vi "main 1.17 beta.vi"() -> ()   [LabVIEW 2015]
uses:
  subvi/PHOIBOS/DEFINITIONS/DEF_dev_state.ctl
  subvi/PHOIBOS/DEFINITIONS/DEF_dev_type.ctl
  <vilib>/Analysis/_algsub.llb/Real Vector Norm.vi
  <vilib>/Analysis/1siggen.llb/Ramp Pattern by Samples.vi
  <vilib>/DAQmx/create/channels.llb/DAQmx Create Channel (DI-Digital Input).vi
  <userlib>/caLab/Private/Put_DBL_PV.vi
  <vilib>/Utility/file.llb/Write Delimited Spreadsheet (string).vi
  <vilib>/Utility/file.llb/Read Delimited Spreadsheet (string).vi
  <vilib>/Utility/file.llb/Write Delimited Spreadsheet (DBL).vi
  <userlib>/caLab/Private/Get_PV.vi
  subvi/Newport ESP301/Newport ESP301.lvlib
  subvi/sp_manip.llb/sp_manip_lib.lvlib
  subvi/sp_manip.llb/tcp_gateway.lvlib
  <vilib>/Analysis/NI_AALBase.lvlib
  <vilib>/Analysis/NI_AALPro.lvlib
  subvi/ZaberTSeries/ZaberTSeries.lvlib
panel:
  out "Pics L":i32=200
  out "Waveform Chart":dbl(graph)
  out "G2 X":cluster{dbl[], "Ramp Pattern":dbl[]}(graph)
  in  "reset every n pics":bool=TRUE
  in  "pics2avg":i32=50
  in  "abort acq.":bool
  out "G2 Y":cluster{dbl[], "Ramp Pattern":dbl[]}(graph)
  out "ETA":timestamp=timestamp(3655133644.4615793 s since 1904-01-01) format="%<%H:%M:%S>T"
  out "acq. imgs":i32=200
  out "snap_prog":dbl(slide)=1.0 scale=0.0..1.0
  in  "BasePath":path=path "X:/trARPES/PESData"
  in  "cam_liveavg":bool=TRUE caption="live average"
  out "cam_fps":dbl=19.774122625512067 caption="FPS" format="%.1g"
  out "sideimg":dbl[][](graph)
  out "RunNumber":u16=3067
  out "sum":dbl format="%#.2g"
  out "max":dbl
  out "mainimg":dbl[][](graph)
  out "ESP_con?":bool=TRUE caption="ESP301"
  out "phoib_con?":bool caption="PHOIBOS"
  out "manip_con?":bool=TRUE caption="manipulator"
  out "cam_con?":bool caption="camera"
  in  "main_close":bool
  in  "Tab Control":enum32{"live", "scan", "devices"}(tab)=enum."devices"
  out "Readback":dbl=304.0
  out "In Range":bool=TRUE
  in  "setpoint_set":bool
  in  "Setpoint":dbl=302.0
  out "TB":dbl=302.67
  out "TA":dbl=303.83
  in  "phoib_I_10s":dbl
  out "phoib_I_10":dbl caption="Mesh Back"
  in  "mirr_go":bool
  in  "ESP_opent0file":bool
  in  "mirr_rel":i32=1 caption="relative [steps]"
  in  "mirr_Y-":bool
  in  "mirr_Y+":bool
  in  "mirr_X+":bool
  in  "mirr_X-":bool
  in  "manip_deltas":dbl[](array[numeric])=[0.0, 0.0, 5.0, 0.0, 0.0, 0.0] caption="delta" format="%#.5g"
  in  "aq.mode":enum32{"Radio Selection 1", "Radio Selection 2"}(radio)=enum."Radio Selection 2"
  in  "dark avg":i32=100
  in  "cam_avgs":i32=200 caption="N"
  in  "ESP_delta":dbl caption="relative [mm]"
  in  "ESP_-":bool
  in  "ESP_+":bool
  in  "ESP_go":bool
  in  "ESP_dest_t":dbl=-1194159.4608093842 caption="[fs]"
  in  "ESP_dest":dbl=-324.0 caption="[mm]"
  in  "ESP_set_t0":bool
  in  "phoib_I_6s":dbl=3200.0
  in  "phoib_I_5s":dbl=1500.0
  in  "phoib_I_4s":dbl=4.558
  in  "phoib_I_3s":dbl=-10.0
  in  "phoib_I_2s":dbl=35.0
  in  "phoib_I_1s":dbl=21.0
  in  "phoib_standby":bool
  in  "phoib_set":bool
  out "phoib_I_6":dbl caption="Screen Voltage"
  out "phoib_I_5":dbl caption="Detctor Voltage"
  out "phoib_I_4":dbl caption="Work Function"
  out "phoib_I_3":dbl caption="Coil Current"
  out "phoib_I_2":dbl caption="Pass Energy"
  out "phoib_I_1":dbl caption="Kinetic Energy"
  out "Saved Positions":string[][](table)=[["ertwertwert", "-2.299945", "-2.030214", "38.900024", "50.000762", "0.000887", "-97.998082"], ["uztgugt", "-14.999451", "-13.638894", "442.380066", "13.998380", "-1.893758", "-76.305838"], ["asdf", "-14.999451", "-13.638894", "442.380066", "13.998380", "-1.893758", "-76.305838"], ["test3", "-14.999451", "-13.638894", "441.380066", "13.998380", "-1.893758", "-76.305838"]]
  in  "Save Pos":bool
  in  "Load":bool
  in  "Delete":bool
  in  "ManipRel +":bool
  in  "ManipRel -":bool
  in  "Move Abs":bool
  in  "stop manip":bool
  in  "dest":dbl[](array[numeric])=[1.794011231344732, -4.007411134769244, 35.099853515625, 337.9843004481455, 2.0, 140.61656469713384] caption="destination" format="%#.5g"
  out "axis":string[](array[string])=["x", "y", "z", "polar", "tilt", "azimut"]
  out "pos":dbl[](array[numeric])=[1.794011231344732, -4.007411134769244, 35.099853515625, 337.9843004481455, 1.998632949125299, 140.61656469713384] caption="position" format="%.5f"
  in  "ana_mode":T1(ring)=enum."WideAngleMode"
  in  "ana_voltrange":enum16{"3.5kV", "1.5kV", "400V", "100V", "10V"}(ring)=enum."400V"
  out "ESP_pos":dbl=-325.0 caption="Position"
  out "ESP_delay":dbl=-1200830.742713347 caption="Delay"
  out "ESP_t0":dbl=-145.0 caption="Time Zero @"
  out "phoib_I_7":dbl caption="Conversion Voltage"
  in  "phoib_I_7s":dbl=-30.0
  in  "phoib_I_8s":dbl=0.0039
  in  "phoib_I_9s":dbl
  out "phoib_I_8":dbl caption="FD1"
  out "phoib_I_9":dbl caption="Mesh Front"
  in  "gain":bool
  in  "cam_exp":u32=50 caption="exposure [ms]"
  in  "binning":u16(ring)=2 items=["X 1", "X 2", "X 4", "X 8"]
  in  "cam_dark?":bool=TRUE caption="subtract dark?"
  in  "cam_dark":bool
  in  "cam_saveimg":bool
  in  "e-size":u8
  in  "lower threshold":i32=50
  in  "count?":bool
  in  "ROI Left":i32=1
  in  "ROI Right":i32=43
  in  "ROI Top":i32=1
  in  "ROI Bottom":i32=33
  out "moving?":bool[](array[boolean])
  out "mirr_posX":i32=60782 caption="X"
  out "mirr_posY":i32=121383 caption="Y"
  in  "mirr_dest":i32[](array[numeric])=[60782, 121383]
  out "waveplate position":dbl format="%.6g"
  out "stage2 position":dbl format="%.6g"
  out "current scan 2":i32=3
  out "scan 1":dbl(slide)=1.0 scale=0.0..1.0
  in  "Tab Control 2":enum32{"setup", "data"}(tab)
  in  "scan_selector 2":T2(tab)=enum."stage2"
  in  "scan_manip_start 2":dbl[](array[numeric])=[1.794011231344732, -4.007411134769244, 35.099853515625, 337.9843004481455, 2.000390761745462, 140.61656469713384] caption="start position" format="%#.5g"
  in  "scan_manip_deltas 2":dbl[](array[numeric])=[0.0, 0.0, 0.0, 0.0, 1.0, 0.0] caption="direction vector\n(gets normalized)" format="%#.5g"
  in  "scan_manip_setstart 2":bool
  in  "scan_mirr_start 2":i32[](array[numeric])=[60782, 121383] caption="scan_mirr_start"
  in  "scan_mirr_deltas 2":i32[](array[numeric])=[1, 0] caption="direction vector\n(gets normalized)"
  in  "scan_mirr_setstart 2":bool
  in  "wait addional  2":dbl caption="s"
  in  "Wait for T 2":bool=TRUE
  in  "scan_volt_parameter 2":string(combo)="Kinetic Energy"
  in  "waypointsD2":string[][](table)=[["302", "1"], ["304", ""], ["", ""]]
  in  "waypointsD1":string[][](table)=[["302", "1"], ["304", ""], ["", ""]]
  in  "load waypoints 1":bool
  in  "meas_iter":i32=1 caption="Iterations"
  in  "scan_selector":T2(tab)=enum."stage2"
  in  "scan_manip_setstart":bool
  in  "scan_manip_start":dbl[](array[numeric])=[1.794011231344732, -4.007411134769244, 35.099853515625, 337.9843004481455, 2.000390761745462, 140.61656469713384] caption="start position" format="%#.5g"
  in  "scan_manip_deltas":dbl[](array[numeric])=[0.0, 0.0, 0.0, 0.0, 1.0, 0.0] caption="direction vector\n(gets normalized)" format="%#.5g"
  in  "scan_mirr_start":i32[](array[numeric])=[60782, 121383]
  in  "scan_mirr_deltas":i32[](array[numeric])=[1, 0] caption="direction vector\n(gets normalized)"
  in  "scan_mirr_setstart":bool
  in  "wait addional":dbl caption="s"
  in  "Wait for T":bool=TRUE
  in  "scan_volt_parameter":string(combo)="Kinetic Energy"
  in  "clear waypoints 1":bool
  in  "load waypoints 2":bool
  in  "clear waypoints 2":bool
  out "intensitygraph":cluster{"Array":dbl[], "Intensity Chart":dbl[]}(graph)={"Array"=[302.0, 303.0, 304.0], "Intensity Chart"=[1937.88, 12704.590000000002, 4640.840000000001]}
  out "energygraph":dbl[][](graph)=[[0.0, 0.0, 0.0, 64.28999999999999, 120.06, 0.0, 0.0, 0.0, 0.0, 0.0, 0.0, 0.0, 0.0, 0.0, 0.0, 0.0, 0.0, 0.0, 0.0, 0.0, 0.0, 0.0, 0.0, 0.0, 0.0, 0.0, 0.0, 0.0, 0.0, 0.0, 0.0, 0.0, 0.0, 0.0, 0.0, 0.0, 0.0, 0.0, 0.0, 0.0, 0.0, 0.0, 0.0, 0.0, 0.0, 0.0, 0.0, 0.0, 0.0, 384.53999999999996, 1103.3799999999999, 448.21000000000004, 0.0, 0.0, 0.0, 0.0, 0.0, 0.0, 0.0, 0.0, 0.0, 0.0, 0.0, 0.0, 0.0, 0.0, 0.0, 0.0, 0.0, 120.82, 0.0, 261.04, 195.1, 253.87, 199.70999999999998, 127.75, 87.50999999999999, 0.0, 52.54, 0.0, 0.0, 51.78, 55.73, 0.0, 0.0, 0.0, 0.0, 0.0, 0.0, 0.0, 0.0, 0.0, 0.0, 0.0, 0.0, 0.0, 0.0, 0.0, 0.0, 0.0, 0.0, 0.0, 0.0, 0.0, 0.0, 0.0, 0.0, 0.0, 0.0, 0.0, 0.0, 0.0, 0.0, 332.90999999999997, 1106.25, 934.74, 0.0, 156.76, 62.65, 0.0, 0.0, 0.0, 0.0, 0.0, 0.0, 54.62, 0.0, 0.0, 0.0, 0.0, 0.0, 0.0, 0.0, 0.0, 0.0, 0.0, 0.0, 0.0, 0.0, 0.0, 0.0, 0.0, 0.0, 0.0, 65.85, 165.75, 0.0, 0.0, 0.0, 0.0, 0.0, 0.0, 0.0, 0.0, 0.0, 0.0, 0.0, 0.0, 0.0, 0.0, 0.0, 0.0, 0.0, 266.63, 591.5, 261.64, 0.0, 391.9, 527.29, 82.87, 123.75, 286.74, 151.72, 0.0, 0.0, 0.0, 0.0, 0.0, 0.0, 0.0, 0.0, 0.0, 0.0, 0.0, 0.0, 0.0, 0.0, 0.0, 0.0, 0.0, 0.0, 0.0, 396.37, 721.0900000000001, 353.5, 83.97999999999999, 104.77000000000001, 0.0, 57.83, 60.98, 182.28, 128.78, 0.0, 0.0, 0.0, 465.25, 624.3399999999999, 348.62, 0.0, 0.0, 0.0, 0.0, 0.0, 0.0, 0.0, 0.0, 0.0, 0.0, 0.0, 0.0, 119.7, 217.91, 120.56, 0.0, 0.0, 0.0, 0.0, 0.0, 0.0, 0.0, 58.89, 0.0, 0.0, 0.0, 202.23999999999998, 149.79000000000002, 0.0, 117.82, 212.51999999999998, 534.74, 421.98, 50.97, 0.0, 0.0, 0.0, 0.0, 362.15999999999997, 656.04, 265.02, 0.0, 0.0, 0.0, 0.0, 0.0, 0.0, 0.0, 0.0, 0.0, 0.0, 0.0, 0.0, 0.0, 0.0, 0.0, 0.0, 0.0, 0.0, 0.0, 0.0, 0.0, 0.0, 0.0, 0.0, 0.0, 0.0, 0.0, 0.0, 0.0, 0.0, 0.0, 0.0, 0.0, 0.0, 0.0, 0.0, 0.0, 0.0, 0.0, 0.0, 0.0, 0.0, 0.0, 0.0, 0.0, 0.0, 0.0, 0.0, 0.0, 0.0, 0.0, 0.0, 0.0, 0.0, 0.0, 0.0, 0.0, 0.0, 0.0, 0.0, 0.0, 0.0, 0.0, 0.0, 237.67999999999998, 286.08, 130.9, 0.0, 0.0, 0.0, 0.0, 0.0, 0.0, 0.0, 0.0, 0.0, 0.0, 0.0, 0.0, 0.0, 0.0, 0.0, 0.0, 0.0, 0.0, 0.0, 0.0, 0.0, 0.0, 0.0, 0.0, 0.0, 0.0, 0.0, 0.0], [0.0, 0.0, 0.0, 0.0, 0.0, 0.0, 0.0, 0.0, 0.0, 0.0, 0.0, 0.0, 0.0, 0.0, 0.0, 0.0, 0.0, 485.13, 1279.2, 234.71, 0.0, 0.0, 0.0, 0.0, 0.0, 0.0, 0.0, 0.0, 0.0, 0.0, 0.0, 0.0, 50.5, 654.4200000000001, 511.98, 0.0, 0.0, 0.0, 0.0, 0.0, 0.0, 0.0, 0.0, 0.0, 0.0, 0.0, 0.0, 0.0, 0.0, 0.0, 0.0, 0.0, 0.0, 0.0, 0.0, 0.0, 0.0, 0.0, 63.72, 693.84, 574.54, 0.0, 0.0, 0.0, 68.68, 1054.28, 1010.9499999999999, 0.0, 0.0, 0.0, 0.0, 0.0, 0.0, 0.0, 0.0, 0.0, 0.0, 0.0, 56.57, 971.76, 1333.73, 330.0, 0.0, 0.0, 0.0, 0.0, 0.0, 349.33000000000004, 292.7, 0.0, 0.0, 0.0, 0.0, 0.0, 0.0, 82.77000000000001, 1059.23, 1069.87, 156.47, 0.0, 0.0, 0.0, 0.0, 293.91, 333.47, 551.4, 493.64, 73.72999999999999, 0.0, 0.0, 0.0, 0.0, 0.0, 0.0, 0.0, 0.0, 0.0, 0.0, 0.0, 0.0, 0.0, 0.0, 286.01, 543.0699999999999, 251.94, 0.0, 0.0, 0.0, 0.0, 0.0, 233.63, 968.4799999999999, 771.53, 109.94, 0.0, 123.07, 499.72999999999996, 431.4, 0.0, 0.0, 60.85, 69.5, 0.0, 0.0, 0.0, 0.0, 0.0, 0.0, 0.0, 0.0, 0.0, 0.0, 0.0, 0.0, 0.0, 0.0, 52.01, 0.0, 0.0, 0.0, 0.0, 0.0, 0.0, 0.0, 0.0, 0.0, 0.0, 0.0, 0.0, 0.0, 0.0, 0.0, 0.0, 0.0, 0.0, 0.0, 0.0, 0.0, 0.0, 0.0, 0.0, 0.0, 0.0, 0.0, 0.0, 0.0, 0.0, 0.0, 0.0, 0.0, 52.95, 478.8, 870.47, 572.83, 61.67, 268.19, 1143.4, 1804.2599999999998, 1145.6100000000001, 739.22, 904.59, 1109.3000000000002, 1233.6599999999999, 212.92, 0.0, 0.0, 105.95, 448.76000000000005, 1306.3500000000001, 1005.5900000000001, 68.8, 0.0, 57.94, 0.0, 0.0, 0.0, 0.0, 0.0, 0.0, 0.0, 0.0, 0.0, 0.0, 0.0, 0.0, 0.0, 0.0, 0.0, 0.0, 0.0, 0.0, 0.0, 0.0, 0.0, 0.0, 0.0, 0.0, 159.01, 520.94, 925.5600000000001, 1641.53, 2261.26, 1259.83, 0.0, 0.0, 0.0, 0.0, 0.0, 0.0, 136.69, 398.81, 382.02, 0.0, 0.0, 0.0, 0.0, 0.0, 0.0, 421.01, 1376.5800000000002, 1425.75, 268.07, 0.0, 345.84000000000003, 396.77, 0.0, 0.0, 0.0, 0.0, 0.0, 216.93, 727.65, 830.9, 774.2299999999999, 839.3900000000001, 309.97, 0.0, 0.0, 0.0, 0.0, 0.0, 0.0, 0.0, 100.57, 459.66, 305.86, 0.0, 0.0, 0.0, 0.0, 0.0, 0.0, 0.0, 0.0, 0.0, 0.0, 0.0, 0.0, 0.0, 0.0, 0.0, 0.0, 0.0, 0.0, 0.0, 0.0, 0.0, 0.0, 0.0, 0.0, 0.0, 64.97999999999999, 379.62, 337.15999999999997, 83.6, 463.66, 399.03999999999996, 0.0, 0.0, 0.0, 0.0, 0.0, 0.0, 0.0, 0.0, 0.0, 0.0, 0.0, 0.0, 0.0, 0.0, 0.0, 0.0, 0.0, 0.0, 0.0, 0.0, 0.0, 0.0, 0.0, 0.0, 0.0, 0.0, 0.0], [0.0, 0.0, 0.0, 0.0, 0.0, 0.0, 0.0, 0.0, 0.0, 0.0, 0.0, 0.0, 0.0, 0.0, 0.0, 165.83, 124.99, 78.27000000000001, 0.0, 0.0, 0.0, 765.77, 1457.88, 293.67, 0.0, 0.0, 0.0, 0.0, 0.0, 0.0, 0.0, 0.0, 0.0, 0.0, 0.0, 0.0, 0.0, 0.0, 0.0, 0.0, 0.0, 0.0, 0.0, 0.0, 0.0, 0.0, 0.0, 0.0, 0.0, 85.5, 116.32, 0.0, 0.0, 0.0, 0.0, 0.0, 0.0, 0.0, 0.0, 0.0, 0.0, 0.0, 0.0, 0.0, 0.0, 0.0, 0.0, 0.0, 179.01, 123.78999999999999, 64.69, 0.0, 433.57000000000005, 1457.15, 661.49, 0.0, 0.0, 0.0, 0.0, 0.0, 0.0, 171.38, 497.28999999999996, 835.47, 1797.0300000000002, 1202.25, 169.95, 0.0, 0.0, 0.0, 0.0, 383.74, 496.08, 196.89999999999998, 0.0, 0.0, 0.0, 0.0, 719.08, 1717.5100000000002, 1360.8, 163.65, 118.56, 798.75, 610.32, 0.0, 0.0, 0.0, 0.0, 73.12, 51.75, 0.0, 0.0, 0.0, 0.0, 0.0, 0.0, 0.0, 0.0, 0.0, 0.0, 0.0, 233.35000000000002, 1128.3, 1138.8400000000001, 207.43, 0.0, 0.0, 50.52, 0.0, 0.0, 0.0, 0.0, 0.0, 0.0, 0.0, 0.0, 0.0, 0.0, 0.0, 0.0, 0.0, 0.0, 0.0, 0.0, 0.0, 0.0, 0.0, 0.0, 0.0, 0.0, 122.82, 66.93, 184.87, 606.35, 1065.2, 616.33, 82.97, 0.0, 0.0, 0.0, 0.0, 0.0, 0.0, 0.0, 0.0, 0.0, 0.0, 0.0, 210.77, 369.49, 0.0, 0.0, 0.0, 0.0, 0.0, 0.0, 0.0, 0.0, 0.0, 0.0, 0.0, 0.0, 0.0, 0.0, 0.0, 0.0, 0.0, 0.0, 61.71, 492.70000000000005, 501.67999999999995, 50.9, 0.0, 0.0, 0.0, 0.0, 0.0, 0.0, 0.0, 0.0, 0.0, 0.0, 0.0, 0.0, 0.0, 0.0, 0.0, 0.0, 0.0, 0.0, 0.0, 0.0, 0.0, 0.0, 0.0, 0.0, 0.0, 0.0, 0.0, 0.0, 0.0, 0.0, 0.0, 0.0, 0.0, 0.0, 0.0, 0.0, 0.0, 0.0, 0.0, 0.0, 0.0, 0.0, 0.0, 0.0, 0.0, 0.0, 0.0, 0.0, 0.0, 0.0, 0.0, 0.0, 0.0, 0.0, 0.0, 0.0, 0.0, 0.0, 0.0, 0.0, 0.0, 0.0, 0.0, 0.0, 0.0, 0.0, 0.0, 0.0, 0.0, 0.0, 0.0, 0.0, 0.0, 0.0, 0.0, 0.0, 0.0, 191.69, 347.02, 262.31, 325.89, 168.79, 0.0, 0.0, 52.9, 53.13, 0.0, 0.0, 0.0, 0.0, 0.0, 0.0, 0.0, 0.0, 0.0, 0.0, 0.0, 0.0, 0.0, 0.0, 0.0, 0.0, 0.0, 0.0, 0.0, 0.0, 0.0, 0.0, 0.0, 0.0, 0.0, 0.0, 327.12, 491.83000000000004, 242.02999999999997, 0.0, 0.0, 0.0, 0.0, 0.0, 0.0, 0.0, 676.6, 975.77, 229.86, 0.0, 144.15, 151.75, 0.0, 0.0, 0.0, 0.0, 0.0, 0.0, 0.0, 0.0, 0.0, 0.0, 0.0, 0.0, 0.0, 0.0, 0.0, 0.0, 0.0, 0.0, 0.0, 0.0, 0.0, 0.0, 0.0]]
  out "anglegraph":dbl[][](graph)=[[0.0, 0.0, 0.0, 0.0, 0.0, 0.0, 0.0, 0.0, 0.0, 0.0, 0.0, 0.0, 0.0, 0.0, 0.0, 0.0, 0.0, 0.0, 0.0, 0.0, 0.0, 0.0, 0.0, 0.0, 0.0, 0.0, 0.0, 307.98, 204.45, 0.0, 0.0, 0.0, 0.0, 0.0, 0.0, 0.0, 0.0, 0.0, 0.0, 0.0, 0.0, 0.0, 0.0, 0.0, 0.0, 0.0, 0.0, 0.0, 0.0, 0.0, 0.0, 0.0, 0.0, 0.0, 0.0, 0.0, 0.0, 0.0, 0.0, 0.0, 0.0, 0.0, 0.0, 0.0, 0.0, 0.0, 0.0, 0.0, 0.0, 0.0, 0.0, 0.0, 0.0, 0.0, 0.0, 0.0, 0.0, 0.0, 0.0, 0.0, 0.0, 0.0, 0.0, 0.0, 0.0, 0.0, 0.0, 0.0, 0.0, 0.0, 0.0, 0.0, 0.0, 0.0, 0.0, 0.0, 0.0, 0.0, 0.0, 0.0, 0.0, 0.0, 0.0, 0.0, 0.0, 0.0, 0.0, 0.0, 0.0, 0.0, 0.0, 0.0, 0.0, 0.0, 0.0, 0.0, 0.0, 0.0, 0.0, 0.0, 0.0, 0.0, 0.0, 0.0, 0.0, 0.0, 0.0, 0.0, 0.0, 0.0, 0.0, 0.0, 0.0, 0.0, 0.0, 0.0, 0.0, 0.0, 0.0, 0.0, 0.0, 0.0, 0.0, 0.0, 0.0, 0.0, 0.0, 0.0, 0.0, 0.0, 0.0, 0.0, 0.0, 0.0, 0.0, 0.0, 640.8800000000001, 550.45, 91.89, 0.0, 0.0, 0.0, 0.0, 0.0, 0.0, 0.0, 0.0, 0.0, 0.0, 0.0, 0.0, 0.0, 0.0, 0.0, 0.0, 69.94, 60.96, 0.0, 0.0, 0.0, 0.0, 0.0, 0.0, 0.0, 0.0, 0.0, 0.0, 0.0, 0.0, 0.0, 0.0, 0.0, 0.0, 0.0, 0.0, 0.0, 115.87, 235.84, 172.04999999999998, 0.0, 0.0, 0.0, 0.0, 0.0, 0.0, 0.0, 0.0, 0.0, 0.0, 0.0, 0.0, 0.0, 0.0, 0.0, 0.0, 0.0, 0.0, 0.0, 0.0, 0.0, 0.0, 0.0, 0.0, 0.0, 0.0, 0.0, 0.0, 0.0, 0.0, 0.0, 0.0, 0.0, 0.0, 0.0, 0.0, 0.0, 0.0, 0.0, 0.0, 0.0, 0.0, 0.0, 0.0, 0.0, 0.0, 0.0, 0.0, 0.0, 0.0, 0.0, 0.0, 0.0, 0.0, 0.0, 0.0, 0.0], [0.0, 0.0, 0.0, 0.0, 0.0, 0.0, 0.0, 0.0, 0.0, 0.0, 0.0, 0.0, 0.0, 0.0, 0.0, 0.0, 54.97, 1426.6399999999999, 1312.94, 180.81, 0.0, 0.0, 0.0, 0.0, 0.0, 0.0, 0.0, 465.48, 989.61, 293.56, 0.0, 0.0, 0.0, 0.0, 0.0, 0.0, 0.0, 0.0, 0.0, 0.0, 0.0, 0.0, 0.0, 0.0, 0.0, 0.0, 0.0, 0.0, 0.0, 0.0, 0.0, 0.0, 0.0, 0.0, 0.0, 0.0, 0.0, 0.0, 0.0, 331.78, 944.91, 463.28, 0.0, 0.0, 0.0, 0.0, 143.70999999999998, 402.81, 196.09, 0.0, 0.0, 0.0, 483.82, 433.7, 0.0, 0.0, 0.0, 0.0, 0.0, 0.0, 89.85, 513.2, 263.03999999999996, 0.0, 0.0, 0.0, 0.0, 0.0, 0.0, 0.0, 0.0, 104.84, 0.0, 226.86, 214.93, 235.13, 0.0, 0.0, 0.0, 0.0, 0.0, 0.0, 0.0, 0.0, 0.0, 0.0, 0.0, 0.0, 0.0, 0.0, 0.0, 0.0, 0.0, 0.0, 0.0, 0.0, 0.0, 0.0, 0.0, 0.0, 0.0, 0.0, 0.0, 0.0, 0.0, 0.0, 0.0, 0.0, 0.0, 0.0, 0.0, 0.0, 0.0, 0.0, 0.0, 0.0, 0.0, 0.0, 0.0, 380.83, 649.96, 229.04, 0.0, 0.0, 0.0, 276.21000000000004, 441.79999999999995, 228.29, 0.0, 0.0, 0.0, 0.0, 0.0, 0.0, 0.0, 0.0, 0.0, 0.0, 0.0, 0.0, 0.0, 0.0, 0.0, 0.0, 0.0, 0.0, 0.0, 0.0, 123.92000000000002, 1311.81, 1454.81, 600.87, 0.0, 0.0, 0.0, 0.0, 0.0, 0.0, 0.0, 0.0, 0.0, 0.0, 0.0, 0.0, 0.0, 0.0, 0.0, 0.0, 0.0, 0.0, 0.0, 0.0, 0.0, 0.0, 0.0, 0.0, 0.0, 0.0, 0.0, 0.0, 0.0, 0.0, 654.53, 894.22, 410.35, 0.0, 0.0, 0.0, 0.0, 0.0, 0.0, 0.0, 0.0, 0.0, 0.0, 0.0, 0.0, 0.0, 0.0, 0.0, 0.0, 0.0, 0.0, 0.0, 0.0, 0.0, 0.0, 0.0, 0.0, 0.0, 0.0, 0.0, 0.0, 0.0, 0.0, 0.0, 0.0, 0.0, 0.0, 0.0, 0.0, 0.0, 0.0, 0.0, 0.0, 0.0, 0.0, 0.0, 0.0, 0.0, 0.0, 0.0, 0.0, 0.0, 0.0, 0.0], [0.0, 0.0, 0.0, 0.0, 0.0, 0.0, 0.0, 0.0, 0.0, 0.0, 0.0, 0.0, 0.0, 0.0, 0.0, 0.0, 0.0, 0.0, 0.0, 0.0, 0.0, 0.0, 0.0, 0.0, 0.0, 0.0, 0.0, 0.0, 0.0, 125.9, 1017.51, 504.48, 0.0, 0.0, 0.0, 0.0, 0.0, 0.0, 0.0, 0.0, 0.0, 0.0, 0.0, 0.0, 0.0, 0.0, 0.0, 0.0, 0.0, 0.0, 0.0, 0.0, 0.0, 0.0, 0.0, 0.0, 0.0, 0.0, 0.0, 0.0, 0.0, 0.0, 0.0, 0.0, 0.0, 0.0, 0.0, 0.0, 0.0, 0.0, 0.0, 0.0, 109.81, 66.88, 0.0, 0.0, 733.48, 806.32, 342.43, 0.0, 0.0, 0.0, 0.0, 0.0, 0.0, 0.0, 0.0, 0.0, 0.0, 0.0, 0.0, 0.0, 0.0, 0.0, 0.0, 0.0, 0.0, 0.0, 0.0, 0.0, 0.0, 0.0, 0.0, 0.0, 0.0, 174.07999999999998, 275.74, 429.21, 301.15999999999997, 0.0, 0.0, 0.0, 0.0, 0.0, 0.0, 0.0, 0.0, 0.0, 0.0, 0.0, 0.0, 0.0, 0.0, 0.0, 0.0, 0.0, 0.0, 0.0, 0.0, 0.0, 0.0, 0.0, 0.0, 0.0, 0.0, 0.0, 0.0, 0.0, 0.0, 0.0, 0.0, 0.0, 0.0, 0.0, 0.0, 0.0, 0.0, 0.0, 0.0, 0.0, 0.0, 0.0, 0.0, 0.0, 0.0, 0.0, 0.0, 0.0, 0.0, 0.0, 0.0, 0.0, 0.0, 0.0, 0.0, 0.0, 0.0, 0.0, 0.0, 0.0, 0.0, 0.0, 0.0, 0.0, 0.0, 252.98000000000002, 303.56, 60.91, 52.9, 53.13, 0.0, 0.0, 0.0, 0.0, 0.0, 0.0, 0.0, 0.0, 0.0, 0.0, 0.0, 0.0, 0.0, 0.0, 0.0, 0.0, 0.0, 0.0, 0.0, 0.0, 0.0, 0.0, 0.0, 0.0, 0.0, 0.0, 0.0, 0.0, 0.0, 0.0, 0.0, 0.0, 0.0, 61.05, 350.49, 266.71000000000004, 0.0, 0.0, 0.0, 0.0, 0.0, 0.0, 0.0, 0.0, 0.0, 0.0, 0.0, 0.0, 0.0, 0.0, 0.0, 0.0, 0.0, 0.0, 0.0, 0.0, 0.0, 0.0, 0.0, 0.0, 0.0, 0.0, 0.0, 0.0, 0.0, 0.0, 0.0, 0.0, 0.0, 0.0, 0.0, 0.0, 0.0, 0.0, 0.0, 0.0]]
  in  "stop after iteration":bool
  in  "time/step [s]":dbl=10.787117004394531
  out "current iteration":i32=1
  out "current scan":i32=3
  out "iteration":dbl(slide)=1.0 scale=0.0..1.0
  out "scan 2":dbl(slide)=1.0 scale=0.0..1.0
  in  "stop after step":bool
  in  "scan_go":bool
  out "measpoints":i32=3
  out "total steps":i32=3
  out "RAM [MB]":dbl=1.6590000000000003
  out "disk [MB]":dbl=1.6590000000000003
  out "duration [HH:MM:SS]":dbl=32.361351013183594 format="%<%H:%M:%S>t"
  out "ETA 2":timestamp
  in  "ESP patch":i32[](array[numeric])=[3, 2, 1]
  in  "LS310  EPICS Heater":string="trARPES:Carving:HT-RNG"
  in  "LS310  EPICS SP":string="trARPES:Carving:TEMP"
  in  "LS310  EPICS chanel B":string="trARPES:Carving:TEMP-B"
  in  "mm/s":dbl
  in  "Set Speed to":bool
  in  "ESP Axis waveplate":i32=2 min=1 max=3
  in  "mirr_init":bool
  in  "mirr_release":bool
  in  "mirr_Y#":u8=2
  in  "manip_init":bool
  in  "manip_release":bool
  in  "phoib_init":bool
  in  "phoib_release":bool
  in  "ESP_init":bool
  in  "ESP_release":bool
  in  "ESP301 VISA":refnum<visa-resource-name>="COM4"
  in  "board number":i32
  in  "cam_init":bool
  in  "cam_release":bool
  out "cam_error":errorcluster
  out "phoib_error":errorcluster
  out "state":T3 items=["Off"=-1, "Standby"=0, "On"=1]
  in  "ESP Axis delay":i32=3 min=1 max=3
  out "error out":errorcluster={"status"=FALSE, "code"=1073676418, "source"="VISA Close in Newport ESP301.lvlib:Close.vi->main 1.16 testing LR.vi"}
  out "error out 2":errorcluster={"status"=TRUE, "code"=1, "source"="TCP Write in sp_manip_lib.lvlib:sp_manip_disconnect.vi->main 1.16 testing LR.vi"}
  out "mirr_Error":errorcluster={"status"=FALSE, "code"=1073676418, "source"="VISA Close in ZaberTSeries.lvlib:Close.vi->main 1.16 testing LR.vi"}
  in  "mirr_VISA":refnum<visa-resource-name>="COM7"
  in  "mirr_X#":u8=1
  in  "Operating mode\nHP & QE / HS & DiCam Pro":u32=1
  in  "Frame trigger \n(High Performance and QE only)":u16
  in  "LS310  EPICS chanel A":string="trARPES:Carving:TEMP_RBV"
  in  "Status EPICS chanel":string="trARPES:Carving:TEMP-STAT"
  # "camera"
  # "analyzer"
  # "manipulator"
  # "temperature"
  # "aquisition"
  # "delay stage"
  # "mirror"
  # "Position"
  # "Destination"
  # "- no settings -"
  # "waypoints are absolute values"
  # "- no settings -"
  # "waypoints are absolute values"
  # "- no settings -"
  # "waypoints are absolute values"
  # "X\nY\nZ\npolar\ntilt\nazimut"
  # "waypoint \"0\" is start position"
  # "X\nY"
  # "waypoint \"0\" is start position"
  # "waypoints are absolute values"
  # "- no settings -"
  # "waypoints are absolute values"
  # "- no settings -"
  # "waypoints are absolute values"
  # "- no settings -"
  # "waypoints are absolute values"
  # "X\nY\nZ\npolar\ntilt\nazimut"
  # "waypoint \"0\" is start position"
  # "X\nY"
  # "waypoint \"0\" is start position"
  # "waypoints are absolute values"
  # "camera"
  # "phoibos"
  # "ESP301"
  # "manipulator"
  # "mirror"
  # "delay"
  # "waveplate"
  # "stage2"
  # "0 = sequential\n1 = simultaneous"
  # "0 = internal\n1 = external rising\n2 = external falling"
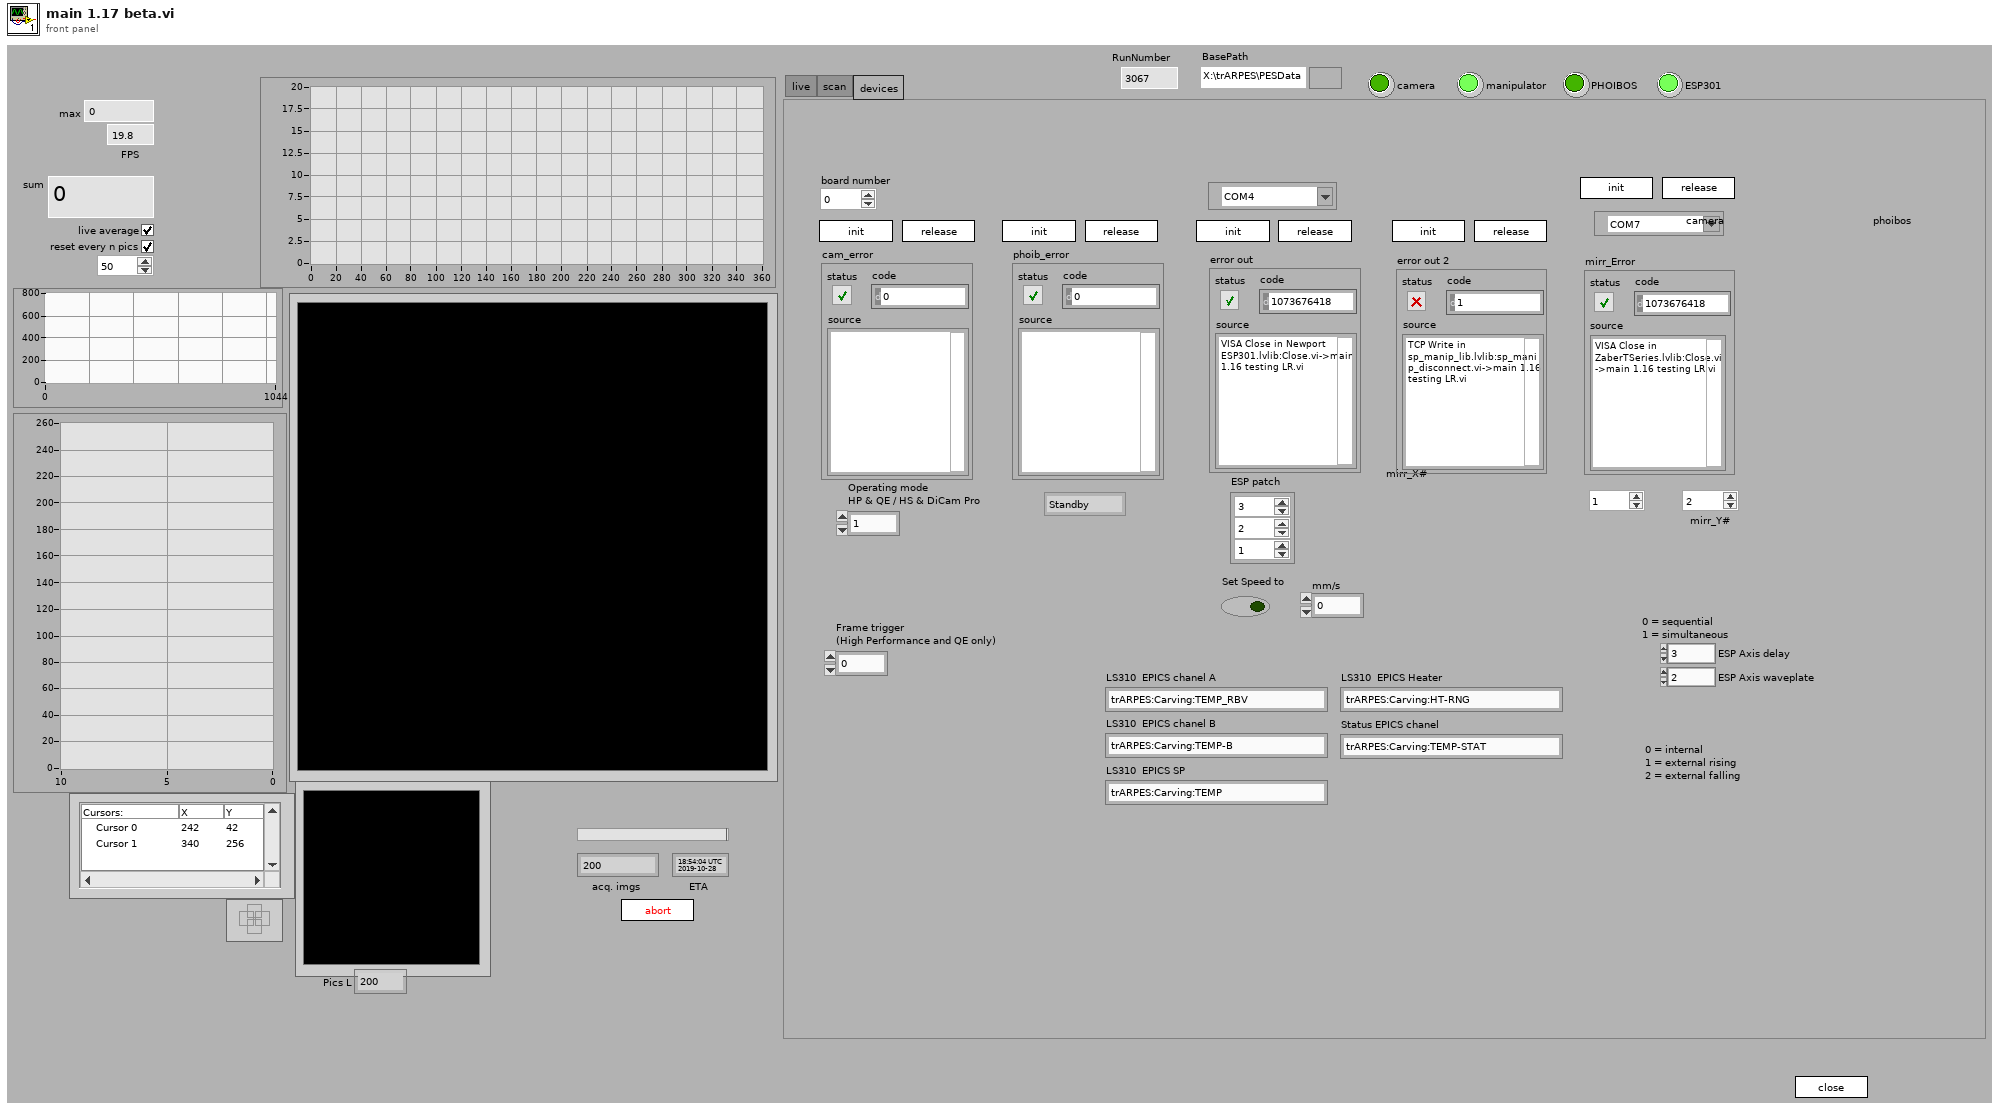
[diagram p1: front panel]
types:
  T1 = enum16{"HighMagnification", "MediumMagnification", "LowMagnification", "HighAngularDispersion", "MediumAngularDispersion", "LowAngularDispersion", "WideAngleMode", "LargeArea", "MediumArea", "SmallArea", "HighMagnification2", "SmallArea2"}
  T2 = enum32{"none", "delay", "waveplate", "stage2", "manipulator", "mirror", "temperature", "voltage"}
  T3 = typedef "DEF_dev_state.ctl" = i32
  T4 = cluster{"queue out":refnum<queue>, "queue out":refnum<queue>, "queue out":refnum<queue>, "queue out":refnum<queue>, "queue out":refnum<queue>, "queue out":refnum<queue>}
  T5 = typedef "LVCursorListTypeDef.ctl" = cluster{"Name":string, "Color":u32, "Style":u8, "Point Style":u8, "Name Visible":bool, "Allow Drag":bool, "Cursor Mode":u32, "Plot":i32, "Index":i32, "Position":cluster{"X":dbl, "Y":dbl}, "X Scale":u32, "Y Scale":u32, "Watch Plots":i32[], "Watch All Plots":bool, "Plot Area":i32, "Label Offset":cluster{"X":dbl, "Y":dbl}}[]
  T6 = cluster{"mirr_X#":u8, "Command":u8, dbl, "Response Count":i32}
  T7 = cluster{"mirr_Y#":u8, "Command":u8, dbl, "Response Count":i32}
  T8 = cluster{i32, "Command":u8, i32, "Response Count":i32}
  T9 = cluster{"Axis_Name":string, "Axis_Type":string, "Axis_Position":dbl, "continous":bool, "moving":bool}[]
  T10 = typedef "DEF_dev_type.ctl" = enum32{"devA (analyzer)", "devD (detector)"}
  T11 = cluster{"Camera type":u32, "Operating mode\nHP & QE / HS & DiCam Pro ":u32, "Frame trigger \n(High Performance and QE only)":u16, "Sequence trigger":u16, "Low Light\n(QE only)":bool, "Gain":bool, "Horzontal\nbinning":u16, "Vertical\nbinning ":u16, "ROI Left":i32, "ROI Right":i32, "ROI Top":i32, "ROI Bottom":i32}
  T12 = cluster{"Name":string, "Color":u32, "Style":u8, "Point Style":u8, "Name Visible":bool, "Allow Drag":bool, "Cursor Mode":u32, "Plot":i32, "Index":i32, "Position":cluster{"X":dbl, "Y":dbl}, "X Scale":u32, "Y Scale":u32, "Watch Plots":i32[], "Watch All Plots":bool, "Plot Area":i32, "Label Offset":cluster{"X":dbl, "Y":dbl}}
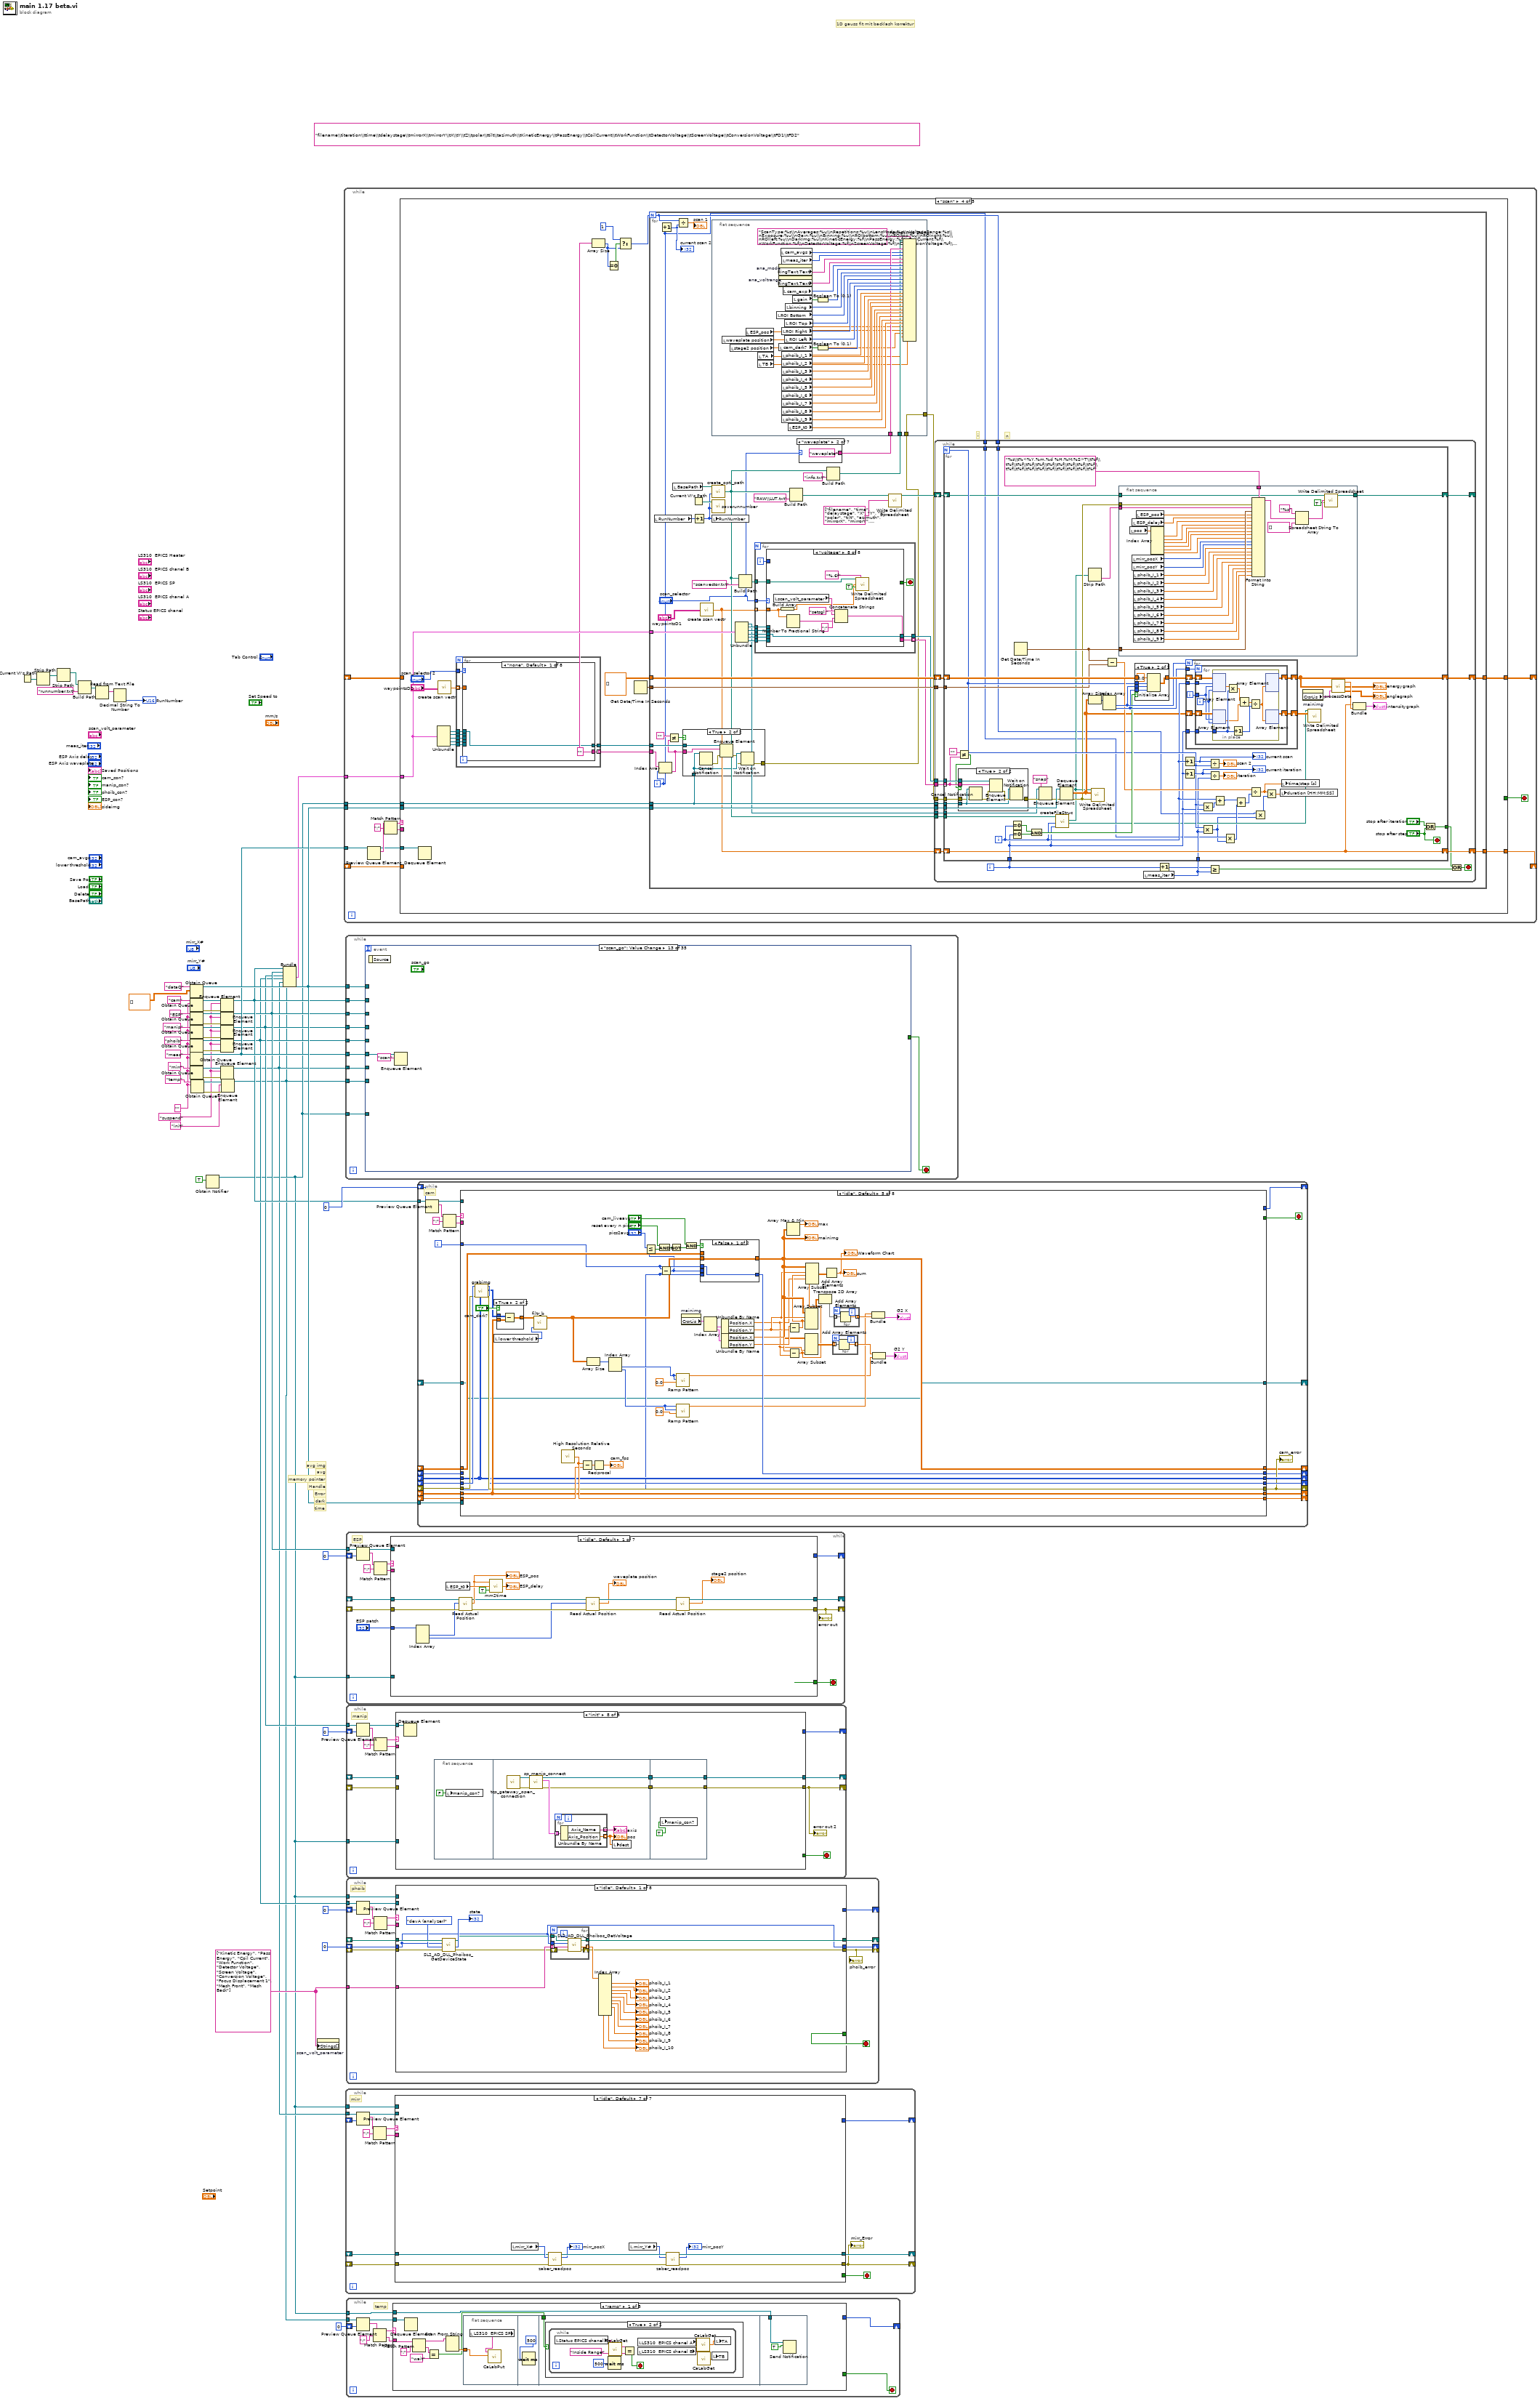
[diagram p0: block diagram]
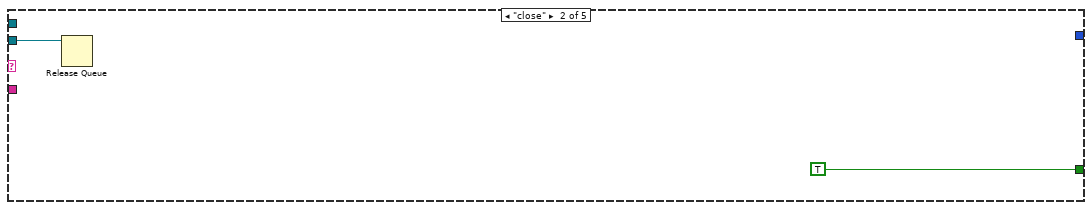
[diagram p3: hidden frame]
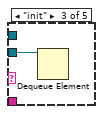
[diagram p4: hidden frame]
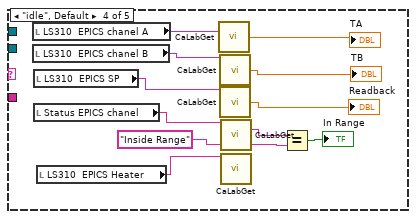
[diagram p5: hidden frame]
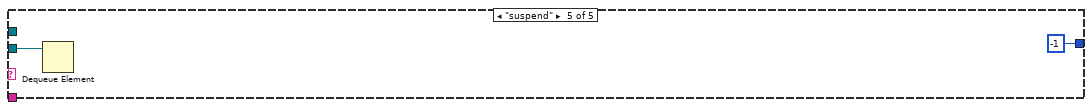
[diagram p6: hidden frame]
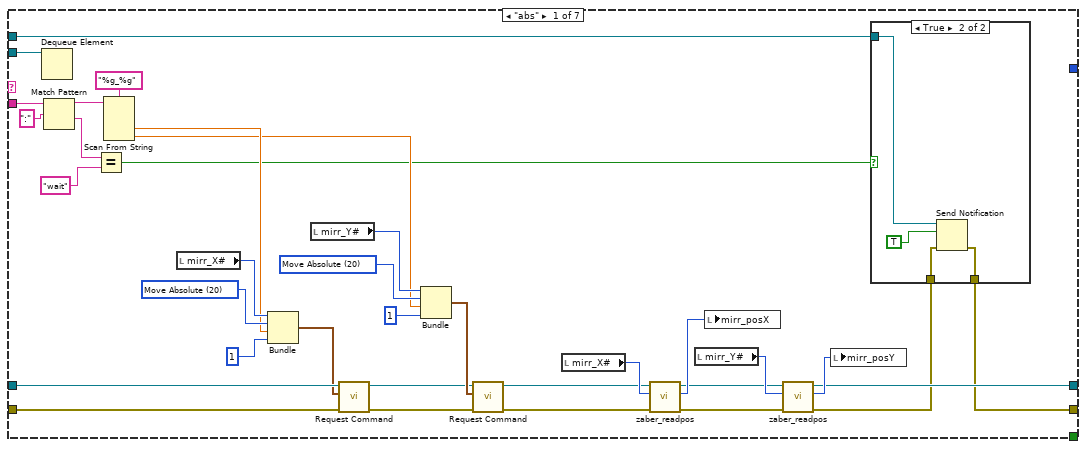
[diagram p7: hidden frame]
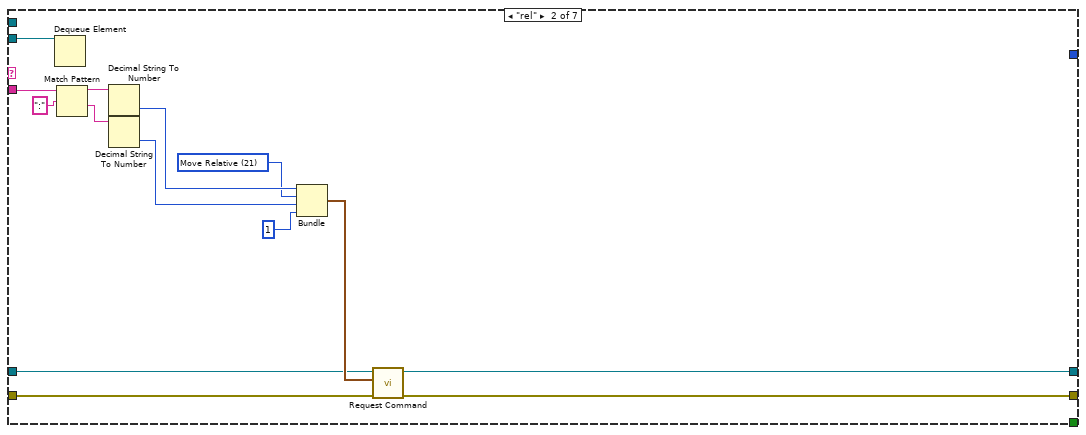
[diagram p9: hidden frame]
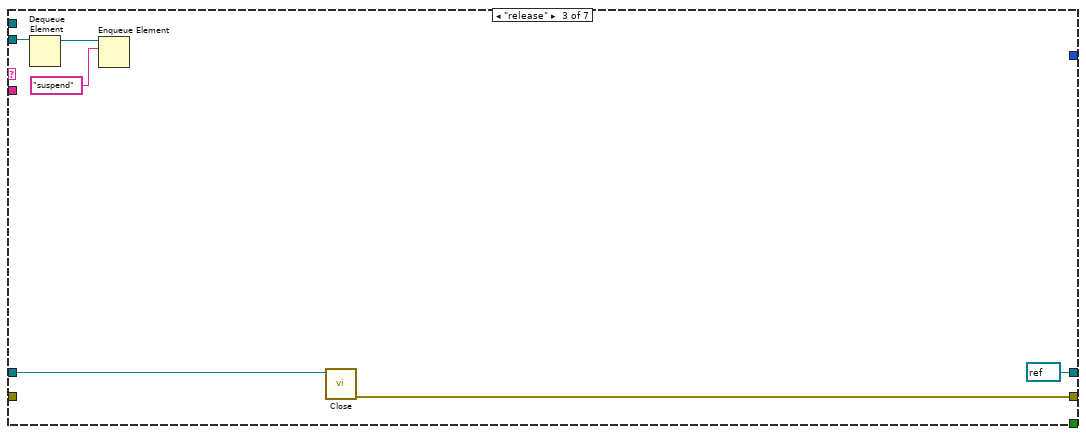
[diagram p10: hidden frame]
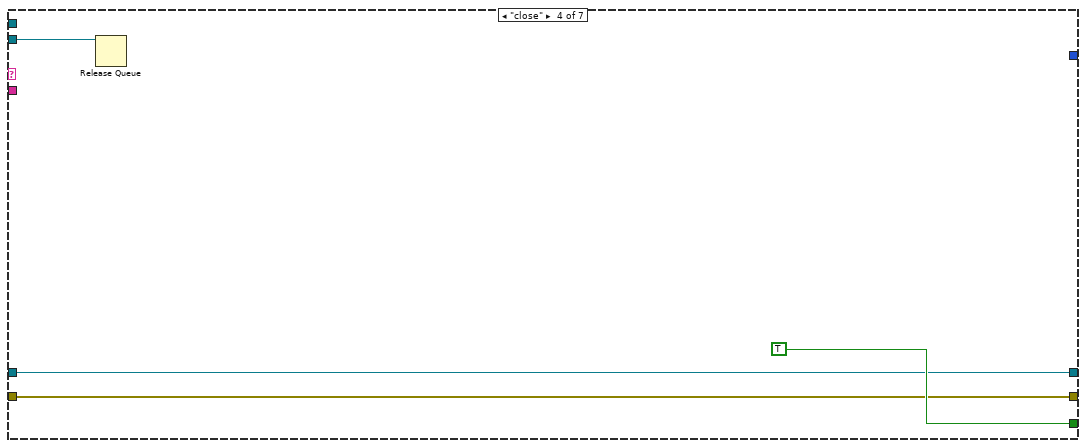
[diagram p11: hidden frame]
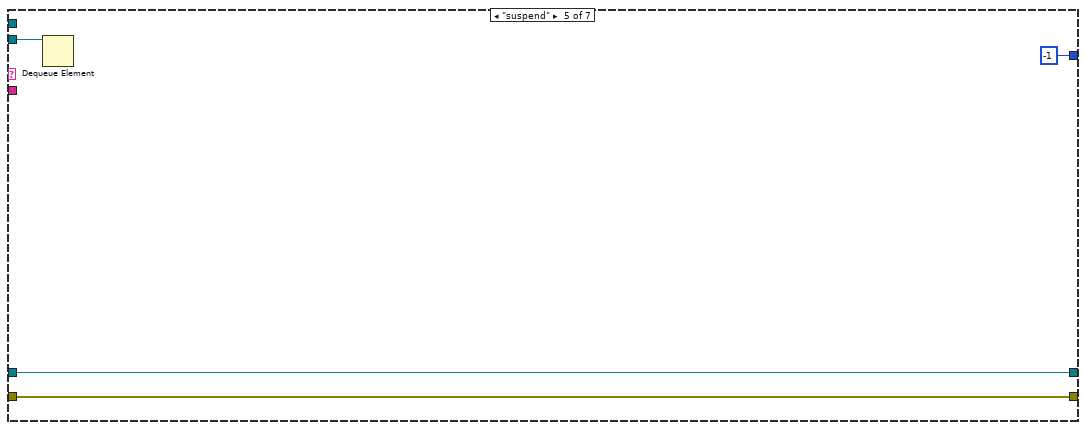
[diagram p12: hidden frame]
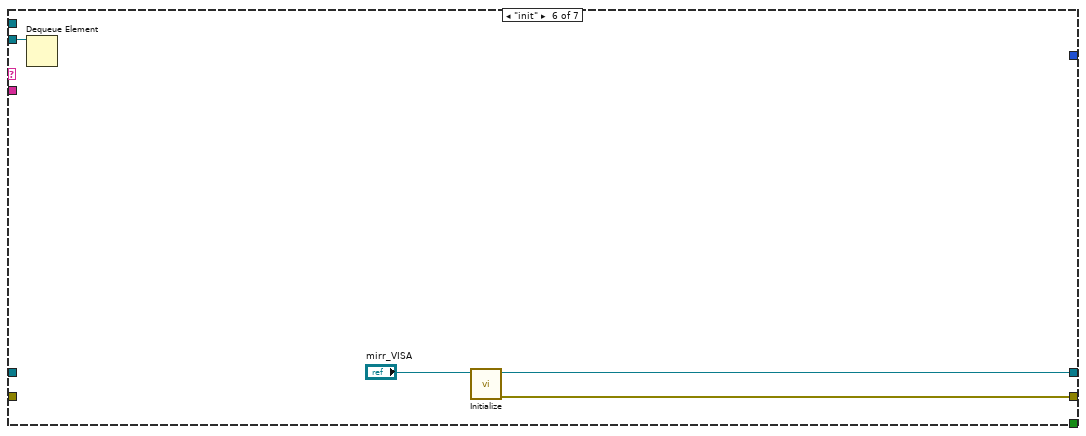
[diagram p13: hidden frame]
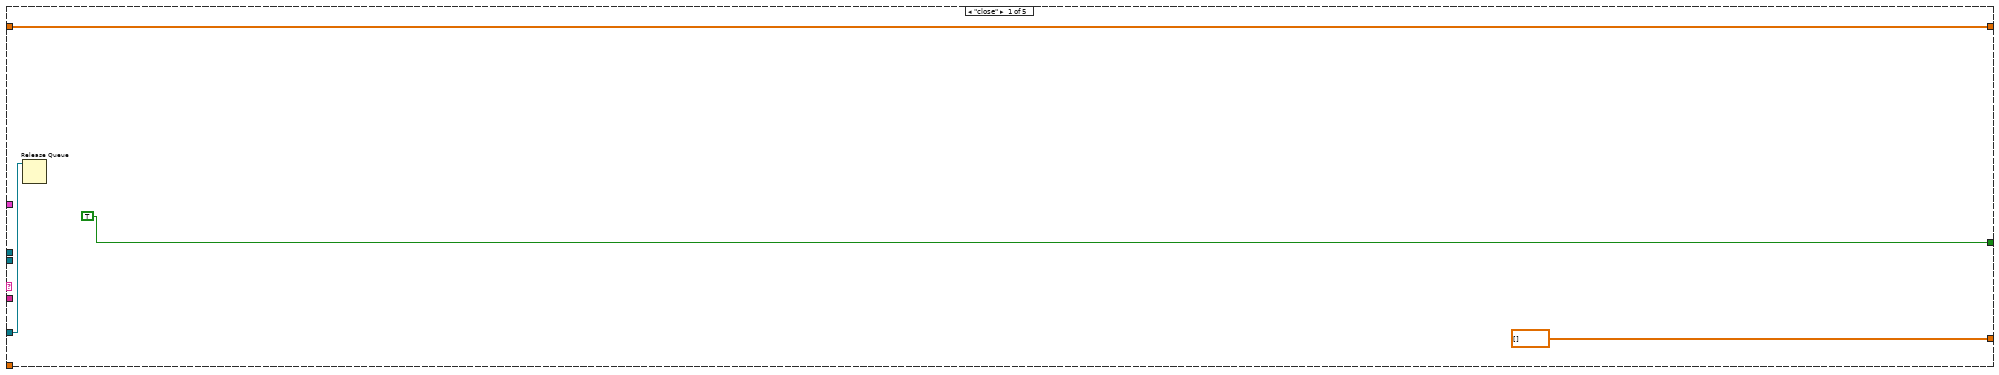
[diagram p14: hidden frame]
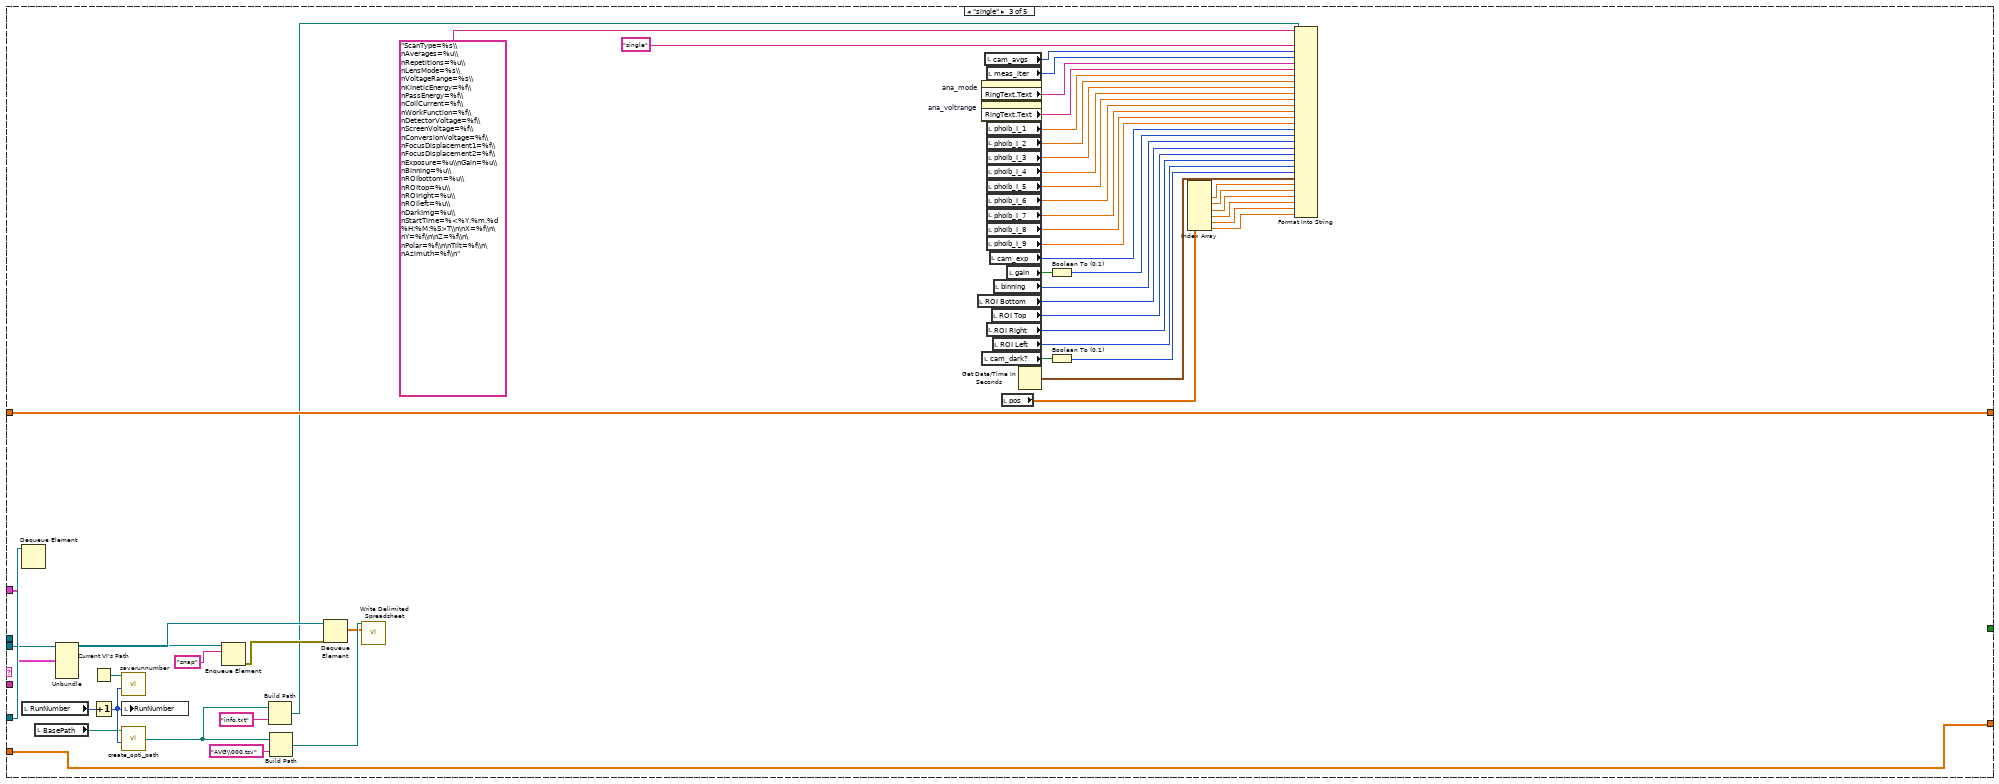
[diagram p16: hidden frame]
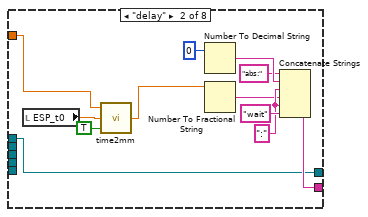
[diagram p17: hidden frame]
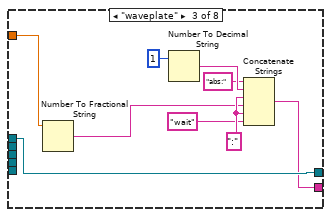
[diagram p18: hidden frame]
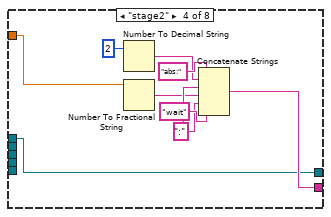
[diagram p19: hidden frame]
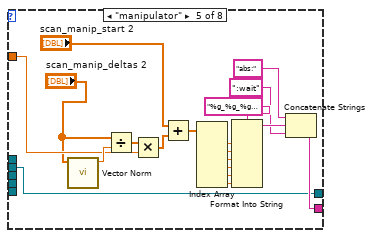
[diagram p20: hidden frame]
diagram:
  (unwired) "filename\\titeration\\ttime\\tdelaystage\\tmirrorX\\tmirrorY\\tX\\tY\\tZ\\tpolar\\ttilt\\tazimuth\\tKineticEnergy\\tPassEnergy\\tCoilCurrent\\tWorkFunction\\tDetectorVoltage\\tScreenVoltage\\tConversionVoltage\\tFD1\\tFD2"
  w15 = string[] ["Kinetic Energy", "Pass Energy", "Coil Current", "Work Function", "Detector Voltage", "Screen Voltage", "Conversion Voltage", "Focus Displacement 1", "Mesh Front", "Mesh Back"]
  w3 = "suspend" ("name (unnamed)")
  w8 = "" ("name (unnamed)")
  # "1D gauss fit mit backlash korrektur"
  # "avg img"
  # "avg"
  # "time"
  # "dark"
  # "Error"
  # "Handle"
  # "memory pointer"
  n1 = Current VI's Path() -> (path=w23:path)
  n2 = Strip Path(path=w23) -> (stripped path=w27:path)  [unwired: 1 out]
  n3 = Strip Path(path=w27) -> (stripped path=w28:path)  [unwired: 1 out]
  n4 = Build Path(base path=w28, name or relative path="runnumber.txt") -> (appended path=w25:path)
  n5 = Read from Text File(file (use dialog)=w25) -> (text=w26:string)  [unwired: 3 in, 3 out]
  n6 = Decimal String To Number(string=w26) -> (number=→"RunNumber":i32)  [unwired: 2 in, 1 out]
  n7 = Obtain Queue(name (unnamed)="dataQ", element data type=dbl[][] []) -> (queue out=w29:refnum<queue>)  [unwired: 3 in, 2 out]
  n8 = Obtain Queue(name (unnamed)="cam", element data type=w8) -> (queue out=w48:refnum<queue>, error out=w47:errorcluster)  [unwired: 3 in, 1 out]
  n9 = Obtain Queue(name (unnamed)="ESP", element data type=w8) -> (queue out=w45:refnum<queue>, error out=w46:errorcluster)  [unwired: 3 in, 1 out]
  n10 = Obtain Queue(name (unnamed)="manip", element data type=w8) -> (queue out=w42:refnum<queue>, error out=w41:errorcluster)  [unwired: 3 in, 1 out]
  n11 = Obtain Queue(name (unnamed)="phoib", element data type=w8) -> (queue out=w39:refnum<queue>, error out=w40:errorcluster)  [unwired: 3 in, 1 out]
  n12 = Obtain Queue(name (unnamed)="meas", element data type=w8) -> (queue out=w22:refnum<queue>)  [unwired: 3 in, 2 out]
  n13 = Obtain Queue(name (unnamed)="mirr", element data type=w8) -> (queue out=w13:refnum<queue>, error out=w12:errorcluster)  [unwired: 3 in, 1 out]
  n14 = Obtain Queue(name (unnamed)="temp", element data type=w8) -> (queue out=w7:refnum<queue>, error out=w6:errorcluster)  [unwired: 3 in, 1 out]
  n15 = Obtain Notifier(notification data type=TRUE) -> (notifier out=w5:refnum<notifier>)  [unwired: 3 in, 2 out]
  n16 = Enqueue Element(queue=w48, element=w3, error in (no error)=w47) -> (queue out=w20:refnum<queue>)  [unwired: 1 in, 2 out]
  n17 = Enqueue Element(queue=w45, element=w3, error in (no error)=w46) -> (queue out=w19:refnum<queue>)  [unwired: 1 in, 2 out]
  n18 = Enqueue Element(queue=w42, element=w3, error in (no error)=w41) -> (queue out=w18:refnum<queue>)  [unwired: 1 in, 2 out]
  n19 = Enqueue Element(queue=w39, element=w3, error in (no error)=w40) -> (queue out=w17:refnum<queue>)  [unwired: 1 in, 2 out]
  n20 = Enqueue Element(queue=w13, element=w3, error in (no error)=w12) -> (queue out=w10:refnum<queue>)  [unwired: 1 in, 2 out]
  n21 = Enqueue Element(queue=w7, element="init" ("name (unnamed)"), error in (no error)=w6) -> (queue out=w1:refnum<queue>)  [unwired: 1 in, 2 out]
  n22 = Bundle("queue out"=w20, "queue out"=w19, "queue out"=w18, "queue out"=w17, "queue out"=w10, "queue out"=w1) -> (w21:T4)  [unwired: 1 in]
  n23 = property on="scan_volt_parameter" class="CmbBox"("Strings[]"=w15) -> ()  [unwired: 2 in, 2 out]
  n24 = while {
    tunnel: w29 -> [w63]
    tunnel: w22 -> [w60]
    tunnel: w21 -> [w56]
    shift-right: [w54] -> _
    shift-left: _ -> [w53]
    tunnel: w5 -> [w52]
    shift-right: [w51] -> _
    shift-left: _ -> [w50]
    stop <- w55 stop-if-true
    n25 = Preview Queue Element(queue=w60) -> (queue out=w57:refnum<queue>, element=w62:string)  [unwired: 2 in, 2 out]
    n26 = Match Pattern(string=w62, regular expression=":") -> (before substring=w59:string, after substring=w58:string)  [unwired: 1 in, 2 out]
    n27 = case shown="\"scan\"" w59 {
      tunnel: w63 -> [_ _ w119 w142 _]
      tunnel: w58 -> [_ _ _ _ _]
      tunnel: w57 -> [w67 _ w120 w138 w601]
      tunnel: [TRUE _ _ _ _] -> w55
      tunnel: w56 -> [_ _ w107 w135 _]
      tunnel: [w65 w69 w105 w140 w607] -> w54
      tunnel: w53 -> [w65 w69 w105 _ w607]
      tunnel: w52 -> [_ _ _ w139 _]
      tunnel: [dbl[] [] ("Array") w68 w77 w136 w603] -> w51
      tunnel: w50 -> [_ w68 w77 _ w603]
      frame "close" {
        n28 = Release Queue(queue=w67) -> ()  [unwired: 2 in, 3 out]
      }
      frame "idle", Default {
      }
      frame "single" {
        n29 = Dequeue Element(queue=w120) -> ()  [unwired: 2 in, 4 out]
        n30 = local read "RunNumber"() -> (w114:u16)
        n31 = local read "BasePath"() -> (w115:path)
        n32 = Unbundle(w107) -> ("queue out"=w106:refnum<queue>)  [unwired: 5 out]
        n33 = Increment(x=w114) -> (x+1=w116:u16)
        n34 = Current VI's Path() -> (path=w113:path)
        n35 = call "saverunnumber.vi"("RunNumber"=w116, "VI path"=w113) -> ()  [unwired: 10 in]
        n36 = local write "RunNumber"(w116) -> ()
        n37 = call "create_opti_path.vi"("RunNumber"=w116, "base path"=w115) -> ("Path"=w109:path)  [unwired: 2 in]
        n38 = Enqueue Element(queue=w106, element="snap" ("string")) -> (error out=w117:errorcluster)  [unwired: 2 in, 2 out]
        n39 = Build Path(base path=w109, name or relative path="info.txt") -> (appended path=w78:path)
        n40 = Build Path(base path=w109, name or relative path="AVG\\000.tsv") -> (appended path=w111:path)
        n41 = Dequeue Element(queue=w119, error in (no error)=w117) -> (element=w108:dbl[][])  [unwired: 1 in, 3 out]
        n42 = call-poly <vilib>:"Write Delimited Spreadsheet.vi"("file path (dialog if empty)"=w111, "2D data"=w108) -> ()  [unwired: 12 in, 2 out]
        n43 = local read "ROI Bottom"() -> (w85:i32)
        n44 = property on="ana_mode" class="Enum (strict)"() -> ("RingText.Text"=w100:string)  [unwired: 2 in, 2 out]
        n45 = property on="ana_voltrange" class="Enum (strict)"() -> ("RingText.Text"=w99:string)  [unwired: 2 in, 2 out]
        n46 = local read "cam_dark?"() -> (w81:bool)
        n47 = local read "cam_avgs"() -> (w102:i32)
        n48 = local read "meas_iter"() -> (w101:i32)
        n49 = local read "phoib_I_1"() -> (w98:dbl)
        n50 = local read "phoib_I_2"() -> (w97:dbl)
        n51 = local read "phoib_I_3"() -> (w96:dbl)
        n52 = local read "phoib_I_4"() -> (w95:dbl)
        n53 = local read "phoib_I_5"() -> (w94:dbl)
        n54 = local read "phoib_I_6"() -> (w93:dbl)
        n55 = local read "phoib_I_7"() -> (w92:dbl)
        n56 = local read "phoib_I_8"() -> (w91:dbl)
        n57 = local read "phoib_I_9"() -> (w90:dbl)
        n58 = local read "ROI Right"() -> (w83:i32)
        n59 = local read "cam_exp"() -> (w89:u32)
        n60 = local read "ROI Top"() -> (w84:i32)
        n61 = local read "ROI Left"() -> (w82:i32)
        n62 = local read "binning"() -> (w86:u16)
        n63 = local read "pos"() -> (w76:dbl[])
        n64 = local read "gain"() -> (w88:bool)
        n65 = Get Date/Time In Seconds() -> (seconds since 1Jan1904=w79:timestamp)
        n66 = Boolean To (0,1)(Boolean=w88) -> (0, 1=w87:i16)
        n67 = Boolean To (0,1)(Boolean=w81) -> (0, 1=w80:i16)
        n68 = Index Array(array=w76) -> (element #1=w75:dbl, element #2=w74:dbl, element #3=w73:dbl, element #4=w72:dbl, element #5=w71:dbl, element #6=w70:dbl)  [unwired: 6 in]
        n69 = Format Into String(format string="ScanType=%s\\nAverages=%u\\nRepetitions=%u\\nLensMode=%s\\nVoltageRange=%s\\nKineticEnergy=%f\\nPassEnergy=%f\\nCoilCurrent=%f\\nWorkFunction=%f\\nDetectorVoltage=%f\\nScreenVoltage=%f\\nConversionVoltage=%f\\nFocusDisplacement1=%f\\nFocusDisplacement2=%f\\nExposure=%u\\nGain=%u\\nBinning=%u\\nROIbottom=%u\\nROItop=%u\\nROIright=%u\\nROIleft=%u\\nDarkImg=%u\\nStartTime=%<%Y.%m.%d %H:%M:%S>T\\n\nX=%f\\n\nY=%f\\n\nZ=%f\\n\nPolar=%f\\n\nTilt=%f\\n\nAzimuth=%f\\n", initial string=w78, "single" ("input 1"), w102, w101, w100, w99, w98, w97, w96, w95, w94, w93, w92, w91, w90, w89, w87, w86, w85, w84, w83, w82, w80, w79, w75, w74, w73, w72, w71, w70) -> ()  [unwired: 1 in, 2 out]
      }
      frame "scan" {
        n70 = Dequeue Element(queue=w138) -> ()  [unwired: 2 in, 4 out]
        n71 = Unbundle(w135) -> ("queue out"=w134:refnum<queue>, "queue out"=w133:refnum<queue>, "queue out"=w132:refnum<queue>, "queue out"=w131:refnum<queue>, "queue out"=w130:refnum<queue>)  [unwired: 1 out]
        n72 = call "create scan vectr.vi"("Table Control"="waypointsD2") -> ("Array"=w128:dbl[])
        n73 = for {
          tunnel: "scan_selector 2" -> [w151]
          tunnel: w134 -> [w150]
          tunnel: w133 -> [w149]
          tunnel: w132 -> [w148]
          tunnel: w131 -> [w147]
          tunnel: w130 -> [w146]
          tunnel: [w145] -> w125 mode=indexing
          tunnel: [w144] -> w129
          tunnel: w128 -> [w143] mode=indexing
          n74 = case shown="\"none\", Default" w151 {
            tunnel: ["" w155 w166 w176 w187 w205 w219 w231] -> w145
            tunnel: w150 -> [w152 w154 w168 w175 _ _ _ _]
            tunnel: w149 -> [_ _ _ _ w186 _ _ _]
            tunnel: w148 -> [_ _ _ _ _ _ _ w230]
            tunnel: w147 -> [_ _ _ _ _ w204 _ _]
            tunnel: w146 -> [_ _ _ _ _ _ w218 _]
            tunnel: [w152 w154 w168 w175 w186 w204 w218 w230] -> w144
            tunnel: w143 -> [_ w156 w167 w177 w188 w203 w221 w232]
            frame "none", Default {
            }
            frame "delay" {
              w159 = ":" ("string")
              n75 = local read "ESP_t0"() -> (w163:dbl)
              n76 = call "time2mm.vi"("fs[1]/ps[0]"=TRUE, "Offset (mm)"=w163, "time"=w156) -> ("position (mm)"=w164:dbl)
              n77 = Number To Decimal String(number=0) -> (decimal integer string=w161:string)  [unwired: 1 in]
              n78 = Number To Fractional String(number=w164) -> (F-format string=w157:string)  [unwired: 3 in]
              n79 = Concatenate Strings("abs:" ("string"), w161, w159, w157, w159, "wait" ("string")) -> (w155:string)
            }
            frame "waveplate" {
              w174 = ":" ("string")
              n80 = Number To Fractional String(number=w167) -> (F-format string=w169:string)  [unwired: 3 in]
              n81 = Number To Decimal String(number=1) -> (decimal integer string=w172:string)  [unwired: 1 in]
              n82 = Concatenate Strings("abs:" ("string"), w172, w174, w169, w174, "wait" ("string")) -> (w166:string)
            }
            frame "stage2" {
              w182 = ":" ("string")
              n83 = Number To Decimal String(number=2) -> (decimal integer string=w179:string)  [unwired: 1 in]
              n84 = Number To Fractional String(number=w177) -> (F-format string=w178:string)  [unwired: 3 in]
              n85 = Concatenate Strings("abs:" ("string"), w179, w182, w178, w182, "wait" ("string")) -> (w176:string)
            }
            frame "manipulator" {
              n86 = call-poly <vilib>:"Vector Norm.vi"("Input Vector"="scan_manip_deltas 2") -> ("norm"=w189:dbl)  [unwired: 9 in, 1 out]
              n87 = Divide(x="scan_manip_deltas 2", y=w189) -> (x/y=w190:dbl[])
              n88 = Multiply(x=w190, y=w188) -> (x*y=w201:dbl[])
              n89 = Add(x="scan_manip_start 2", y=w201) -> (x+y=w202:dbl[])
              n90 = Index Array(array=w202) -> (element #1=w199:dbl, element #2=w198:dbl, element #3=w197:dbl, element #4=w196:dbl, element #5=w195:dbl, element #6=w194:dbl)  [unwired: 6 in]
              n91 = Format Into String(format string="%g_%g_%g_%g_%g_%g", w199, w198, w197, w196, w195, w194) -> (resulting string=w192:string)  [unwired: 2 in, 1 out]
              n92 = Concatenate Strings("abs:" ("string"), w192, ":wait" ("string")) -> (w187:string)
            }
            frame "mirror" {
              n93 = call-poly <vilib>:"Vector Norm.vi"("Input Vector"="scan_mirr_deltas 2") -> ("norm"=w208:dbl)  [unwired: 9 in, 1 out]
              n94 = Divide(x="scan_mirr_deltas 2", y=w208) -> (x/y=w209:dbl[])
              n95 = Multiply(x=w209, y=w203) -> (x*y=w216:dbl[])
              n96 = Add(x="scan_mirr_start 2", y=w216) -> (x+y=w217:dbl[])
              n97 = Index Array(array=w217) -> (element #1=w213:dbl, element #2=w212:dbl)  [unwired: 2 in]
              n98 = Format Into String(format string="%g_%g", w213, w212) -> (resulting string=w210:string)  [unwired: 2 in, 1 out]
              n99 = Concatenate Strings("abs:" ("string"), w210, ":wait" ("string")) -> (w205:string)
            }
            frame "temperature" {
              n100 = Number To Fractional String(number=w221) -> (F-format string=w223:string)  [unwired: 3 in]
              n101 = Concatenate Strings("ramp:" ("string"), w223) -> (w224:string)
              n102 = case shown="True" "Wait for T 2" {
                tunnel: w224 -> [w226 w229]
                tunnel: ":wait" ("string") -> [_ w228]
                tunnel: [w226 w227] -> w219
                frame False {
                }
                frame True {
                  n103 = Concatenate Strings(w229, w228) -> (w227:string)
                }
              }
            }
            frame "voltage" {
              n104 = Number To Fractional String(number=w232) -> (F-format string=w236:string)  [unwired: 3 in]
              n105 = Concatenate Strings("setsgl:" ("string"), "scan_volt_parameter 2", ":" ("string"), w236) -> (w231:string)
            }
          }
        }
        n106 = Array Size(array=w125) -> (size(s)=w122:i32)
        n107 = Equal To 0?(x=w122) -> (x = 0?=w124:bool)
        n108 = Select(t=1, s=w124, f=w122) -> (s? t:f=w121:i32)
        n109 = Get Date/Time In Seconds() -> (seconds since 1Jan1904=w137:timestamp)
        n110 = for {
          N: w121 -> [w242]
          tunnel: w142 -> [w279]
          tunnel: dbl[][][] [] -> [w278]
          tunnel: [w277] -> w140
          tunnel: w139 -> [w274]
          tunnel: w137 -> [w276]
          tunnel: [w275] -> w136
          tunnel: w135 -> [w266]
          tunnel: w125 -> [w239]
          tunnel: w129 -> [w247]
          i -> [w237]
          # "i"
          # "n"
          n111 = local read "RunNumber"() -> (w259:u16)
          n112 = Index Array(array=w239, index=w237) -> (element=w238:string)
          n113 = Increment(x=w237) -> (x+1=w243:i32)
          "current scan 2" <- w243
          n114 = Not Equal?(x="", y=w238) -> (x != y?=w272:bool)
          n115 = local read "BasePath"() -> (w258:path)
          n116 = Divide(x=w242, y=w243) -> (x/y=→"scan 1":dbl)
          n117 = case shown="True" w272 {
            tunnel: w247 -> [_ w450]
            tunnel: w238 -> [_ w449]
            tunnel: w274 -> [_ w448]
            tunnel: [errorcluster {"status"=FALSE, "code"=0, "source"=""} ("error out") w445] -> w246
            frame False {
            }
            frame True {
              n118 = Cancel Notification(0:w448) -> (11:w447:errorcluster)  [unwired: 1 in, 2 out]
              n119 = Enqueue Element(queue=w450, element=w449, error in (no error)=w447) -> (error out=w446:errorcluster)  [unwired: 1 in, 2 out]
              n120 = Wait on Notification(notifier=w448, error in (no error)=w446) -> (error out=w445:errorcluster)  [unwired: 2 in, 3 out]
            }
          }
          n121 = Current VI's Path() -> (path=w260:path)
          n122 = Increment(x=w259) -> (x+1=w257:u16)
          n123 = call "create scan vectr.vi"("Table Control"="waypointsD1") -> ("Array"=w248:dbl[])
          n124 = flat-sequence {
            tunnel: w262 -> [w294]
            tunnel: w249 -> [w286]
            tunnel: w246 -> [w280]
            tunnel: [w280] -> w245
            frame #0 {
              n125 = local read "waveplate position"() -> (w283:dbl)
              n126 = local read "stage2 position"() -> (w282:dbl)
              n127 = local read "ESP_pos"() -> (w284:dbl)
              n128 = local read "TA"() -> (w285:dbl)
              n129 = local read "TB"() -> (w281:dbl)
              n130 = local read "ROI Bottom"() -> (w298:i32)
              n131 = property on="ana_mode" class="Enum (strict)"() -> ("RingText.Text"=w290:string)  [unwired: 2 in, 2 out]
              n132 = property on="ana_voltrange" class="Enum (strict)"() -> ("RingText.Text"=w291:string)  [unwired: 2 in, 2 out]
              n133 = local read "cam_dark?"() -> (w293:bool)
              n134 = local read "cam_avgs"() -> (w288:i32)
              n135 = local read "meas_iter"() -> (w289:i32)
              n136 = local read "ROI Right"() -> (w300:i32)
              n137 = local read "phoib_I_1"() -> (w303:dbl)
              n138 = local read "phoib_I_2"() -> (w304:dbl)
              n139 = local read "phoib_I_3"() -> (w305:dbl)
              n140 = local read "phoib_I_4"() -> (w306:dbl)
              n141 = local read "phoib_I_5"() -> (w307:dbl)
              n142 = local read "phoib_I_6"() -> (w308:dbl)
              n143 = local read "phoib_I_7"() -> (w309:dbl)
              n144 = local read "phoib_I_8"() -> (w310:dbl)
              n145 = local read "phoib_I_9"() -> (w311:dbl)
              n146 = local read "cam_exp"() -> (w295:u32)
              n147 = local read "ROI Top"() -> (w299:i32)
              n148 = local read "ROI Left"() -> (w301:i32)
              n149 = local read "binning"() -> (w297:u16)
              n150 = local read "ESP_t0"() -> (w312:dbl)
              n151 = local read "gain"() -> (w292:bool)
              n152 = Boolean To (0,1)(Boolean=w292) -> (0, 1=w296:i16)
              n153 = Boolean To (0,1)(Boolean=w293) -> (0, 1=w302:i16)
              n154 = Format Into String(format string="ScanType:%s\\nAverages:%u\\nRepetitions:%u\\nLensMode:%s\\nVoltageRange:%s\\nExposure:%u\\nGain:%u\\nBinning:%u\\nROIbottom:%u\\nROItop:%u\\nROIright:%u\\nROIleft:%u\\nDarkImg:%u\\nKineticEnergy:%f\\nPassEnergy:%f\\nCoilCurrent:%f\\nWorkFunction:%f\\nDetectorVoltage:%f\\nScreenVoltage:%f\\nConversionVoltage:%f\\nFocusDisplacement1:%f\\nFocusDisplacement2:%f\\nTimeZero:%f\\nDelayStage:%f\\nWaveplate:%f\\n2ndStage:%f\\nTempA:%f\\nTempB:%f\\n", initial string=w286, w294, w288, w289, w290, w291, w295, w296, w297, w298, w299, w300, w301, w302, w303, w304, w305, w306, w307, w308, w309, w310, w311, w312, w284, w283, w282, w285, w281) -> ()  [unwired: 1 in, 2 out]
            }
          }
          n155 = call "create_opti_path.vi"("RunNumber"=w257, "base path"=w258) -> ("Path"=w250:path)  [unwired: 2 in]
          n156 = call "saverunnumber.vi"("RunNumber"=w257, "VI path"=w260) -> ()  [unwired: 10 in]
          n157 = local write "RunNumber"(w257) -> ()
          n158 = Unbundle(w266) -> ("queue out"=w265:refnum<queue>, "queue out"=w267:refnum<queue>, "queue out"=w268:refnum<queue>, "queue out"=w269:refnum<queue>, "queue out"=w270:refnum<queue>, "queue out"=w271:refnum<queue>)
          n159 = Build Path(base path=w250, name or relative path="scanvector.txt") -> (appended path=w252:path)
          n160 = for {
            tunnel: [w331] -> w264 mode=indexing
            tunnel: [w330] -> w263
            tunnel: w267 -> [w329]
            tunnel: w268 -> [w328]
            tunnel: w269 -> [w327]
            tunnel: w270 -> [w326]
            tunnel: w252 -> [w325]
            tunnel: w271 -> [w324]
            tunnel: w248 -> [w323] mode=indexing
            tunnel: "scan_selector" -> [w321]
            i -> [w320]
            stop <- w322 stop-if-true
            n161 = case shown="\"voltage\"" w321 {
              tunnel: w323 -> [w340 _ w354 w365 w396 w408 w425 w434]
              tunnel: [w338 w348 w351 w366 w384 w405 w423 w438] -> w330
              tunnel: [w343 "" w355 w367 w385 w406 w418 w439] -> w331
              tunnel: w329 -> [w338 w348 w351 w366 _ _ _ _]
              tunnel: w328 -> [_ _ _ _ w384 _ _ _]
              tunnel: w327 -> [_ _ _ _ _ _ _ w438]
              tunnel: w326 -> [_ _ _ _ _ w405 _ _]
              tunnel: w325 -> [w333 _ w353 w364 w380 w402 w426 w435]
              tunnel: w324 -> [_ _ _ _ _ _ w423 _]
              tunnel: [_ TRUE _ _ _ _ _ _] -> w322
              tunnel: w320 -> [_ _ _ _ _ _ _ _]
              frame "delay" {
                w345 = ":" ("string")
                n162 = local read "ESP_t0"() -> (w339:dbl)
                n163 = call "time2mm.vi"("fs[1]/ps[0]"=TRUE, "Offset (mm)"=w339, "time"=w340) -> ("position (mm)"=w335:dbl)
                n164 = Build Array(w335) -> (w334:dbl[])
                n165 = Number To Decimal String(number=0) -> (decimal integer string=w342:string)  [unwired: 1 in]
                n166 = Number To Fractional String(number=w335) -> (F-format string=w347:string)  [unwired: 3 in]
                n167 = call-poly <vilib>:"Write Delimited Spreadsheet.vi"("file path (dialog if empty)"=w333, "format (%.3f)"="%.6f", "1D data"=w334, "append to file? (F)"=TRUE) -> ()  [unwired: 10 in, 2 out]
                n168 = Concatenate Strings("abs:" ("string"), w342, w345, w347, w345, "wait" ("string")) -> (w343:string)
              }
              frame "none", Default {
              }
              frame "waveplate" {
                w352 = ":" ("string")
                n169 = Number To Fractional String(number=w354) -> (F-format string=w363:string)  [unwired: 3 in]
                n170 = Build Array(w354) -> (w357:dbl[])
                n171 = Number To Decimal String(number=1) -> (decimal integer string=w360:string)  [unwired: 1 in]
                n172 = call-poly <vilib>:"Write Delimited Spreadsheet.vi"("file path (dialog if empty)"=w353, "format (%.3f)"="%.6f", "1D data"=w357, "append to file? (F)"=TRUE) -> ()  [unwired: 10 in, 2 out]
                n173 = Concatenate Strings("abs:" ("string"), w360, w352, w363, w352, "wait" ("string")) -> (w355:string)
              }
              frame "stage2" {
                w369 = ":" ("string")
                n174 = Build Array(w365) -> (w374:dbl[])
                n175 = Number To Decimal String(number=2) -> (decimal integer string=w375:string)  [unwired: 1 in]
                n176 = Number To Fractional String(number=w365) -> (F-format string=w376:string)  [unwired: 3 in]
                n177 = call-poly <vilib>:"Write Delimited Spreadsheet.vi"("file path (dialog if empty)"=w364, "format (%.3f)"="%.6f", "1D data"=w374, "append to file? (F)"=TRUE) -> ()  [unwired: 10 in, 2 out]
                n178 = Concatenate Strings("abs:" ("string"), w375, w369, w376, w369, "wait" ("string")) -> (w367:string)
              }
              frame "manipulator" {
                n179 = call-poly <vilib>:"Vector Norm.vi"("Input Vector"="scan_manip_deltas") -> ("norm"=w398:dbl)  [unwired: 9 in, 1 out]
                n180 = Divide(x="scan_manip_deltas", y=w398) -> (x/y=w397:dbl[])
                n181 = Multiply(x=w397, y=w396) -> (x*y=w383:dbl[])
                n182 = Add(x="scan_manip_start", y=w383) -> (x+y=w379:dbl[])
                n183 = call-poly <vilib>:"Write Delimited Spreadsheet.vi"("file path (dialog if empty)"=w380, "format (%.3f)"="%.6f", "1D data"=w379, "append to file? (F)"=TRUE) -> ()  [unwired: 10 in, 2 out]
                n184 = Index Array(array=w379) -> (element #1=w387:dbl, element #2=w388:dbl, element #3=w389:dbl, element #4=w390:dbl, element #5=w391:dbl, element #6=w392:dbl)  [unwired: 6 in]
                n185 = Format Into String(format string="%g_%g_%g_%g_%g_%g", w387, w388, w389, w390, w391, w392) -> (resulting string=w394:string)  [unwired: 2 in, 1 out]
                n186 = Concatenate Strings("abs:" ("string"), w394, ":wait" ("string")) -> (w385:string)
              }
              frame "mirror" {
                n187 = call-poly <vilib>:"Vector Norm.vi"("Input Vector"="scan_mirr_deltas") -> ("norm"=w416:dbl)  [unwired: 9 in, 1 out]
                n188 = Divide(x="scan_mirr_deltas", y=w416) -> (x/y=w415:dbl[])
                n189 = Multiply(x=w415, y=w408) -> (x*y=w404:dbl[])
                n190 = Add(x="scan_mirr_start", y=w404) -> (x+y=w401:dbl[])
                n191 = call-poly <vilib>:"Write Delimited Spreadsheet.vi"("file path (dialog if empty)"=w402, "format (%.3f)"="%.6f", "1D data"=w401, "append to file? (F)"=TRUE) -> ()  [unwired: 10 in, 2 out]
                n192 = Index Array(array=w401) -> (element #1=w411:dbl, element #2=w412:dbl)  [unwired: 2 in]
                n193 = Format Into String(format string="%g_%g", w411, w412) -> (resulting string=w414:string)  [unwired: 2 in, 1 out]
                n194 = Concatenate Strings("abs:" ("string"), w414, ":wait" ("string")) -> (w406:string)
              }
              frame "temperature" {
                n195 = Build Array(w425) -> (w424:dbl[])
                n196 = Number To Fractional String(number=w425) -> (F-format string=w422:string)  [unwired: 3 in]
                n197 = Concatenate Strings("ramp:" ("string"), w422) -> (w420:string)
                n198 = case shown="True" "Wait for T" {
                  tunnel: w420 -> [w429 w432]
                  tunnel: ":wait" ("string") -> [_ w431]
                  tunnel: [w429 w430] -> w418
                  frame False {
                  }
                  frame True {
                    n199 = Concatenate Strings(w432, w431) -> (w430:string)
                  }
                }
                n200 = call-poly <vilib>:"Write Delimited Spreadsheet.vi"("file path (dialog if empty)"=w426, "format (%.3f)"="%.6f", "1D data"=w424, "append to file? (F)"=TRUE) -> ()  [unwired: 10 in, 2 out]
              }
              frame "voltage" {
                n201 = local read "scan_volt_parameter"() -> (w442:string)
                n202 = Build Array(w434) -> (w433:dbl[])
                n203 = Number To Fractional String(number=w434) -> (F-format string=w440:string)  [unwired: 3 in]
                n204 = Concatenate Strings("setsgl:" ("string"), w442, ":" ("string"), w440) -> (w439:string)
                n205 = call-poly <vilib>:"Write Delimited Spreadsheet.vi"("file path (dialog if empty)"=w435, "format (%.3f)"="%.6f", "1D data"=w433, "append to file? (F)"=TRUE) -> ()  [unwired: 10 in, 2 out]
              }
            }
          }
          n206 = Build Path(base path=w250, name or relative path="RAW\\LUT.txt") -> (appended path=w261:path)
          n207 = case shown="\"waveplate\"" "scan_selector" {
            tunnel: ["delay" ("input 1") "waveplate" ("input 1") "stage2" ("input 1") "manipulator" ("input 1") "temperature" "mirror" ("input 1") "voltage" ("input 1")] -> w262
            frame "delay", Default {
            }
            frame "waveplate" {
            }
            frame "stage2" {
            }
            frame "manipulator" {
            }
            frame "temperature" {
            }
            frame "mirror" {
            }
            frame "voltage" {
            }
          }
          n208 = Build Path(base path=w250, name or relative path="info.txt") -> (appended path=w249:path)
          n209 = call-poly <vilib>:"Write Delimited Spreadsheet.vi"("file path (dialog if empty)"=w261, "1D data"=string[] ["filename", "time", "delaystage", "X", "Y", "Z", "polar", "tilt", "azimuth", "mirrorX", "mirrorY", "KineticEnergy", "PassEnergy", "CoilCurrent", "WorkFunction", "DetectorVoltage", "ScreenVoltage", "ConversionVoltage", "FD1", "FD2"]) -> ("new file path (Not A Path if cancelled)"=w253:path)  [unwired: 12 in, 1 out]
          n210 = while {
            tunnel: w250 -> [w472]
            tunnel: w279 -> [w471]
            shift-right: [w470] -> w277
            shift-left: w278 -> [w469]
            tunnel: w274 -> [w468]
            tunnel: w276 -> [w467]
            tunnel: w263 -> [w466]
            tunnel: w264 -> [w465]
            tunnel: w265 -> [w464]
            shift-right: [w462] -> _
            shift-left: w253 -> [w463]
            shift-right: [w461] -> w275
            shift-left: w248 -> [w460]
            tunnel: w245 -> [w453]
            tunnel: w242 -> [w452]
            tunnel: w237 -> [w451]
            i -> [w459]
            stop <- w456 stop-if-true
            n211 = local read "meas_iter"() -> (w458:i32)
            n212 = for {
              N -> [w509]
              tunnel: w472 -> [w507]
              tunnel: w471 -> [w528]
              tunnel: w459 -> [w505]
              shift-right: [w519] -> w470
              shift-left: w469 -> [w524]
              tunnel: w468 -> [w521]
              tunnel: w467 -> [w508]
              tunnel: w466 -> [w501]
              tunnel: w465 -> [w481] mode=indexing
              tunnel: w464 -> [w500]
              shift-right: [w496] -> w462
              shift-left: w463 -> [w497]
              shift-right: [w492] -> w461
              shift-left: w460 -> [w492]
              tunnel: [w489] -> w455
              tunnel: w458 -> [w488]
              tunnel: w453 -> [w483]
              tunnel: w452 -> [w475]
              tunnel: w451 -> [w479]
              i -> [w506]
              stop <- "stop after step" stop-if-true
              n213 = Not Equal?(x="", y=w481) -> (x != y?=w480:bool)
              n214 = case shown="True" w480 {
                tunnel: [w533 w539] -> w523
                tunnel: w521 -> [_ w537]
                tunnel: w501 -> [_ w536]
                tunnel: w481 -> [_ w535]
                tunnel: w483 -> [w533 w534]
                frame False {
                }
                frame True {
                  n215 = Cancel Notification(0:w537, 3:w534) -> (11:w538:errorcluster)  [unwired: 2 out]
                  n216 = Enqueue Element(queue=w536, element=w535, error in (no error)=w538) -> (error out=w540:errorcluster)  [unwired: 1 in, 2 out]
                  n217 = Wait on Notification(notifier=w537, error in (no error)=w540) -> (error out=w539:errorcluster)  [unwired: 2 in, 3 out]
                }
              }
              n218 = Equal To 0?(x=w506) -> (x = 0?=w527:bool)
              n219 = Equal To 0?(x=w505) -> (x = 0?=w526:bool)
              n220 = Get Date/Time In Seconds() -> (seconds since 1Jan1904=w498:timestamp)
              n221 = And(x=w527, y=w526) -> (x .and. y?=w525:bool)
              n222 = Enqueue Element(queue=w500, element="snap", error in (no error)=w523) -> (error out=w522:errorcluster)  [unwired: 1 in, 2 out]
              n223 = call "createFileStruc.vi"("i_iter"=w505, "i_delay"=w506, "meas_path"=w507) -> ("AVG file"=w502:path, "RAW file"=w494:path)  [unwired: 7 in]
              n224 = Dequeue Element(queue=w528, error in (no error)=w522) -> (element=w504:dbl[][], error out=w495:errorcluster)  [unwired: 1 in, 2 out]
              n225 = Strip Path(path=w494) -> (name=w493:string)  [unwired: 1 out]
              n226 = Array Size(array=w504) -> (size(s)=w532:i32[])
              n227 = call-poly <vilib>:"Write Delimited Spreadsheet.vi"("file path (dialog if empty)"=w494, "2D data"=w504, "error in (no error)"=w495) -> ()  [unwired: 11 in, 2 out]
              n228 = Index Array(array=w532) -> (element #1=w530:i32, element #2=w529:i32)  [unwired: 2 in]
              n229 = Subtract(x=w498, y=w508) -> (x-y=w511:dbl)
              n230 = flat-sequence {
                tunnel: "%s\\t%<%Y.%m.%d %H:%M:%S>T\\t%f\\t%f\\t%f\\t%f\\t%f\\t%f\\t%f\\t%f\\t%f\\t%f\\t%f\\t%f\\t%f\\t%f\\t%f\\t%f\\t%f\\t%f\\t%f" -> [w570]
                tunnel: w498 -> [w569]
                tunnel: w497 -> [w546]
                tunnel: [w545] -> w496
                tunnel: w495 -> [w542]
                tunnel: w493 -> [w541]
                frame #0 {
                  n231 = local read "pos"() -> (w571:dbl[])
                  n232 = local read "mirr_posX"() -> (w558:i32)
                  n233 = local read "mirr_posY"() -> (w559:i32)
                  n234 = local read "ESP_delay"() -> (w551:dbl)
                  n235 = local read "phoib_I_1"() -> (w560:dbl)
                  n236 = local read "phoib_I_2"() -> (w561:dbl)
                  n237 = local read "phoib_I_3"() -> (w562:dbl)
                  n238 = local read "phoib_I_4"() -> (w563:dbl)
                  n239 = local read "phoib_I_5"() -> (w564:dbl)
                  n240 = local read "phoib_I_6"() -> (w565:dbl)
                  n241 = local read "phoib_I_7"() -> (w566:dbl)
                  n242 = local read "phoib_I_8"() -> (w567:dbl)
                  n243 = local read "phoib_I_9"() -> (w568:dbl)
                  n244 = local read "ESP_pos"() -> (w550:dbl)
                  n245 = Index Array(array=w571) -> (element #1=w552:dbl, element #2=w553:dbl, element #3=w554:dbl, element #4=w555:dbl, element #5=w556:dbl, element #6=w557:dbl)  [unwired: 6 in]
                  n246 = Format Into String(format string=w570, error in=w542, w541, w569, w550, w551, w552, w553, w554, w555, w556, w557, w558, w559, w560, w561, w562, w563, w564, w565, w566, w567, w568) -> (resulting string=w548:string)  [unwired: 1 in, 1 out]
                  n247 = Spreadsheet String To Array(format string="%s", spreadsheet string=w548, array type (2D Dbl)=string[] []) -> (array=w544:string[])  [unwired: 1 in]
                  n248 = call-poly <vilib>:"Write Delimited Spreadsheet.vi"("file path (dialog if empty)"=w546, "1D data"=w544, "append to file? (F)"=TRUE) -> ("new file path (Not A Path if cancelled)"=w545:path)  [unwired: 11 in, 1 out]
                }
              }
              n249 = case shown="True" w525 {
                tunnel: w509 -> [_ w577]
                tunnel: [w572 w575] -> w531
                tunnel: w524 -> [w572 _]
                tunnel: w530 -> [_ w574]
                tunnel: w529 -> [_ w573]
                frame False {
                }
                frame True {
                  n250 = Initialize Array(0.0 ("element"), w577, w574, w573) -> (w575:dbl[][][])
                }
              }
              n251 = Increment(x=w506) -> (x+1=w515:i32)
              "current scan" <- w515
              n252 = Increment(x=w505) -> (x+1=w514:i32)
              "current iteration" <- w514
              n253 = for {
                N: w530 -> [_]
                tunnel: w506 -> [w584]
                shift-right: [w582] -> w519
                shift-left: w531 -> [w585]
                tunnel: w505 -> [w580]
                shift-right: [w579] -> w503
                shift-left: w504 -> [w581]
                tunnel: w529 -> [w578]
                i -> [w583]
                n254 = for {
                  N: w578 -> [_]
                  tunnel: w584 -> [w592]
                  tunnel: w583 -> [w589]
                  shift-right: [w591] -> w582
                  shift-left: w585 -> [w593]
                  tunnel: w580 -> [w587]
                  shift-right: [w586] -> w579
                  shift-left: w581 -> [w590]
                  i -> [w588]
                  n255 = in-place {
                    in-place-border: w587 -> [w599]
                    n256 = in-place-array #1(w593, w592, w589, w588) -> (w600:dbl)
                    n257 = in-place-array #2(w590, w589, w588) -> (w597:dbl)
                    n258 = Multiply(x=w600, y=w599) -> (x*y=w598:dbl)
                    n259 = Increment(x=w599) -> (x+1=w595:i32)
                    n260 = Add(x=w598, y=w597) -> (x+y=w596:dbl)
                    n261 = Divide(x=w596, y=w595) -> (x/y=w594:dbl)
                    n262 = in-place-array #1(w594) -> (w591:dbl[][][])  [unwired: 3 out]
                    n263 = in-place-array #2(w594) -> (w586:dbl[][])  [unwired: 2 out]
                  }
                }
              }
              n264 = Multiply(x=w509, y=w505) -> (x*y=w510:i32)
              n265 = Multiply(x=w509, y=w488) -> (x*y=w474:i32)
              n266 = Divide(x=w515, y=w509) -> (x/y=→"scan 2":dbl)
              n267 = Divide(x=w514, y=w488) -> (x/y=→"iteration":dbl)
              n268 = Add(x=w506, y=w510) -> (x+y=w477:i32)
              n269 = Multiply(x=w479, y=w474) -> (x*y=w478:i32)
              n270 = Add(x=w477, y=w478) -> (x+y=w476:i32)
              n271 = Divide(x=w511, y=w476) -> (x/y=w484:dbl)
              n272 = Multiply(x=w475, y=w474) -> (x*y=w473:i32)
              n273 = Multiply(x=w484, y=w473) -> (x*y=w487:dbl)
              n274 = local write "duration [HH:MM:SS]"(w487) -> ()
              n275 = local write "time/step [s]"(w484) -> ()
              n276 = property on="mainimg" class="IntGraph (strict)"() -> ("CrsrLis"=w518:T5)  [unwired: 2 in, 2 out]
              n277 = call-poly <vilib>:"Write Delimited Spreadsheet.vi"("file path (dialog if empty)"=w502, "2D data"=w503) -> ()  [unwired: 12 in, 2 out]
              n278 = call "processData.vi"("Cursor List"=w518, "data in"=w519) -> ("Angle Chart"=→"anglegraph":dbl[][], "Energy Chart"=→"energygraph":dbl[][], "Intensity Chart"=w517:dbl[])  [unwired: 1 in]
              n279 = Bundle("Array"=w492, "Intensity Chart"=w517) -> (→"intensitygraph":cluster{"Array":dbl[], "Intensity Chart":dbl[]})  [unwired: 1 in]
              n280 = Or(x="stop after iteration", y="stop after step") -> (x .or. y?=w489:bool)
            }
            n281 = Increment(x=w459) -> (x+1=w457:i32)
            n282 = Greater Or Equal?(x=w457, y=w458) -> (x >= y?=w454:bool)
            n283 = Or(x=w455, y=w454) -> (x .or. y?=w456:bool)
          }
        }
      }
      frame "refresh" {
        n284 = Dequeue Element(queue=w601) -> ()  [unwired: 2 in, 4 out]
        n285 = property on="mainimg" class="IntGraph (strict)"() -> ("CrsrLis"=w608:T5)  [unwired: 2 in, 2 out]
        n286 = call "processData.vi"("Cursor List"=w608, "data in"=w607) -> ("Angle Chart"=w605:dbl[][], "Energy Chart"=w606:dbl[][], "Intensity Chart"=w602:dbl[])  [unwired: 1 in]
        n287 = Bundle("Array"=w603, "Intensity Chart"=w602) -> (w604:cluster{"Array":dbl[], "Intensity Chart":dbl[]})  [unwired: 1 in]
        n288 = local write "energygraph"(w606) -> ()
        n289 = local write "intensitygraph"(w604) -> ()
        n290 = local write "anglegraph"(w605) -> ()
      }
    }
  }
  n291 = while {
    tunnel: w20 -> [w617]
    tunnel: w19 -> [w616]
    tunnel: w18 -> [w615]
    tunnel: w17 -> [w614]
    tunnel: w22 -> [w612]
    tunnel: w29 -> [w613]
    tunnel: w5 -> [w611]
    tunnel: w10 -> [w610]
    tunnel: w1 -> [w609]
    stop <- w618 stop-if-true
    n292 = event shown="[12] \"scan_go\": Value Change" {
      selector: _ -> [_ _ _ _ _ _ _ _ _ _ _ _ _ _ _ _ _ _ _ _ _ _ _ _ _ _ _ _ _ _ _ _ _ _ _]
      dyn-events: _ -> [_ _ _ _ _ _ _ _ _ _ _ _ _ _ _ _ _ _ _ _ _ _ _ _ _ _ _ _ _ _ _ _ _ _ _]
      timeout: _ -> [_ _ _ _ _ _ _ _ _ _ _ _ _ _ _ _ _ _ _ _ _ _ _ _ _ _ _ _ _ _ _ _ _ _ _]
      tunnel: [_ TRUE _ _ _ _ _ _ _ _ _ _ _ _ _ _ _ _ _ _ _ _ _ _ _ _ _ _ _ _ _ _ _ _ _] -> w618
      tunnel: w617 -> [_ w633 w645 _ _ _ _ _ _ w673 w675 _ _ _ _ _ _ _ _ _ _ _ _ _ _ _ _ _ _ _ _ _ _ _ _]
      tunnel: w616 -> [_ w632 _ w649 _ _ _ _ _ _ _ _ _ _ _ _ _ _ _ _ _ _ w754 _ _ w776 _ _ _ _ _ _ _ _ _]
      tunnel: w615 -> [_ w631 _ _ w655 _ _ _ _ _ _ _ _ _ _ _ _ _ _ w728 w744 w746 _ _ _ _ _ _ _ _ _ _ _ _ _]
      tunnel: w614 -> [_ w630 _ _ _ _ w663 w669 w670 _ _ _ _ _ _ _ _ _ _ _ _ _ _ _ _ _ _ _ _ _ _ _ _ _ _]
      tunnel: w613 -> [_ w638 _ _ _ _ _ _ _ _ _ _ _ _ _ _ _ _ _ _ _ _ _ _ _ _ _ _ _ _ _ _ _ _ _]
      tunnel: w612 -> [_ w629 _ _ _ _ _ _ _ _ _ w677 w679 _ _ _ _ _ _ _ _ _ _ _ _ _ _ _ _ _ _ _ w800 _ _]
      tunnel: w611 -> [_ w637 _ _ _ _ _ _ _ _ _ _ _ _ _ _ _ _ _ _ _ _ _ _ _ _ _ _ _ _ _ _ _ _ _]
      tunnel: w610 -> [_ w628 _ _ _ _ _ _ _ _ _ _ _ _ w702 _ _ _ _ _ _ _ _ _ _ _ _ _ _ _ _ _ _ w802 w823]
      tunnel: w609 -> [_ w621 _ _ _ _ _ _ _ _ _ _ _ _ _ _ _ _ _ _ _ _ _ _ _ _ _ _ _ _ _ _ _ _ _]
      event Timeout {
        n293 = event-data() -> ()  [unwired: 1 in, 1 out]
      }
      event "main_close": Value Change {
        w619 = "close" ("element")
        w634 = "release" ("element")
        n294 = event-data() -> ()  [unwired: 1 in, 1 out]
        n295 = Flush Queue(queue=w633) -> (queue out=w627:refnum<queue>)  [unwired: 1 in, 2 out]
        n296 = Flush Queue(queue=w632) -> (queue out=w626:refnum<queue>)  [unwired: 1 in, 2 out]
        n297 = Flush Queue(queue=w631) -> (queue out=w625:refnum<queue>)  [unwired: 1 in, 2 out]
        n298 = Flush Queue(queue=w630) -> (queue out=w624:refnum<queue>)  [unwired: 1 in, 2 out]
        n299 = Flush Queue(queue=w629) -> (queue out=w623:refnum<queue>)  [unwired: 1 in, 2 out]
        n300 = Flush Queue(queue=w628) -> (queue out=w622:refnum<queue>)  [unwired: 1 in, 2 out]
        n301 = Flush Queue(queue=w621) -> (queue out=w620:refnum<queue>)  [unwired: 1 in, 2 out]
        n302 = Release Notifier(notifier=w637) -> ()  [unwired: 2 in, 3 out]
        n303 = Release Queue(queue=w638) -> ()  [unwired: 2 in, 3 out]
        n304 = Enqueue Element(queue=w627, element=w634) -> (queue out=w642:refnum<queue>)  [unwired: 2 in, 2 out]
        n305 = Enqueue Element(queue=w626, element=w634) -> (queue out=w641:refnum<queue>)  [unwired: 2 in, 2 out]
        n306 = Enqueue Element(queue=w625, element=w634) -> (queue out=w640:refnum<queue>)  [unwired: 2 in, 2 out]
        n307 = Enqueue Element(queue=w624, element=w634) -> (queue out=w639:refnum<queue>)  [unwired: 2 in, 2 out]
        n308 = Enqueue Element(queue=w622, element=w634) -> (queue out=w636:refnum<queue>, error out=w635:errorcluster)  [unwired: 2 in, 1 out]
        n309 = Enqueue Element(queue=w642, element=w619) -> ()  [unwired: 2 in, 3 out]
        n310 = Enqueue Element(queue=w641, element=w619) -> ()  [unwired: 2 in, 3 out]
        n311 = Enqueue Element(queue=w640, element=w619) -> ()  [unwired: 2 in, 3 out]
        n312 = Enqueue Element(queue=w639, element=w619) -> ()  [unwired: 2 in, 3 out]
        n313 = Enqueue Element(queue=w623, element=w619) -> ()  [unwired: 2 in, 3 out]
        n314 = Enqueue Element(queue=w636, element=w619, error in (no error)=w635) -> ()  [unwired: 1 in, 3 out]
        n315 = Enqueue Element(queue=w620, element=w619) -> ()  [unwired: 2 in, 3 out]
      }
      event "cam_release", "cam_init": Value Change {
        n316 = event-data() -> ()  [unwired: 1 in, 2 out]
        n317 = Select(t="init" ("name (unnamed)"), s="cam_init", f="release" ("name (unnamed)")) -> (s? t:f=w644:string)
        n318 = Enqueue Element(queue=w645, element=w644) -> ()  [unwired: 2 in, 3 out]
      }
      event "ESP_release", "ESP_init": Value Change {
        n319 = event-data() -> ()  [unwired: 1 in, 2 out]
        n320 = Select(t="init" ("name (unnamed)"), s="ESP_init", f="release" ("name (unnamed)")) -> (s? t:f=w653:string)
        n321 = Enqueue Element(queue=w649, element=w653) -> ()  [unwired: 2 in, 3 out]
      }
      event "manip_init", "manip_release": Value Change {
        n322 = event-data() -> ()  [unwired: 1 in, 2 out]
        n323 = Flush Queue(queue=w655) -> (queue out=w654:refnum<queue>)  [unwired: 1 in, 2 out]
        n324 = Select(t="init" ("name (unnamed)"), s="manip_init", f="release" ("name (unnamed)")) -> (s? t:f=w657:string)
        n325 = Enqueue Element(queue=w654, element=w657) -> ()  [unwired: 2 in, 3 out]
      }
      event "setpoint_set": Value Change {
        n326 = event-data() -> ()  [unwired: 1 in, 2 out]
        n327 = local read "Setpoint"() -> (w661:dbl)
        n328 = local read "LS310  EPICS SP"() -> (w660:string)
        n329 = call-poly <userlib>:"CaLabPut.vi"("Value"=w661, "PV Name"=w660) -> ()  [unwired: 6 in, 4 out]
      }
      event "phoib_release", "phoib_init": Value Change {
        n330 = event-data() -> ()  [unwired: 1 in, 2 out]
        n331 = Flush Queue(queue=w663) -> (queue out=w662:refnum<queue>)  [unwired: 1 in, 2 out]
        n332 = Select(t="init" ("name (unnamed)"), s="phoib_init", f="release" ("name (unnamed)")) -> (s? t:f=w665:string)
        n333 = Enqueue Element(queue=w662, element=w665) -> ()  [unwired: 2 in, 3 out]
      }
      event "phoib_standby": Value Change {
        n334 = event-data() -> ()  [unwired: 1 in, 2 out]
        n335 = Enqueue Element(queue=w669, element="standby") -> ()  [unwired: 2 in, 3 out]
      }
      event "phoib_set": Value Change {
        n336 = event-data() -> ()  [unwired: 1 in, 2 out]
        n337 = Enqueue Element(queue=w670, element="set") -> ()  [unwired: 2 in, 3 out]
      }
      event "cam_dark": Value Change {
        n338 = event-data() -> ()  [unwired: 1 in, 2 out]
        n339 = Enqueue Element(queue=w673, element="dark") -> ()  [unwired: 2 in, 3 out]
      }
      event "ROI Left", "ROI Right", "ROI Top", "ROI Bottom", "cam_exp", "binning", "gain": Value Change {
        n340 = event-data() -> ()  [unwired: 1 in, 1 out]
        n341 = Enqueue Element(queue=w675, element="set") -> ()  [unwired: 2 in, 3 out]
      }
      event "cam_saveimg": Value Change {
        n342 = event-data() -> ()  [unwired: 1 in, 1 out]
        n343 = Enqueue Element(queue=w677, element="single") -> ()  [unwired: 2 in, 3 out]
      }
      event "scan_go": Value Change {
        n344 = event-data() -> ()  [unwired: 1 in, 1 out]
        n345 = Enqueue Element(queue=w679, element="scan") -> ()  [unwired: 2 in, 3 out]
      }
      event "meas_iter", "waypointsD1", "waypointsD2": Value Change {
        n346 = event-data() -> ()  [unwired: 1 in, 6 out]
        n347 = local read "waypointsD2"() -> (w690:string[][])
        n348 = local read "waypointsD1"() -> (w700:string[][])
        n349 = call "create scan vectr.vi"("Table Control"=w690) -> ("Array"=w689:dbl[])
        n350 = call "create scan vectr.vi"("Table Control"=w700) -> ("Array"=w699:dbl[])
        n351 = Array Size(array=w689) -> (size(s)=w687:i32)
        n352 = Array Size(array=w699) -> (size(s)=w683:i32)
        n353 = local read "meas_iter"() -> (w695:i32)
        n354 = local read "binning"() -> (w697:u16)
        n355 = Equal To 0?(x=w687) -> (x = 0?=w688:bool)
        n356 = Select(t=1, s=w688, f=w687) -> (s? t:f=w685:i32)
        n357 = Index Array(array=dbl[] [8.79, 2.2, 0.553, 0.138], index=w697) -> (element=w694:dbl)
        n358 = Multiply(x=w685, y=w683) -> (x*y=w684:i32)
        "measpoints" <- w684
        n359 = Multiply(x=w684, y=w695) -> (x*y=w692:i32)
        "total steps" <- w692
        n360 = Get Date/Time In Seconds() -> (seconds since 1Jan1904=w682:timestamp)
        n361 = Multiply(x=w692, y=w694) -> (x*y=→"disk [MB]":dbl)
        n362 = Multiply(x=w692, y="time/step [s]") -> (x*y=w681:dbl)
        "duration [HH:MM:SS]" <- w681
        n363 = Multiply(x=w683, y=w694) -> (x*y=→"RAM [MB]":dbl)
        n364 = Add(x=w682, y=w681) -> (x+y=→"ETA 2":timestamp)
      }
      event "mirr_go": Value Change {
        n365 = event-data() -> ()  [unwired: 1 in, 1 out]
        n366 = Index Array(array="mirr_dest") -> (element #1=w707:i32, element #2=w706:i32)  [unwired: 2 in]
        n367 = Format Into String(format string="%g_%g", w707, w706) -> (resulting string=w704:string)  [unwired: 2 in, 1 out]
        n368 = Concatenate Strings("abs:" ("string"), w704) -> (w701:string)
        n369 = Enqueue Element(queue=w702, element=w701) -> ()  [unwired: 2 in, 3 out]
      }
      event "scan_manip_setstart": Value Change {
        n370 = event-data() -> ()  [unwired: 1 in, 1 out]
        n371 = local read "pos"() -> (w709:dbl[])
        n372 = local write "scan_manip_start"(w709) -> ()
      }
      event "scan_manip_setstart 2": Value Change {
        n373 = event-data() -> ()  [unwired: 1 in, 1 out]
        n374 = local read "pos"() -> (w710:dbl[])
        n375 = local write "scan_manip_start 2"(w710) -> ()
      }
      event "scan_mirr_setstart": Value Change {
        n376 = event-data() -> ()  [unwired: 1 in, 1 out]
        n377 = local read "mirr_posX"() -> (w713:i32)
        n378 = local read "mirr_posY"() -> (w712:i32)
        n379 = Build Array(w713, w712) -> (w711:i32[])
        n380 = local write "scan_mirr_start"(w711) -> ()
      }
      event "scan_mirr_setstart 2": Value Change {
        n381 = event-data() -> ()  [unwired: 1 in, 1 out]
        n382 = local read "mirr_posX"() -> (w716:i32)
        n383 = local read "mirr_posY"() -> (w715:i32)
        n384 = Build Array(w716, w715) -> (w714:i32[])
        n385 = local write "scan_mirr_start 2"(w714) -> ()
      }
      event "Move Abs": Value Change {
        n386 = event-data() -> ()  [unwired: 1 in, 1 out]
        n387 = Index Array(array="dest") -> (element #1=w726:dbl, element #2=w725:dbl, element #3=w724:dbl, element #4=w723:dbl, element #5=w722:dbl, element #6=w721:dbl)  [unwired: 6 in]
        n388 = Format Into String(format string="%g_%g_%g_%g_%g_%g", w726, w725, w724, w723, w722, w721) -> (resulting string=w719:string)  [unwired: 2 in, 1 out]
        n389 = Concatenate Strings("abs:" ("string"), w719) -> (w718:string)
        n390 = Enqueue Element(queue=w728, element=w718) -> ()  [unwired: 2 in, 3 out]
      }
      event "ManipRel +", "ManipRel -": Value Change {
        n391 = event-data() -> ()  [unwired: 1 in, 2 out]
        n392 = Negate(x="manip_deltas") -> (-x=w732:dbl[])
        n393 = Select(t="manip_deltas", s="ManipRel +", f=w732) -> (s? t:f=w730:dbl[])
        n394 = Index Array(array=w730) -> (element #1=w736:dbl, element #2=w737:dbl, element #3=w738:dbl, element #4=w739:dbl, element #5=w740:dbl, element #6=w741:dbl)  [unwired: 6 in]
        n395 = Format Into String(format string="%g_%g_%g_%g_%g_%g", w736, w737, w738, w739, w740, w741) -> (resulting string=w743:string)  [unwired: 2 in, 1 out]
        n396 = Concatenate Strings("rel:" ("string"), w743, ":wait" ("string")) -> (w734:string)
        n397 = Enqueue Element(queue=w744, element=w734) -> ()  [unwired: 2 in, 3 out]
      }
      event "stop manip": Value Change {
        n398 = event-data() -> ()  [unwired: 1 in, 1 out]
        n399 = Enqueue Element(queue=w746, element="stop") -> ()  [unwired: 2 in, 3 out]
      }
      event "ESP_go": Value Change {
        w748 = ":" ("string")
        n400 = event-data() -> ()  [unwired: 1 in, 1 out]
        n401 = Number To Decimal String(number=0) -> (decimal integer string=w750:string)  [unwired: 1 in]
        n402 = Number To Fractional String(number="ESP_dest") -> (F-format string=w749:string)  [unwired: 3 in]
        n403 = Concatenate Strings("abs:" ("string"), w750, w748, w749, w748) -> (w753:string)
        n404 = Enqueue Element(queue=w754, element=w753) -> ()  [unwired: 2 in, 3 out]
      }
      event "ESP_set_t0": Value Change {
        n405 = event-data() -> ()  [unwired: 1 in, 1 out]
        n406 = Current VI's Path() -> (path=w765:path)
        n407 = Strip Path(path=w765) -> (stripped path=w763:path)  [unwired: 1 out]
        n408 = Strip Path(path=w763) -> (stripped path=w762:path)  [unwired: 1 out]
        n409 = local read "ESP_pos"() -> (w764:dbl)
        "ESP_t0" <- w764
        n410 = Number To Fractional String(number=w764) -> (F-format string=w757:string)  [unwired: 3 in]
        n411 = Build Path(base path=w762, name or relative path="t0.txt") -> (appended path=w759:path)
        n412 = Get Date/Time In Seconds() -> (seconds since 1Jan1904=w761:timestamp)
        n413 = Format Date/Time String(time format string (%c)="%Y.%m.%d %H:%M", seconds (now)=w761) -> (date/time string=w758:string)  [unwired: 1 in]
        n414 = Build Array(w758, w757) -> (w756:string[])
        n415 = call-poly <vilib>:"Write Delimited Spreadsheet.vi"("file path (dialog if empty)"=w759, "1D data"=w756, "append to file? (F)"=TRUE) -> ()  [unwired: 11 in, 2 out]
      }
      event "ESP_opent0file": Value Change {
        n416 = event-data() -> ()  [unwired: 1 in, 6 out]
        n417 = Current VI's Path() -> (path=w769:path)
        n418 = Strip Path(path=w769) -> (stripped path=w768:path)  [unwired: 1 out]
        n419 = Strip Path(path=w768) -> (stripped path=w770:path)  [unwired: 1 out]
        n420 = call <vilib>:"System Exec.vi"("wait until completion? (T)"=FALSE, "working directory"=w770, "command line"="notepad t0.txt") -> ()  [unwired: 5 in, 4 out]
      }
      event "ESP_+", "ESP_-": Value Change {
        n421 = event-data() -> ()  [unwired: 1 in, 6 out]
        n422 = Negate(x="ESP_delta") -> (-x=w779:dbl)
        n423 = Select(t="ESP_delta", s="ESP_+", f=w779) -> (s? t:f=w777:dbl)
        n424 = Number To Decimal String(number=0) -> (decimal integer string=w775:string)  [unwired: 1 in]
        n425 = Number To Fractional String(number=w777) -> (F-format string=w773:string)  [unwired: 3 in]
        n426 = Concatenate Strings("rel:" ("string"), w775, ":" ("string"), w773) -> (w782:string)
        n427 = Enqueue Element(queue=w776, element=w782) -> ()  [unwired: 2 in, 3 out]
      }
      event "ESP_dest": Value Change {
        n428 = event-data() -> ()  [unwired: 1 in, 6 out]
        n429 = local read "ESP_dest"() -> (w786:dbl)
        n430 = local read "ESP_t0"() -> (w785:dbl)
        n431 = call "mm2time.vi"("fs?"=TRUE ("fs[1]/ps[0]"), "Offset (mm)"=w785, "distance (mm)"=w786) -> ("time in fs/ps seconds"=w783:dbl)
        n432 = local write "ESP_dest_t"(w783) -> ()
      }
      event "ESP_dest_t": Value Change {
        n433 = event-data() -> ()  [unwired: 1 in, 1 out]
        n434 = local read "ESP_t0"() -> (w789:dbl)
        n435 = call "time2mm.vi"("fs[1]/ps[0]"=TRUE, "Offset (mm)"=w789, "time"="ESP_dest_t") -> ("position (mm)"=w787:dbl)
        n436 = local write "ESP_dest"(w787) -> ()
      }
      event "load waypoints 1": Value Change {
        n437 = event-data() -> ()  [unwired: 1 in, 6 out]
        n438 = call-poly <vilib>:"Read Delimited Spreadsheet.vi"() -> ("all rows"=w792:string[][], "error out"=w791:errorcluster)  [unwired: 10 in, 4 out]
        n439 = case shown="No Error" w791 {
          tunnel: w792 -> [w793 _]
          frame No Error {
            n440 = local write "waypointsD1"(w793) -> ()
          }
          frame Error {
          }
        }
      }
      event "load waypoints 2": Value Change {
        n441 = event-data() -> ()  [unwired: 1 in, 6 out]
        n442 = call-poly <vilib>:"Read Delimited Spreadsheet.vi"() -> ("all rows"=w795:string[][], "error out"=w794:errorcluster)  [unwired: 10 in, 4 out]
        n443 = case shown="No Error" w794 {
          tunnel: w795 -> [w796 _]
          frame No Error {
            n444 = local write "waypointsD2"(w796) -> ()
          }
          frame Error {
          }
        }
      }
      event "clear waypoints 1": Value Change {
        n445 = event-data() -> ()  [unwired: 1 in, 6 out]
        n446 = local write "waypointsD1"(string[][] []) -> ()
      }
      event "clear waypoints 2": Value Change {
        n447 = event-data() -> ()  [unwired: 1 in, 6 out]
        n448 = local write "waypointsD2"(string[][] []) -> ()
      }
      event "mainimg": Cursor Release {
        n449 = event-data() -> ()  [unwired: 1 in, 1 out]
        n450 = Enqueue Element(queue=w800, element="refresh") -> ()  [unwired: 2 in, 3 out]
      }
      event "mirr_init", "mirr_release": Value Change {
        n451 = event-data() -> ()  [unwired: 1 in, 6 out]
        n452 = Flush Queue(queue=w802) -> (queue out=w803:refnum<queue>)  [unwired: 1 in, 2 out]
        n453 = Select(t="init" ("name (unnamed)"), s="mirr_init", f="release" ("name (unnamed)")) -> (s? t:f=w804:string)
        n454 = Enqueue Element(queue=w803, element=w804) -> ()  [unwired: 2 in, 3 out]
      }
      event "mirr_X-", "mirr_X+", "mirr_Y+", "mirr_Y-": Value Change {
        n455 = event-data() -> ()  [unwired: 1 in, 1 out]
        n456 = local read "mirr_X#"() -> (w814:u8)
        n457 = local read "mirr_Y#"() -> (w813:u8)
        n458 = Or(x="mirr_X+", y="mirr_X-") -> (x .or. y?=w815:bool)
        n459 = Or(x="mirr_X-", y="mirr_Y-") -> (x .or. y?=w821:bool)
        n460 = Negate(x="mirr_rel") -> (-x=w820:i32)
        n461 = Select(t=w814, s=w815, f=w813) -> (s? t:f=w812:u8)
        n462 = Select(t=w820, s=w821, f="mirr_rel") -> (s? t:f=w809:i32)
        n463 = Number To Decimal String(number=w812) -> (decimal integer string=w811:string)  [unwired: 1 in]
        n464 = Number To Decimal String(number=w809) -> (decimal integer string=w808:string)  [unwired: 1 in]
        n465 = Concatenate Strings("rel:" ("string"), w811, ":" ("string"), w808) -> (w807:string)
        n466 = Enqueue Element(queue=w823, element=w807) -> ()  [unwired: 2 in, 3 out]
      }
    }
  }
  n467 = while {
    tunnel: w10 -> [w832]
    shift-right: [w829] -> _
    shift-left: _ -> [w830]
    tunnel: w5 -> [w828]
    shift-right: [w827] -> _
    shift-left: _ -> [w826]
    shift-right: [w824] -> _
    shift-left: _ -> [w825]
    stop <- w831 stop-if-true
    # "mirr"
    n468 = Preview Queue Element(queue=w832, timeout in ms (-1)=w830) -> (queue out=w835:refnum<queue>, element=w836:string)  [unwired: 1 in, 2 out]
    n469 = Match Pattern(string=w836, regular expression=":") -> (before substring=w834:string, after substring=w833:string)  [unwired: 1 in, 2 out]
    n470 = case shown="\"idle\", Default" w834 {
      tunnel: w835 -> [w871 w881 w896 w900 w903 w908 _]
      tunnel: w833 -> [w865 w882 _ _ _ _ _]
      tunnel: [_ _ _ TRUE _ _ _] -> w831
      tunnel: [_ _ _ _ -1 _ _] -> w829
      tunnel: w828 -> [w838 _ _ _ _ _ _]
      tunnel: [w857 w878 refnum<visa-resource-name> refnum ("VISA resource name out") w898 w902 w907 w913] -> w827
      tunnel: w826 -> [w870 w880 w895 w898 w902 _ w917]
      tunnel: [w842 w877 w894 w897 w901 w906 w912] -> w824
      tunnel: w825 -> [w869 w879 _ w897 w901 _ w916]
      frame "abs" {
        w853 = u8 20 items=["Echo"=55, "Home"=1, "Move Absolute"=20, "Move Relative"=21, "Move at Constant Speed"=22, "Renumber"=2, "Restore Settings"=36, "Stop"=23] ("Command")
        w868 = u8 20 items=["Echo"=55, "Home"=1, "Move Absolute"=20, "Move Relative"=21, "Move at Constant Speed"=22, "Renumber"=2, "Restore Settings"=36, "Stop"=23] ("Command")
        n471 = Dequeue Element(queue=w871) -> ()  [unwired: 2 in, 4 out]
        n472 = Match Pattern(string=w865, regular expression=":") -> (before substring=w855:string, after substring=w841:string)  [unwired: 1 in, 2 out]
        n473 = Equal?(x=w841, y="wait") -> (x = y?=w839:bool)
        n474 = Scan From String(format string="%g_%g", input string=w855) -> (output 1=w850:dbl, output 2=w849:dbl)  [unwired: 4 in, 3 out]
        n475 = local read "mirr_X#"() -> (w852:u8)
        n476 = Bundle("mirr_X#"=w852, "Command"=w868, w850, "Response Count"=1) -> (w864:T6)  [unwired: 1 in]
        n477 = local read "mirr_Y#"() -> (w851:u8)
        n478 = call "Request Command.vi"("error in (no error)"=w869, "Request"=w864, "VISA resource name"=w870) -> ("error out"=w846:errorcluster, "VISA resource name out"=w847:refnum<visa-resource-name>)  [unwired: 5 in, 2 out]
        n479 = Bundle("mirr_Y#"=w851, "Command"=w853, w849, "Response Count"=1) -> (w848:T7)  [unwired: 1 in]
        n480 = call "Request Command.vi"("error in (no error)"=w846, "Request"=w848, "VISA resource name"=w847) -> ("error out"=w844:errorcluster, "VISA resource name out"=w845:refnum<visa-resource-name>)  [unwired: 5 in, 2 out]
        n481 = local read "mirr_X#"() -> (w862:u8)
        n482 = call "zaber_readpos.vi"("error in (no error)"=w844, "axis"=w862, "VISA in"=w845) -> ("error out"=w858:errorcluster, "position"=w863:i32, "VISA out"=w859:refnum<visa-resource-name>)  [unwired: 6 in]
        n483 = local read "mirr_Y#"() -> (w860:u8)
        n484 = local write "mirr_posX"(w863) -> ()
        n485 = call "zaber_readpos.vi"("error in (no error)"=w858, "axis"=w860, "VISA in"=w859) -> ("error out"=w843:errorcluster, "position"=w861:i32, "VISA out"=w857:refnum<visa-resource-name>)  [unwired: 6 in]
        n486 = local write "mirr_posY"(w861) -> ()
        n487 = case shown="True" w839 {
          tunnel: w843 -> [w872 w876]
          tunnel: [w872 w875] -> w842
          tunnel: w838 -> [_ w874]
          frame False {
          }
          frame True {
            n488 = Send Notification(notification=TRUE, notifier=w874, error in (no error)=w876) -> (error out=w875:errorcluster)  [unwired: 1 out]
          }
        }
      }
      frame "rel" {
        w885 = u8 21 items=["Echo"=55, "Home"=1, "Move Absolute"=20, "Move Relative"=21, "Move at Constant Speed"=22, "Renumber"=2, "Restore Settings"=36, "Stop"=23] ("Command")
        n489 = Dequeue Element(queue=w881) -> ()  [unwired: 2 in, 4 out]
        n490 = Match Pattern(string=w882, regular expression=":") -> (before substring=w887:string, after substring=w886:string)  [unwired: 1 in, 2 out]
        n491 = Decimal String To Number(string=w887) -> (number=w889:i32)  [unwired: 2 in, 1 out]
        n492 = Decimal String To Number(string=w886) -> (number=w890:i32)  [unwired: 2 in, 1 out]
        n493 = Bundle(w889, "Command"=w885, w890, "Response Count"=1) -> (w883:T8)  [unwired: 1 in]
        n494 = call "Request Command.vi"("error in (no error)"=w879, "Request"=w883, "VISA resource name"=w880) -> ("error out"=w877:errorcluster, "VISA resource name out"=w878:refnum<visa-resource-name>)  [unwired: 5 in, 2 out]
      }
      frame "release" {
        n495 = Dequeue Element(queue=w896) -> (queue out=w892:refnum<queue>)  [unwired: 2 in, 3 out]
        n496 = Enqueue Element(queue=w892, element="suspend") -> ()  [unwired: 2 in, 3 out]
        n497 = call "Close.vi"("VISA resource name"=w895) -> ("error out"=w894:errorcluster)  [unwired: 9 in, 1 out]
      }
      frame "close" {
        n498 = Release Queue(queue=w900) -> ()  [unwired: 2 in, 3 out]
      }
      frame "suspend" {
        n499 = Dequeue Element(queue=w903) -> ()  [unwired: 2 in, 4 out]
      }
      frame "init" {
        n500 = Dequeue Element(queue=w908) -> ()  [unwired: 2 in, 4 out]
        n501 = call "Initialize.vi"("VISA resource name"="mirr_VISA") -> ("error out"=w906:errorcluster, "VISA resource name out"=w907:refnum<visa-resource-name>)  [unwired: 8 in, 1 out]
      }
      frame "idle", Default {
        n502 = local read "mirr_X#"() -> (w918:u8)
        n503 = call "zaber_readpos.vi"("error in (no error)"=w916, "axis"=w918, "VISA in"=w917) -> ("error out"=w914:errorcluster, "position"=→"mirr_posX":i32, "VISA out"=w915:refnum<visa-resource-name>)  [unwired: 6 in]
        n504 = local read "mirr_Y#"() -> (w911:u8)
        n505 = call "zaber_readpos.vi"("error in (no error)"=w914, "axis"=w911, "VISA in"=w915) -> ("error out"=w912:errorcluster, "position"=→"mirr_posY":i32, "VISA out"=w913:refnum<visa-resource-name>)  [unwired: 6 in]
      }
    }
    "mirr_Error" <- w824
  }
  n506 = while {
    tunnel: w19 -> [w928]
    shift-right: [w926] -> _
    shift-left: _ -> [w924]
    shift-right: [w925] -> _
    shift-left: _ -> [w923]
    shift-right: [w921] -> _
    shift-left: 0 -> [w922]
    tunnel: w5 -> [w920]
    stop <- w927 stop-if-true
    # "ESP"
    n507 = Preview Queue Element(queue=w928, timeout in ms (-1)=w922) -> (queue out=w931:refnum<queue>, element=w932:string)  [unwired: 1 in, 2 out]
    n508 = Match Pattern(string=w932, regular expression=":") -> (before substring=w930:string, after substring=w929:string)  [unwired: 1 in, 2 out]
    n509 = case shown="\"idle\", Default" w930 {
      tunnel: w931 -> [_ w954 w974 w1014 w1017 w1024 w1029]
      tunnel: w929 -> [_ w958 w980 _ _ _ _]
      tunnel: [_ _ _ _ _ TRUE _] -> w927
      tunnel: [w937 w960 w975 w1012 refnum<visa-resource-name> refnum ("VISA resource name out") w1021 w1028] -> w926
      tunnel: [w938 w961 w973 w1011 w1019 w1022 w1027] -> w925
      tunnel: w924 -> [w947 w963 w978 w1012 w1020 w1021 _]
      tunnel: w923 -> [w946 w962 w979 w1011 _ w1022 _]
      tunnel: [_ _ _ -1 _ _ _] -> w921
      tunnel: w920 -> [_ _ w967 _ _ _ _]
      tunnel: "ESP patch" -> [w944 w953 w966 _ _ _ _]
      frame "idle", Default {
        n510 = Index Array(array=w944) -> (element #1=w943:i32, element #2=w940:i32)  [unwired: 3 in, 1 out]
        n511 = local read "ESP_t0"() -> (w950:dbl)
        n512 = call "Read Actual Position.vi"("error in (no error)"=w946, "Axis (1)"=w943, "VISA resource name"=w947) -> ("error out"=w941:errorcluster, "Position (units)"=w945:dbl, "VISA resource name out"=w942:refnum<visa-resource-name>)  [unwired: 2 in]
        "ESP_pos" <- w945
        n513 = call "mm2time.vi"("fs?"=TRUE, "Offset (mm)"=w950, "distance (mm)"=w945) -> ("time in fs/ps seconds"=→"ESP_delay":dbl)
        n514 = call "Read Actual Position.vi"("error in (no error)"=w941, "Axis (1)"=w940, "VISA resource name"=w942) -> ("error out"=w939:errorcluster, "Position (units)"=→"waveplate position":dbl, "VISA resource name out"=w936:refnum<visa-resource-name>)  [unwired: 2 in]
        n515 = call "Read Actual Position.vi"("error in (no error)"=w939, "VISA resource name"=w936) -> ("error out"=w938:errorcluster, "Position (units)"=→"stage2 position":dbl, "VISA resource name out"=w937:refnum<visa-resource-name>)  [unwired: 3 in]
      }
      frame "rel" {
        n516 = Dequeue Element(queue=w954) -> ()  [unwired: 2 in, 4 out]
        n517 = Match Pattern(string=w958, regular expression=":") -> (before substring=w957:string, after substring=w956:string)  [unwired: 1 in, 2 out]
        n518 = Decimal String To Number(string=w957) -> (number=w952:i32)  [unwired: 2 in, 1 out]
        n519 = Fract/Exp String To Number(string=w956) -> (number=w955:dbl)  [unwired: 3 in, 1 out]
        n520 = Index Array(array=w953, index=w952) -> (element=w951:i32)
        n521 = call "Move Relative.vi"("error in (no error)"=w962, "Position (0 units)"=w955, "Axis (1)"=w951, "VISA resource name"=w963) -> ("error out"=w961:errorcluster, "VISA resource name out"=w960:refnum<visa-resource-name>)  [unwired: 2 in]
      }
      frame "abs" {
        n522 = Dequeue Element(queue=w974) -> ()  [unwired: 2 in, 4 out]
        n523 = Match Pattern(string=w980, regular expression=":") -> (before substring=w981:string, after substring=w971:string)  [unwired: 1 in, 2 out]
        n524 = Match Pattern(string=w971, regular expression=":") -> (before substring=w970:string, after substring=w969:string)  [unwired: 1 in, 2 out]
        n525 = Decimal String To Number(string=w981) -> (number=w965:i32)  [unwired: 2 in, 1 out]
        n526 = Fract/Exp String To Number(string=w970) -> (number=w968:dbl)  [unwired: 3 in, 1 out]
        n527 = Index Array(array=w966, index=w965) -> (element=w964:i32)
        n528 = call "Move Absolute.vi"("error in (no error)"=w979, "Position (0 units)"=w968, "Axis (1)"=w964, "VISA resource name"=w978) -> ("error out"=w976:errorcluster, "VISA resource name out"=w977:refnum<visa-resource-name>)  [unwired: 2 in]
        n529 = case shown="\"wait\"" w969 {
          tunnel: w964 -> [_ w985]
          tunnel: w977 -> [w984 w1001]
          tunnel: w976 -> [w983 w1000]
          tunnel: [w984 w990] -> w975
          tunnel: [w983 w997] -> w973
          tunnel: w967 -> [_ w996]
          frame "", Default {
          }
          frame "wait" {
            n530 = while {
              tunnel: w985 -> [w1010]
              shift-right: [w1007] -> w999
              shift-left: w1001 -> [w1009]
              shift-right: [w1006] -> w998
              shift-left: w1000 -> [w1008]
              stop <- w1005 stop-if-true
              n531 = call "Get Axis Motion Status.vi"("error in (no error)"=w1008, "Axis (1)"=w1010, "VISA resource name"=w1009) -> ("error out"=w1006:errorcluster, "Motion Done"=w1005:bool, "VISA resource name out"=w1007:refnum<visa-resource-name>)  [unwired: 2 in]
            }
            n532 = flat-sequence {
              tunnel: w999 -> [w1004]
              tunnel: w998 -> [w1003]
              tunnel: [w1004] -> w992
              tunnel: [w1003] -> w991
              frame #0 {
                n533 = Wait (ms)(milliseconds to wait=u32 1000) -> ()  [unwired: 1 out]
              }
            }
            n534 = local read "ESP_t0"() -> (w994:dbl)
            n535 = call "Read Actual Position.vi"("error in (no error)"=w991, "Axis (1)"=w985, "VISA resource name"=w992) -> ("error out"=w986:errorcluster, "Position (units)"=w988:dbl, "VISA resource name out"=w990:refnum<visa-resource-name>)  [unwired: 2 in]
            n536 = call "mm2time.vi"("fs?"=TRUE, "Offset (mm)"=w994, "distance (mm)"=w988) -> ("time in fs/ps seconds"=w989:dbl)
            n537 = call <vilib>:"Clear Errors.vi"("error in (no error)"=w986) -> ("error out"=w987:errorcluster)  [unwired: 5 in, 1 out]
            n538 = local write "ESP_pos"(w988) -> ()
            n539 = local write "ESP_delay"(w989) -> ()
            n540 = Send Notification(notification=TRUE, notifier=w996, error in (no error)=w987) -> (error out=w997:errorcluster)  [unwired: 1 out]
          }
        }
      }
      frame "suspend" {
        n541 = Dequeue Element(queue=w1014) -> ()  [unwired: 2 in, 4 out]
      }
      frame "release" {
        n542 = Dequeue Element(queue=w1017) -> (queue out=w1015:refnum<queue>)  [unwired: 2 in, 3 out]
        n543 = call "Close.vi"("VISA resource name"=w1020) -> ("error out"=w1019:errorcluster)  [unwired: 10 in]
        n544 = Enqueue Element(queue=w1015, element="suspend") -> ()  [unwired: 2 in, 3 out]
      }
      frame "close" {
        n545 = Release Queue(queue=w1024) -> ()  [unwired: 2 in, 3 out]
      }
      frame "init" {
        n546 = Dequeue Element(queue=w1029) -> ()  [unwired: 2 in, 4 out]
        n547 = flat-sequence {
          tunnel: [w1032] -> w1026
          tunnel: [w1031] -> w1025
          tunnel: [w1036] -> w1027
          tunnel: [w1037] -> w1028
          tunnel: w1026 -> [w1037]
          tunnel: w1025 -> [w1036]
          frame #0 {
            n548 = local write "ESP_con?"(FALSE ("ESP_con?")) -> ()
          }
          frame #1 {
            n549 = call "Initialize.vi"("VISA resource name"="ESP301 VISA", "Serial Link (RS232)"=enum16{"RS232", "USB"}."RS232") -> ("VISA resource name out"=w1032:refnum<visa-resource-name>, "error out"=w1031:errorcluster)  [unwired: 7 in]
          }
          frame #2 {
            n550 = local write "ESP_con?"(TRUE ("ESP_con?")) -> ()
          }
        }
      }
    }
    "error out" <- w925
  }
  n551 = while {
    tunnel: w18 -> [w1046]
    shift-right: [w1044] -> _
    shift-left: _ -> [w1042]
    shift-right: [w1043] -> _
    shift-left: _ -> [w1041]
    shift-right: [w1039] -> _
    shift-left: 0 -> [w1040]
    tunnel: w5 -> [w1038]
    stop <- w1045 stop-if-true
    # "manip"
    n552 = Preview Queue Element(queue=w1046, timeout in ms (-1)=w1040) -> (queue out=w1049:refnum<queue>, element=w1050:string)  [unwired: 1 in, 2 out]
    n553 = Match Pattern(string=w1050, regular expression=":") -> (before substring=w1048:string, after substring=w1047:string)  [unwired: 1 in, 2 out]
    n554 = case shown="\"init\"" w1048 {
      tunnel: w1049 -> [_ w1062 w1089 w1136 w1174 w1180 w1189 w1194]
      tunnel: w1047 -> [_ _ w1076 w1135 _ _ _ _]
      tunnel: [_ _ _ _ _ _ TRUE _] -> w1045
      tunnel: [w1056 w1064 w1068 w1133 w1176 refnum<k5> refnum ("gateway_connection out") w1187 w1193] -> w1044
      tunnel: [w1055 w1063 w1070 w1132 w1175 w1182 w1186 w1192] -> w1043
      tunnel: w1042 -> [w1058 w1066 w1092 w1126 w1176 w1184 w1187 _]
      tunnel: w1041 -> [w1057 w1065 w1091 w1127 w1175 _ w1186 _]
      tunnel: [_ _ _ _ -1 _ _ _] -> w1039
      tunnel: w1038 -> [_ _ w1067 w1129 _ _ _ _]
      frame "idle", Default {
        n555 = call "sp_manip_get_axis_status.vi"("error in"=w1057, "gateway_connection"=w1058) -> ("error out"=w1055:errorcluster, "axis_out"=w1054:T9, "gateway_connection out"=w1056:refnum<k5>)  [unwired: 5 in, 2 out]
        n556 = for {
          tunnel: w1054 -> [w1061] mode=indexing
          tunnel: [w1060] -> w1053 mode=indexing
          tunnel: [w1059] -> w1052 mode=indexing
          n557 = Unbundle By Name(w1061) -> ("Axis_Position"=w1060:dbl, "moving"=w1059:bool)
        }
        "moving?" <- w1052
        n558 = local write "pos"(w1053) -> ()
      }
      frame "stop" {
        n559 = Dequeue Element(queue=w1062) -> ()  [unwired: 2 in, 4 out]
        n560 = call "sp_manip_abort.vi"("error in"=w1065, "gateway_connection"=w1066) -> ("error out"=w1063:errorcluster, "gateway_connection out"=w1064:refnum<k5>)  [unwired: 6 in, 2 out]
      }
      frame "rel" {
        n561 = Dequeue Element(queue=w1089) -> ()  [unwired: 2 in, 4 out]
        n562 = Match Pattern(string=w1076, regular expression=":") -> (before substring=w1075:string, after substring=w1074:string)  [unwired: 1 in, 2 out]
        n563 = Equal?(x=w1074, y="wait") -> (x = y?=w1072:bool)
        n564 = call "sp_manip_get_axis_status.vi"("error in"=w1091, "gateway_connection"=w1092) -> ("error out"=w1094:errorcluster, "axis_out"=w1081:T9, "gateway_connection out"=w1093:refnum<k5>)  [unwired: 5 in, 2 out]
        n565 = Scan From String(format string="%g_%g_%g_%g_%g_%g", input string=w1075) -> (output 1=w1088:dbl, output 2=w1087:dbl, output 3=w1086:dbl, output 4=w1085:dbl, output 5=w1084:dbl, output 6=w1083:dbl)  [unwired: 8 in, 3 out]
        n566 = for {
          tunnel: w1081 -> [w1121] mode=indexing
          tunnel: [w1120] -> w1079 mode=indexing
          tunnel: [w1119] -> w1080 mode=indexing
          n567 = Unbundle By Name(w1121) -> ("Axis_Name"=w1120:string, "Axis_Position"=w1119:dbl)
        }
        n568 = Build Array(w1088, w1087, w1086, w1085, w1084, w1083) -> (w1082:dbl[])
        n569 = Add(x=w1080, y=w1082) -> (x+y=w1078:dbl[])
        n570 = call "sp_manip_start_move.vi"("error in"=w1094, "target positions"=w1078, "axis names"=w1079, "gateway_connection"=w1093) -> ("error out"=w1071:errorcluster, "gateway_connection out"=w1069:refnum<k5>)  [unwired: 4 in, 2 out]
        n571 = case shown="True" w1072 {
          tunnel: w1071 -> [w1095 w1106]
          tunnel: [w1095 w1105] -> w1070
          tunnel: w1069 -> [w1096 w1107]
          tunnel: [w1096 w1099] -> w1068
          tunnel: w1067 -> [_ w1104]
          frame False {
          }
          frame True {
            n572 = while {
              tunnel: w1107 -> [w1113]
              tunnel: w1106 -> [w1112]
              tunnel: [w1111] -> w1100
              tunnel: [w1110] -> w1098
              stop <- w1114 continue-if-true
              n573 = call "sp_manip_get_axis_status.vi"("error in"=w1112, "gateway_connection"=w1113) -> ("error out"=w1110:errorcluster, "axis_out"=w1116:T9, "gateway_connection out"=w1111:refnum<k5>)  [unwired: 5 in, 2 out]
              n574 = for {
                tunnel: w1116 -> [w1118] mode=indexing
                tunnel: [w1117] -> w1115 mode=indexing
                n575 = Unbundle By Name(w1118) -> ("moving"=w1117:bool)
              }
              n576 = Or Array Elements(Boolean array=w1115) -> (logical OR=w1114:bool)
            }
            n577 = call "sp_manip_get_axis_status.vi"("error in"=w1098, "gateway_connection"=w1100) -> ("error out"=w1097:errorcluster, "axis_out"=w1102:T9, "gateway_connection out"=w1099:refnum<k5>)  [unwired: 5 in, 2 out]
            n578 = for {
              tunnel: w1102 -> [w1109] mode=indexing
              tunnel: [w1108] -> w1101 mode=indexing
              n579 = Unbundle By Name(w1109) -> ("Axis_Position"=w1108:dbl)
            }
            n580 = Send Notification(notification=TRUE, notifier=w1104, error in (no error)=w1097) -> (error out=w1105:errorcluster)  [unwired: 1 out]
            n581 = local write "dest"(w1101) -> ()
          }
        }
      }
      frame "abs" {
        n582 = Dequeue Element(queue=w1136) -> ()  [unwired: 2 in, 4 out]
        n583 = call "sp_manip_get_axis_status.vi"("error in"=w1127, "gateway_connection"=w1126) -> ("error out"=w1122:errorcluster, "axis_out"=w1125:T9, "gateway_connection out"=w1123:refnum<k5>)  [unwired: 5 in, 2 out]
        n584 = Match Pattern(string=w1135, regular expression=":") -> (before substring=w1139:string, after substring=w1138:string)  [unwired: 1 in, 2 out]
        n585 = Equal?(x=w1138, y="wait") -> (x = y?=w1128:bool)
        n586 = for {
          tunnel: w1125 -> [w1149] mode=indexing
          tunnel: [w1148] -> w1124 mode=indexing
          n587 = Unbundle By Name(w1149) -> ("Axis_Name"=w1148:string)
        }
        n588 = Scan From String(format string="%g_%g_%g_%g_%g_%g", input string=w1139) -> (output 1=w1145:dbl, output 2=w1144:dbl, output 3=w1143:dbl, output 4=w1142:dbl, output 5=w1141:dbl, output 6=w1140:dbl)  [unwired: 8 in, 3 out]
        n589 = Build Array(w1145, w1144, w1143, w1142, w1141, w1140) -> (w1147:dbl[])
        n590 = call "sp_manip_start_move.vi"("error in"=w1122, "target positions"=w1147, "axis names"=w1124, "gateway_connection"=w1123) -> ("error out"=w1131:errorcluster, "gateway_connection out"=w1130:refnum<k5>)  [unwired: 4 in, 2 out]
        n591 = case shown="True" w1128 {
          tunnel: w1131 -> [w1150 w1161]
          tunnel: [w1150 w1160] -> w1132
          tunnel: w1130 -> [w1151 w1162]
          tunnel: [w1151 w1153] -> w1133
          tunnel: w1129 -> [_ w1159]
          frame False {
          }
          frame True {
            n592 = while {
              tunnel: w1162 -> [w1168]
              tunnel: w1161 -> [w1167]
              tunnel: [w1166] -> w1155
              tunnel: [w1165] -> w1154
              stop <- w1169 continue-if-true
              n593 = call "sp_manip_get_axis_status.vi"("error in"=w1167, "gateway_connection"=w1168) -> ("error out"=w1165:errorcluster, "axis_out"=w1171:T9, "gateway_connection out"=w1166:refnum<k5>)  [unwired: 5 in, 2 out]
              n594 = for {
                tunnel: w1171 -> [w1173] mode=indexing
                tunnel: [w1172] -> w1170 mode=indexing
                n595 = Unbundle By Name(w1173) -> ("moving"=w1172:bool)
              }
              n596 = Or Array Elements(Boolean array=w1170) -> (logical OR=w1169:bool)
            }
            n597 = call "sp_manip_get_axis_status.vi"("error in"=w1154, "gateway_connection"=w1155) -> ("error out"=w1152:errorcluster, "axis_out"=w1157:T9, "gateway_connection out"=w1153:refnum<k5>)  [unwired: 5 in, 2 out]
            n598 = for {
              tunnel: w1157 -> [w1164] mode=indexing
              tunnel: [w1163] -> w1156 mode=indexing
              n599 = Unbundle By Name(w1164) -> ("Axis_Position"=w1163:dbl)
            }
            n600 = local write "pos"(w1156) -> ()
            n601 = Send Notification(notification=TRUE, notifier=w1159, error in (no error)=w1152) -> (error out=w1160:errorcluster)  [unwired: 1 out]
          }
        }
      }
      frame "suspend" {
        n602 = Dequeue Element(queue=w1174) -> ()  [unwired: 2 in, 4 out]
      }
      frame "release" {
        n603 = Dequeue Element(queue=w1180) -> (queue out=w1178:refnum<queue>)  [unwired: 2 in, 3 out]
        n604 = call "sp_manip_disconnect.vi"("gateway_connection"=w1184) -> ("error out"=w1183:errorcluster, "gateway_connection_out"=w1185:refnum<k5>)  [unwired: 7 in, 2 out]
        n605 = call "tcp_gateway_close_connection.vi"("error in"=w1183, "server_connection"=w1185) -> ("error out"=w1182:errorcluster)  [unwired: 5 in]
        n606 = Enqueue Element(queue=w1178, element="suspend") -> ()  [unwired: 2 in, 3 out]
      }
      frame "close" {
        n607 = Release Queue(queue=w1189) -> ()  [unwired: 2 in, 3 out]
      }
      frame "init" {
        n608 = Dequeue Element(queue=w1194) -> ()  [unwired: 2 in, 4 out]
        n609 = flat-sequence {
          tunnel: [w1197] -> w1191
          tunnel: [w1196] -> w1190
          tunnel: [w1207] -> w1192
          tunnel: [w1208] -> w1193
          tunnel: w1191 -> [w1208]
          tunnel: w1190 -> [w1207]
          frame #0 {
            n610 = local write "manip_con?"(FALSE ("manip_con?")) -> ()
          }
          frame #1 {
            n611 = call "tcp_gateway_open_connection.vi"() -> ("gateway_connection"=w1200:refnum<k5>, "error out"=w1199:errorcluster)  [unwired: 5 in, 3 out]
            n612 = call "sp_manip_connect.vi"("error in"=w1199, "gateway_connection"=w1200) -> ("error out"=w1196:errorcluster, "axis_out"=w1198:T9, "gateway_connection out"=w1197:refnum<k5>)  [unwired: 5 in, 2 out]
            n613 = for {
              tunnel: w1198 -> [w1205] mode=indexing
              tunnel: [w1204] -> w1201 mode=indexing
              tunnel: [w1203] -> w1202 mode=indexing
              n614 = Unbundle By Name(w1205) -> ("Axis_Name"=w1204:string, "Axis_Position"=w1203:dbl)
            }
            "axis" <- w1201
            "pos" <- w1202
            n615 = local write "dest"(w1202) -> ()
          }
          frame #2 {
            n616 = local write "manip_con?"(TRUE ("manip_con?")) -> ()
          }
        }
      }
    }
    "error out 2" <- w1043
  }
  n617 = while {
    tunnel: w17 -> [w1220]
    shift-right: [w1209] -> _
    shift-left: 0 -> [w1218]
    shift-right: [w1217] -> _
    shift-left: _ -> [w1216]
    shift-right: [w1215] -> _
    shift-left: _ -> [w1214]
    shift-right: [w1213] -> _
    shift-left: u32 0 ("pHandle") -> [w1212]
    tunnel: w15 -> [w1211]
    tunnel: w5 -> [w1210]
    stop <- w1219 stop-if-true
    # "phoib"
    n618 = Preview Queue Element(queue=w1220, timeout in ms (-1)=w1218) -> (queue out=w1223:refnum<queue>, element=w1224:string)  [unwired: 1 in, 2 out]
    n619 = Match Pattern(string=w1224, regular expression=":") -> (before substring=w1222:string, after substring=w1221:string)  [unwired: 1 in, 2 out]
    n620 = case shown="\"idle\", Default" w1222 {
      tunnel: w1223 -> [_ w1281 w1336 w1353 w1371 w1385 w1390 w1395]
      tunnel: w1221 -> [_ _ w1332 _ _ _ _ _]
      tunnel: [_ _ _ _ _ TRUE _ _] -> w1219
      tunnel: [w1235 w1283 w1301 w1356 w1369 w1383 w1389 w1392] -> w1217
      tunnel: w1216 -> [w1246 w1272 w1322 w1358 w1370 w1383 w1389 _]
      tunnel: [w1234 w1282 w1317 w1355 w1368 w1381 w1387 w1391] -> w1215
      tunnel: w1214 -> [w1244 w1271 _ w1357 _ w1381 w1387 _]
      tunnel: [w1232 w1269 w1300 w1354 w1367 w1382 w1388 w1394] -> w1213
      tunnel: w1212 -> [w1232 w1269 w1320 w1354 w1366 w1382 w1388 _]
      tunnel: w1211 -> [w1233 w1262 w1298 _ _ _ _ _]
      tunnel: w1210 -> [_ _ w1316 _ _ _ _ _]
      tunnel: [_ _ _ _ _ _ -1 _] -> w1209
      frame "idle", Default {
        n621 = call "SL2_AD_DLL_Phoibos_GetDeviceState.vi"("dll_path"=w1246, "pHandle_in"=w1232, "dev_type"=DEF_dev_type."devA (analyzer)", "error in"=w1244) -> ("path out"=w1231:path, "state"=→"state":T3, "error out"=w1230:errorcluster)  [unwired: 2 in]
        n622 = for {
          tunnel: w1232 -> [w1253]
          tunnel: w1233 -> [w1251] mode=indexing
          tunnel: [w1250] -> w1243 mode=indexing
          tunnel: [w1249] -> w1235
          shift-right: [w1248] -> w1234
          shift-left: w1230 -> [w1252]
          tunnel: w1231 -> [w1247]
          n623 = call "SL2_AD_DLL_Phoibos_GetVoltage.vi"("error in"=w1252, "voltage_name"=w1251, "pHandle"=w1253, "dll path in"=w1247) -> ("error out"=w1248:errorcluster, "value"=w1250:dbl, "dll path out"=w1249:path)  [unwired: 3 in]
        }
        n624 = Index Array(array=w1243) -> (element #1=→"phoib_I_1":dbl, element #2=→"phoib_I_2":dbl, element #3=→"phoib_I_3":dbl, element #4=→"phoib_I_4":dbl, element #5=→"phoib_I_5":dbl, element #6=→"phoib_I_6":dbl, element #7=→"phoib_I_7":dbl, element #8=→"phoib_I_8":dbl, element #9=→"phoib_I_9":dbl, element #10=→"phoib_I_10":dbl)  [unwired: 10 in]
      }
      frame "set" {
        n625 = Dequeue Element(queue=w1281) -> ()  [unwired: 2 in, 4 out]
        n626 = Add(x=u32[] [251749632, 251749633, 251749634, 251749635, 251749636, 251749637, 251749638, 251749639, 251749640, 251749641, 251749642, 251749643, 251749644, 251749645, 251749646, 251749647, 251749648, 251749649, 251749650, 251749651, 251749652, 251749653, 251749654, 251749655, 251749656, 251749657, 251749658, 251749659, 251749660, 251749661, 251749662, 251749663, 251749664, 251749665, 251749666, 251749667, 251749668, 251749669, 251749670, 251749671, 251749672, 251749673, 251749674, 251749675, 251749676, 251749677, 251749678, 251749679, 251749680, 251749681, 251749682, 251749683, 251749684, 251749685, 251749686, 251749687, 251749688, 251749689, 251749690, 251749691, 251749692, 251749693, 251749694, 251749695, 251749696] ("modeIDs"), y=9984) -> (x+y=w1255:u32[])
        n627 = Multiply(x="ana_voltrange", y=12) -> (x*y=w1278:i32)
        n628 = Add(x="ana_mode", y=w1278) -> (x+y=w1275:i32)
        n629 = Index Array(array=w1255, index=w1275) -> (element=w1273:u32)
        n630 = Build Array("phoib_I_1s", "phoib_I_2s", "phoib_I_3s", "phoib_I_4s", "phoib_I_5s", "phoib_I_6s", "phoib_I_7s", "phoib_I_8s", "phoib_I_9s", "phoib_I_10s") -> (w1261:dbl[])
        n631 = call "SL2_AD_DLL_Phoibos_SetDeviceMode.vi"("pHandle"=w1269, "error in"=w1271, "value"=w1273, "dev_type"=DEF_dev_type."devA (analyzer)", "dll path in"=w1272) -> ("error out"=w1260:errorcluster, "dll path out"=w1270:path)  [unwired: 4 in]
        n632 = for {
          tunnel: w1269 -> [w1289]
          shift-right: [w1296] -> w1283
          shift-left: w1270 -> [w1293]
          tunnel: w1262 -> [w1288] mode=indexing
          tunnel: w1261 -> [w1287] mode=indexing
          shift-right: [w1295] -> w1282
          shift-left: w1260 -> [w1291]
          n633 = call "SL2_AD_DLL_Phoibos_GetVoltageRange.vi"("error in"=w1291, "voltage_name"=w1288, "pHandle"=w1289, "dll path in"=w1293) -> ("error out"=w1290:errorcluster, "min"=w1285:dbl, "max"=w1286:dbl, "dll path out"=w1292:path)  [unwired: 2 in]
          n634 = In Range and Coerce(upper limit=w1286, x=w1287, lower limit=w1285) -> (coerced(x)=w1284:dbl)  [unwired: 1 out]
          n635 = call "SL2_AD_DLL_Phoibos_SetVoltage.vi"("commit"=TRUE, "pHandle"=w1289, "error in"=w1290, "value"=w1284, "voltageName"=w1288, "dll path in"=w1292) -> ("error out"=w1295:errorcluster, "dll path out"=w1296:path)  [unwired: 3 in]
        }
      }
      frame "setsgl" {
        n636 = Dequeue Element(queue=w1336) -> ()  [unwired: 2 in, 4 out]
        n637 = Match Pattern(string=w1332, regular expression=":") -> (before substring=w1325:string, after substring=w1334:string)  [unwired: 1 in, 2 out]
        n638 = Equal?(x=w1334, y="wait") -> ()  [unwired: 1 out]
        n639 = Match Pattern(string=w1325, regular expression=":") -> (before substring=w1299:string, after substring=w1324:string)  [unwired: 1 in, 2 out]
        n640 = Fract/Exp String To Number(string=w1324) -> (number=w1323:dbl)  [unwired: 3 in, 1 out]
        n641 = call "SL2_AD_DLL_Phoibos_GetVoltageRange.vi"("voltage_name"=w1299, "pHandle"=w1320, "dll path in"=w1322) -> ("error out"=w1329:errorcluster, "min"=w1327:dbl, "max"=w1328:dbl, "dll path out"=w1330:path)  [unwired: 3 in]
        n642 = In Range and Coerce(upper limit=w1328, x=w1323, lower limit=w1327) -> (coerced(x)=w1318:dbl)  [unwired: 1 out]
        n643 = call "SL2_AD_DLL_Phoibos_SetVoltage.vi"("commit"=TRUE, "pHandle"=w1320, "error in"=w1329, "value"=w1318, "voltageName"=w1299, "dll path in"=w1330) -> ("error out"=w1319:errorcluster, "dll path out"=w1321:path)  [unwired: 3 in]
        n644 = while {
          tunnel: w1321 -> [w1352]
          tunnel: w1320 -> [w1346]
          tunnel: w1299 -> [w1351]
          tunnel: w1319 -> [w1350]
          tunnel: w1318 -> [w1349]
          tunnel: [w1346] -> w1300
          tunnel: [w1345] -> w1302
          tunnel: [w1344] -> w1304
          stop <- w1347 stop-if-true
          n645 = call "SL2_AD_DLL_Phoibos_GetVoltage.vi"("error in"=w1350, "voltage_name"=w1351, "pHandle"=w1346, "dll path in"=w1352) -> ("error out"=w1344:errorcluster, "value"=w1348:dbl, "dll path out"=w1345:path)  [unwired: 3 in]
          n646 = Equal?(x=w1349, y=w1348) -> (x = y?=w1347:bool)
        }
        n647 = for {
          tunnel: w1300 -> [w1343]
          tunnel: [w1341] -> w1305 mode=indexing
          tunnel: [w1340] -> w1301
          shift-right: [w1339] -> w1303
          shift-left: w1304 -> [w1342]
          tunnel: w1302 -> [w1338]
          tunnel: w1298 -> [w1337] mode=indexing
          n648 = call "SL2_AD_DLL_Phoibos_GetVoltage.vi"("error in"=w1342, "voltage_name"=w1337, "pHandle"=w1343, "dll path in"=w1338) -> ("error out"=w1339:errorcluster, "value"=w1341:dbl, "dll path out"=w1340:path)  [unwired: 3 in]
        }
        n649 = Index Array(array=w1305) -> (element #1=w1306:dbl, element #2=w1307:dbl, element #3=w1308:dbl, element #4=w1309:dbl, element #5=w1310:dbl, element #6=w1314:dbl, element #7=w1311:dbl, element #8=w1312:dbl, element #9=w1313:dbl, element #10=w1297:dbl)  [unwired: 10 in]
        n650 = local write "phoib_I_1"(w1306) -> ()
        n651 = local write "phoib_I_2"(w1307) -> ()
        n652 = local write "phoib_I_3"(w1308) -> ()
        n653 = local write "phoib_I_4"(w1309) -> ()
        n654 = local write "phoib_I_5"(w1310) -> ()
        n655 = local write "phoib_I_6"(w1314) -> ()
        n656 = local write "phoib_I_7"(w1311) -> ()
        n657 = local write "phoib_I_8"(w1312) -> ()
        n658 = local write "phoib_I_9"(w1313) -> ()
        n659 = local write "phoib_I_10"(w1297) -> ()
        n660 = Send Notification(notification=TRUE, notifier=w1316, error in (no error)=w1303) -> (error out=w1317:errorcluster)  [unwired: 1 out]
      }
      frame "standby" {
        w1359 = T3 0 items=["Off"=-1, "Standby"=0, "On"=1] ("state")
        n661 = Dequeue Element(queue=w1353) -> ()  [unwired: 2 in, 4 out]
        n662 = call "SL2_AD_DLL_Phoibos_SetDeviceState.vi"("pHandle_in"=w1354, "error in"=w1357, "state"=w1359, "dev_type"=DEF_dev_type."devA (analyzer)", "dll_path"=w1358) -> ("error out"=w1355:errorcluster, "path out"=w1356:path)  [unwired: 2 in]
      }
      frame "release" {
        n663 = Dequeue Element(queue=w1371) -> (queue out=w1361:refnum<queue>)  [unwired: 2 in, 3 out]
        n664 = flat-sequence {
          tunnel: w1370 -> [w1372]
          tunnel: w1366 -> [w1373]
          tunnel: [w1376] -> w1365
          tunnel: [w1375] -> w1364
          tunnel: [u32 0] -> w1363
          tunnel: [w1378] -> w1367
          tunnel: [w1379] -> w1368
          tunnel: [w1380] -> w1369
          tunnel: w1365 -> [w1380]
          tunnel: w1364 -> [w1379]
          tunnel: w1363 -> [w1378]
          frame #0 {
            n665 = call "SL2_AD_DLL_Phoibos_Shutdown.vi"("pHandle"=w1373, "dll path in"=w1372) -> ("error out"=w1375:errorcluster, "dll path out"=w1376:path)  [unwired: 4 in]
          }
          frame #1 {
            n666 = local write "phoib_con?"(FALSE ("phoib_con?")) -> ()
          }
        }
        n667 = Enqueue Element(queue=w1361, element="suspend") -> ()  [unwired: 2 in, 3 out]
      }
      frame "close" {
        n668 = Release Queue(queue=w1385) -> ()  [unwired: 2 in, 3 out]
      }
      frame "suspend" {
        n669 = Dequeue Element(queue=w1390) -> ()  [unwired: 2 in, 4 out]
      }
      frame "init" {
        n670 = Dequeue Element(queue=w1395) -> ()  [unwired: 2 in, 4 out]
        n671 = flat-sequence {
          tunnel: [w1402] -> w1393
          tunnel: [w1398] -> w1392
          tunnel: [w1397] -> w1391
          tunnel: [w1410] -> w1394
          tunnel: w1393 -> [w1410]
          frame #0 {
            n672 = local write "phoib_con?"(FALSE ("phoib_con?")) -> ()
          }
          frame #1 {
            w1401 = DEF_dev_type."devA (analyzer)" ("dev_type")
            n673 = call "GetSL2AD_VI_dllPath.vi"() -> ("error"=w1405:errorcluster, "Path"=w1406:path)  [unwired: 9 in, 1 out]
            n674 = call "SL2_AD_DLL_List_Devices.vi"("error in"=w1405, "dev_type"=w1401, "dll path in"=w1406) -> ("error out"=w1399:errorcluster, "devices"=w1408:string[], "dll path out"=w1400:path)  [unwired: 2 in]
            n675 = Index Array(array=w1408) -> (element=w1407:string)  [unwired: 1 in]
            n676 = call "SL2_AD_DLL_Phoibos_Initialize.vi"("error in"=w1399, "analyzerId"=w1407, "dll_path"=w1400) -> ("error out"=w1403:errorcluster, "pHandle"=w1402:u32, "path out"=w1404:path)  [unwired: 2 in]
            n677 = call "SL2_AD_DLL_Phoibos_ListDeviceModes.vi"("dll path in"=w1404, "dev_type"=w1401, "pHandle"=w1402, "error in"=w1403) -> ("dll path out"=w1398:path, "error out"=w1397:errorcluster)  [unwired: 1 in, 2 out]
          }
          frame #2 {
            n678 = local write "phoib_con?"(TRUE ("phoib_con?")) -> ()
          }
        }
      }
    }
    "phoib_error" <- w1215
  }
  n679 = while {
    tunnel: w1 -> [w1420]
    tunnel: w5 -> [w1414]
    shift-right: [w1413] -> _
    shift-left: 0 -> [w1412]
    stop <- w1411 stop-if-true
    # "temp"
    n680 = Preview Queue Element(queue=w1420, timeout in ms (-1)=w1412) -> (queue out=w1415:refnum<queue>, element=w1419:string)  [unwired: 1 in, 2 out]
    n681 = Match Pattern(string=w1419, regular expression=":") -> (before substring=w1418:string, after substring=w1417:string)  [unwired: 1 in, 2 out]
    n682 = case shown="\"ramp\"" w1418 {
      tunnel: w1417 -> [w1426 _ _ _ _]
      tunnel: w1415 -> [w1421 w1446 w1447 _ w1460]
      tunnel: w1414 -> [w1422 _ _ _ _]
      tunnel: [_ _ _ _ -1] -> w1413
      tunnel: [_ TRUE _ _ _] -> w1411
      frame "ramp" {
        n683 = Dequeue Element(queue=w1421) -> ()  [unwired: 2 in, 4 out]
        n684 = Match Pattern(string=w1426, regular expression=":") -> (before substring=w1425:string, after substring=w1429:string)  [unwired: 1 in, 2 out]
        n685 = Equal?(x=w1429, y="wait") -> (x = y?=w1423:bool)
        n686 = Scan From String(input string=w1425) -> (output 1=w1424:dbl)  [unwired: 4 in, 3 out]
        n687 = flat-sequence {
          tunnel: w1424 -> [w1431]
          tunnel: w1423 -> [w1433]
          tunnel: w1422 -> [w1443]
          frame #0 {
            n688 = local read "LS310  EPICS SP"() -> (w1430:string)
            n689 = call-poly <userlib>:"CaLabPut.vi"("Value"=w1431, "PV Name"=w1430) -> ()  [unwired: 6 in, 4 out]
          }
          frame #1 {
            n690 = Wait (ms)(milliseconds to wait=500) -> ()  [unwired: 1 out]
          }
          frame #2 {
            n691 = case shown="True" w1433 {
              frame False {
              }
              frame True {
                n692 = while {
                  stop <- w1439 stop-if-true
                  n693 = local read "Status EPICS chanel"() -> (w1441:string)
                  n694 = Wait (ms)(milliseconds to wait=500) -> ()  [unwired: 1 out]
                  n695 = call-poly <userlib>:"CaLabGet.vi"("PV Name"=w1441) -> ("1rst Value (string)"=w1442:string)  [unwired: 8 in, 6 out]
                  n696 = Equal?(x=w1442, y="Inside Range") -> (x = y?=w1439:bool)
                  n697 = local read "LS310  EPICS chanel A"() -> (w1435:string)
                  n698 = local read "LS310  EPICS chanel B"() -> (w1434:string)
                  n699 = call-poly <userlib>:"CaLabGet.vi"("PV Name"=w1435) -> ("1rst Value (number)"=w1436:dbl)  [unwired: 8 in, 6 out]
                  n700 = call-poly <userlib>:"CaLabGet.vi"("PV Name"=w1434) -> ("1rst Value (number)"=w1437:dbl)  [unwired: 8 in, 6 out]
                  n701 = local write "TB"(w1437) -> ()
                  n702 = local write "TA"(w1436) -> ()
                }
              }
            }
          }
          frame #3 {
            n703 = Send Notification(notification=TRUE, notifier=w1443) -> ()  [unwired: 1 in, 2 out]
          }
        }
      }
      frame "close" {
        n704 = Release Queue(queue=w1446) -> ()  [unwired: 2 in, 3 out]
      }
      frame "init" {
        n705 = Dequeue Element(queue=w1447) -> ()  [unwired: 2 in, 4 out]
      }
      frame "idle", Default {
        n706 = local read "LS310  EPICS chanel A"() -> (w1458:string)
        n707 = local read "LS310  EPICS chanel B"() -> (w1457:string)
        n708 = local read "LS310  EPICS SP"() -> (w1448:string)
        n709 = local read "Status EPICS chanel"() -> (w1456:string)
        n710 = local read "LS310  EPICS Heater"() -> (w1455:string)
        n711 = call-poly <userlib>:"CaLabGet.vi"("PV Name"=w1458) -> ("1rst Value (number)"=→"TA":dbl)  [unwired: 8 in, 6 out]
        n712 = call-poly <userlib>:"CaLabGet.vi"("PV Name"=w1457) -> ("1rst Value (number)"=→"TB":dbl)  [unwired: 8 in, 6 out]
        n713 = call-poly <userlib>:"CaLabGet.vi"("PV Name"=w1448) -> ("1rst Value (number)"=→"Readback":dbl)  [unwired: 8 in, 6 out]
        n714 = call-poly <userlib>:"CaLabGet.vi"("PV Name"=w1456) -> ("1rst Value (string)"=w1452:string)  [unwired: 8 in, 6 out]
        n715 = call-poly <userlib>:"CaLabGet.vi"("PV Name"=w1455) -> ()  [unwired: 8 in, 7 out]
        n716 = Equal?(x=w1452, y="Inside Range") -> (x = y?=→"In Range":bool)
      }
      frame "suspend" {
        n717 = Dequeue Element(queue=w1460) -> ()  [unwired: 2 in, 4 out]
      }
    }
  }
  n718 = while {
    tunnel: w20 -> [w1487]
    shift-right: [w1481] -> _
    shift-left: _ -> [w1480]
    shift-right: [w1479] -> _
    shift-left: _ -> [w1477]
    shift-right: [w1478] -> _
    shift-left: _ -> [w1476]
    shift-right: [w1473] -> _
    shift-left: 0 -> [w1474]
    shift-right: [w1472] -> _
    shift-left: _ -> [w1471]
    shift-right: [w1470] -> _
    shift-left: _ -> [w1469]
    tunnel: w29 -> [w1468]
    shift-right: [w1467] -> _
    shift-left: _ -> [w1466]
    shift-right: [w1464] -> _
    shift-left: _ -> [w1463]
    shift-right: [w1462] -> _
    shift-left: _ -> [w1461]
    i -> [w1465]
    stop <- w1475 stop-if-true
    # "cam"
    n719 = Preview Queue Element(queue=w1487, timeout in ms (-1)=w1474) -> (queue out=w1486:refnum<queue>, element=w1485:string)  [unwired: 1 in, 2 out]
    n720 = Match Pattern(string=w1485, regular expression=":") -> (before substring=w1482:string, after substring=w1483:string)  [unwired: 1 in, 2 out]
    n721 = case shown="\"idle\", Default" w1482 {
      tunnel: w1486 -> [w1499 w1531 w1564 w1577 _ w1665 w1695 w1760]
      tunnel: w1483 -> [_ _ _ _ _ _ _ _]
      tunnel: [w1493 w1518 w1563 w1575 w1618 w1662 w1680 w1758] -> w1481
      tunnel: w1480 -> [_ _ w1563 w1575 w1618 w1662 w1680 w1758]
      tunnel: [w1498 w1532 u64 0 ("Hout") w1574 w1622 w1663 w1690 w1757] -> w1479
      tunnel: [w1500 w1533 w1560 w1573 w1623 w1664 w1681 w1756] -> w1478
      tunnel: w1477 -> [_ w1535 w1562 w1574 w1625 w1667 w1692 w1757]
      tunnel: w1476 -> [_ w1534 _ w1573 w1624 w1666 w1691 w1756]
      tunnel: [_ _ _ TRUE _ _ _ _] -> w1475
      tunnel: [_ _ -1 _ _ _ _ -1] -> w1473
      tunnel: [w1492 w1519 _ _ w1632 _ _ _] -> w1472
      tunnel: w1471 -> [w1492 w1519 _ _ w1631 _ _ _]
      tunnel: [w1493 w1521 w1558 w1572 w1627 w1656 w1693 w1755] -> w1470
      tunnel: w1469 -> [_ w1521 w1558 w1572 w1627 _ w1693 w1755]
      tunnel: w1468 -> [_ _ _ _ _ _ w1684 _]
      tunnel: [w1490 w1516 w1557 w1570 w1585 w1653 w1687 w1754] -> w1467
      tunnel: w1466 -> [w1490 w1516 w1557 w1570 w1620 w1653 w1687 w1754]
      tunnel: w1465 -> [_ _ _ _ w1593 _ _ _]
      tunnel: [w1491 w1517 w1556 w1571 w1619 w1652 w1686 w1753] -> w1464
      tunnel: w1463 -> [w1491 w1517 w1556 w1571 w1592 w1652 w1686 w1753]
      tunnel: [w1489 w1513 refnum<k21> refnum ("task out") w1569 w1578 w1651 w1677 w1752] -> w1462
      tunnel: w1461 -> [_ w1513 w1555 w1569 w1578 w1651 w1678 w1752]
      frame "init" {
        w1493 = u16[][] []
        n722 = flat-sequence {
          tunnel: [w1502] -> w1497
          tunnel: [w1503] -> w1496
          tunnel: [w1511] -> w1498
          tunnel: [w1512] -> w1500
          tunnel: w1497 -> [w1512]
          tunnel: w1496 -> [w1511]
          frame #0 {
            n723 = local write "cam_con?"(FALSE ("cam_con?")) -> ()
          }
          frame #1 {
            n724 = call "SCInitBoard.vi"("boardnr"="board number") -> ("Hout"=w1506:u32, "error out"=w1507:errorcluster)  [unwired: 1 in, 1 out]
            n725 = call "SCSetupCamera.vi"("Handle"=w1506, "error in (no error)"=w1507) -> ("Hout"=w1508:u64, "error out"=w1509:errorcluster)  [unwired: 1 out]
            n726 = call "SCStopCOC.vi"("error in (no error)"=w1509, "Stop mode"=0, "Handle"=w1508) -> ("error out"=w1502:errorcluster, "Hout"=w1503:u64)
          }
          frame #2 {
            n727 = local write "cam_con?"(TRUE ("cam_con?")) -> ()
          }
        }
        n728 = Dequeue Element(queue=w1499) -> (queue out=w1495:refnum<queue>)  [unwired: 2 in, 3 out]
        n729 = Enqueue Element At Opposite End(queue=w1495, element="set") -> ()  [unwired: 2 in, 3 out]
        n730 = call-poly <vilib>:"DAQmx Create Virtual Channel.vi"("lines"=tag "Dev3/port0/line0") -> ("task out"=w1489:refnum<k21>)  [unwired: 13 in, 1 out]
      }
      frame "set" {
        n731 = Dequeue Element(queue=w1531) -> ()  [unwired: 2 in, 4 out]
        n732 = call "SCStopCOC.vi"("error in (no error)"=w1534, "Stop mode"=0, "Handle"=w1535) -> ("error out"=w1550:errorcluster, "Hout"=w1549:u64)
        n733 = Bundle By Name(cluster=cluster{"Delay":dbl, "Exposure ":dbl} {"Delay"=0.0, "Exposure "=0.0} ("Delay and exposure"), "Exposure"="cam_exp") -> (w1528:cluster{"Delay":dbl, "Exposure ":dbl})
        n734 = Bundle By Name(cluster=T11 {"Camera type"=0, "Operating mode\nHP & QE / HS & DiCam Pro "=0, "Frame trigger \n(High Performance and QE only)"=0, "Sequence trigger"=0, "Low Light\n(QE only)"=FALSE, "Gain"=FALSE, "Horzontal\nbinning"=0, "Vertical\nbinning "=0, "ROI Left"=1, "ROI Right"=20, "ROI Top"=1, "ROI Bottom"=15} ("Camera controls"), "Operating mode\nHP & QE / HS & DiCam Pro"="Operating mode\nHP & QE / HS & DiCam Pro", "Horzontal\nbinning"="binning", "Vertical\nbinning"="binning", "ROI Left"="ROI Left", "ROI Right"="ROI Right", "ROI Top"="ROI Top", "ROI Bottom"="ROI Bottom", "Gain"="gain", "Frame trigger \n(High Performance and QE only)"="Frame trigger \n(High Performance and QE only)") -> (w1545:T11)
        n735 = call "New delay and exposure forma.vi"("Operating mode\nHP & QE / HS & DiCam Pro"="Operating mode\nHP & QE / HS & DiCam Pro", "Delay and exposure"=w1528) -> ("Output table"=w1546:string)  [unwired: 3 in]
        n736 = call "SCSetCoC.vi"("error in (no error)"=w1550, "Delay and exposure table"=w1546, "Camera controls"=w1545, "Handle"=w1549) -> ("error out"=w1538:errorcluster, "Hout"=w1537:u64)  [unwired: 1 out]
        n737 = call "SCGetImageSize.vi"("Handle"=w1537, "error in (no error)"=w1538) -> ("Hout"=w1536:u64, "error out"=w1520:errorcluster, "Horizontal size"=w1525:i32, "Vertical size"=w1524:i32)  [unwired: 2 out]
        n738 = Greater?(x=w1525, y=w1524) -> (0:w1526:bool)
        n739 = Initialize Array(u16 0 ("dimension size"), w1524, w1525) -> (w1518:u16[][])
        n740 = call "SCRun.vi"("error in (no error)"=w1520, "Run mode"=0, "Handle"=w1536) -> ("error out"=w1533:errorcluster, "Hout"=w1532:u64)  [unwired: 1 out]
        n741 = Select(t=w1525, s=w1526, f=w1524) -> (s? t:f=w1523:i32)
        n742 = property on="mainimg" class="IntGraph (strict)"("XScale.Maximum"=w1523, "YScale.Maximum"=w1523) -> ()  [unwired: 2 in, 2 out]
      }
      frame "release" {
        n743 = Dequeue Element(queue=w1564) -> (queue out=w1551:refnum<queue>)  [unwired: 2 in, 3 out]
        n744 = flat-sequence {
          tunnel: w1562 -> [w1566]
          tunnel: [w1565] -> w1559
          tunnel: [w1568] -> w1560
          tunnel: w1559 -> [w1568]
          frame #0 {
            n745 = call "SCCloseBoard.vi"("Handle"=w1566) -> ("error out"=w1565:errorcluster)  [unwired: 1 in, 2 out]
          }
          frame #1 {
            n746 = local write "cam_con?"(FALSE ("cam_con?")) -> ()
          }
        }
        n747 = Enqueue Element(queue=w1551, element="suspend") -> ()  [unwired: 2 in, 3 out]
        n748 = call <vilib>:"DAQmx Clear Task.vi"("task in"=w1555) -> ()  [unwired: 14 in, 1 out]
      }
      frame "close" {
        n749 = Release Queue(queue=w1577) -> ()  [unwired: 2 in, 3 out]
      }
      frame "idle", Default {
        n750 = call "grabimg.vi"("array in"=w1618, "error in"=w1624, "Hin"=w1625) -> ("error out"=w1623:errorcluster, "imgdata"=w1621:i32[][], "Hout"=w1622:u64)  [unwired: 6 in]
        n751 = local read "lower threshold"() -> (w1616:i32)
        n752 = case shown="True" "cam_dark?" {
          tunnel: w1627 -> [_ w1650]
          tunnel: [w1647 w1649] -> w1617
          tunnel: w1621 -> [w1647 w1648]
          frame False {
          }
          frame True {
            n753 = Subtract(x=w1648, y=w1650) -> (x-y=w1649:dbl[][])
          }
        }
        n754 = call "filtr_b.vi"("threshold"=w1616, "input array"=w1617) -> ("output array"=w1608:dbl[][])  [unwired: 9 in]
        n755 = call <vilib>:"High Resolution Relative Seconds.vi"() -> ("relative seconds"=w1632:dbl)
        n756 = Subtract(x=w1632, y=w1631) -> (x-y=w1630:dbl)
        n757 = Array Size(array=w1608) -> (size(s)=w1607:i32[])
        n758 = Reciprocal(x=w1630) -> (1/x=→"cam_fps":dbl)
        n759 = Index Array(array=w1607) -> (element #1=w1602:i32, element #2=w1601:i32)  [unwired: 2 in]
        n760 = Subtract(x=w1593, y=w1592) -> (x-y=w1591:i32)
        n761 = Less Or Equal?(x="pics2avg", y=w1591) -> (x <= y?=w1614:bool)
        n762 = And(x="reset every n pics", y=w1614) -> (x .and. y?=w1612:bool)
        n763 = Not(x=w1612) -> (.not. x?=w1611:bool)
        n764 = call-poly <vilib>:"Ramp Pattern.vi"("start"=0.0, "end"=w1602, "samples"=w1602) -> ("Ramp Pattern"=w1597:dbl[])  [unwired: 7 in, 1 out]
        n765 = call-poly <vilib>:"Ramp Pattern.vi"("start"=0.0, "end"=w1601, "samples"=w1601) -> ("Ramp Pattern"=w1598:dbl[])  [unwired: 7 in, 1 out]
        n766 = property on="mainimg" class="IntGraph (strict)"() -> ("CrsrLis"=w1590:T5)  [unwired: 2 in, 2 out]
        n767 = And(x="cam_liveavg", y=w1611) -> (x .and. y?=w1609:bool)
        n768 = case shown="False" w1609 {
          tunnel: w1608 -> [w1637 w1643]
          tunnel: [w1637 w1640] -> w1585
          tunnel: w1620 -> [_ w1645]
          tunnel: w1593 -> [w1638 _]
          tunnel: [w1638 w1646] -> w1619
          tunnel: w1592 -> [_ w1646]
          tunnel: w1591 -> [_ w1639]
          frame False {
          }
          frame True {
            n769 = Multiply(x=w1645, y=w1639) -> (x*y=w1644:dbl[][])
            n770 = Increment(x=w1639) -> (x+1=w1641:i32)
            n771 = Add(x=w1644, y=w1643) -> (x+y=w1642:dbl[][])
            n772 = Divide(x=w1642, y=w1641) -> (x/y=w1640:dbl[][])
          }
        }
        "mainimg" <- w1585
        n773 = Index Array(array=w1590) -> (element #1=w1588:T12, element #2=w1589:T12)  [unwired: 2 in]
        n774 = Unbundle By Name(w1588) -> ("Position.X"=w1582:dbl, "Position.Y"=w1584:dbl)
        n775 = Unbundle By Name(w1589) -> ("Position.X"=w1586:dbl, "Position.Y"=w1587:dbl)
        n776 = Array Max & Min(array=w1585) -> (max value=→"max":dbl)  [unwired: 3 out]
        n777 = Subtract(x=w1587, y=w1584) -> (x-y=w1583:dbl)
        n778 = Subtract(x=w1586, y=w1582) -> (x-y=w1581:dbl)
        n779 = Array Subset(array=w1585, index (row)=w1584, length (row)=w1583) -> (w1596:dbl[][])  [unwired: 2 in]
        n780 = Array Subset(array=w1585, index (col)=w1582, length (col)=w1581) -> (w1594:dbl[][])  [unwired: 2 in]
        n781 = Array Subset(array=w1585, index (row)=w1584, length (row)=w1583, index (col)=w1582, length (col)=w1581) -> (w1580:dbl[][])
        n782 = Transpose 2D Array(2D array=w1596) -> (transposed array=w1595:dbl[][])
        n783 = Add Array Elements(numeric array=w1580) -> (sum=→"sum" →"Waveform Chart":dbl)
        n784 = for {
          tunnel: w1594 -> [w1634] mode=indexing
          tunnel: [w1633] -> w1604 mode=indexing
          n785 = Add Array Elements(numeric array=w1634) -> (sum=w1633:dbl)
        }
        n786 = for {
          tunnel: w1595 -> [w1636] mode=indexing
          tunnel: [w1635] -> w1603 mode=indexing
          n787 = Add Array Elements(numeric array=w1636) -> (sum=w1635:dbl)
        }
        n788 = Bundle("Ramp Pattern"=w1598, w1603) -> (→"G2 X":cluster{"Ramp Pattern":dbl[], dbl[]})  [unwired: 1 in]
        n789 = Bundle(w1604, "Ramp Pattern"=w1597) -> (→"G2 Y":cluster{dbl[], "Ramp Pattern":dbl[]})  [unwired: 1 in]
      }
      frame "dark" {
        n790 = Dequeue Element(queue=w1665) -> ()  [unwired: 2 in, 4 out]
        n791 = Array Size(array=w1662) -> (size(s)=w1661:i32[])
        n792 = Index Array(array=w1661) -> (element #1=w1660:i32, element #2=w1659:i32)  [unwired: 2 in]
        n793 = Initialize Array(0.0 ("element"), w1660, w1659) -> (w1657:dbl[][])
        n794 = for {
          N: "dark avg" -> [_]
          tunnel: w1667 -> [w1675]
          tunnel: w1666 -> [w1674]
          tunnel: [w1673] -> w1664
          tunnel: w1662 -> [w1672]
          tunnel: [w1671] -> w1663
          shift-right: [w1668] -> w1655
          shift-left: w1657 -> [w1669]
          n795 = call "grabimg.vi"("array in"=w1672, "error in"=w1674, "Hin"=w1675) -> ("error out"=w1673:errorcluster, "imgdata"=w1670:i32[][], "Hout"=w1671:u64)  [unwired: 6 in]
          n796 = Add(x=w1670, y=w1669) -> (x+y=w1668:dbl[][])
        }
        n797 = Divide(x=w1655, y="dark avg") -> (x/y=w1656:dbl[][])
      }
      frame "snap" {
        n798 = Dequeue Element(queue=w1695) -> ()  [unwired: 2 in, 4 out]
        n799 = local read "cam_dark?"() -> (w1694:bool)
        n800 = local read "cam_avgs"() -> (w1689:i32)
        n801 = To Double Precision Float(number=w1680) -> (double precision float=w1679:dbl[][])
        n802 = Equal To 0?(x="aq.mode") -> (x = 0?=w1682:bool)
        n803 = Get Date/Time In Seconds() -> (seconds since 1Jan1904=w1685:timestamp)
        n804 = for {
          N: w1689 -> [w1707]
          shift-right: [w1724] -> w1690
          shift-left: w1692 -> [w1726]
          shift-right: [w1712] -> w1688
          shift-left: w1691 -> [w1725]
          tunnel: w1694 -> [w1722]
          tunnel: w1693 -> [w1721]
          tunnel: w1680 -> [w1720]
          tunnel: w1685 -> [w1716]
          tunnel: w1682 -> [w1700]
          shift-right: [w1708] -> w1676
          shift-left: w1679 -> [w1709]
          shift-right: [w1698] -> w1677
          shift-left: w1678 -> [w1698]
          i -> [w1696]
          stop <- "abort acq." stop-if-true
          n805 = call "grabimg.vi"("array in"=w1720, "error in"=w1725, "Hin"=w1726) -> ("error out"=w1712:errorcluster, "imgdata"=w1723:i32[][], "Hout"=w1724:u64)  [unwired: 6 in]
          n806 = local read "lower threshold"() -> (w1703:i32)
          n807 = Increment(x=w1696) -> (x+1=w1705:i32)
          "acq. imgs" <- w1705
          n808 = Get Date/Time In Seconds() -> (seconds since 1Jan1904=w1719:timestamp)
          n809 = case shown="True" w1722 {
            tunnel: w1723 -> [w1748 w1751]
            tunnel: w1721 -> [_ w1750]
            tunnel: [w1748 w1749] -> w1702
            frame False {
            }
            frame True {
              n810 = Subtract(x=w1751, y=w1750) -> (x-y=w1749:dbl[][])
            }
          }
          n811 = Divide(x=w1705, y=w1707) -> (x/y=→"snap_prog":dbl)
          n812 = Subtract(x=w1719, y=w1716) -> (x-y=w1718:dbl)
          n813 = call "filtr_b.vi"("threshold"=w1703, "input array"=w1702) -> ("output array"=w1701:dbl[][])  [unwired: 9 in]
          n814 = Divide(x=w1718, y=w1696) -> (x/y=w1714:dbl)
          n815 = Multiply(x=w1714, y=w1707) -> (x*y=w1717:dbl)
          n816 = Reciprocal(x=w1714) -> (1/x=w1713:dbl)
          n817 = case shown="True" "count?" {
            tunnel: w1701 -> [w1739 w1741]
            tunnel: "e-size" -> [_ w1743]
            tunnel: w1703 -> [_ w1742]
            tunnel: [w1739 w1740] -> w1699
            frame False {
            }
            frame True {
              n818 = Array Size(array=w1741) -> (size(s)=w1745:i32[])
              n819 = call "findr.vi"("thresh"=w1742, "esize"=w1743, "inp array"=w1741) -> ("locs"=w1744:i32[][])  [unwired: 8 in]
              n820 = Index Array(array=w1745) -> (element #1=w1747:i32, element #2=w1746:i32)  [unwired: 2 in]
              n821 = call "drawe.vi"("Ysize"=w1747, "Xsize"=w1746, "pos array"=w1744) -> ("img out"=w1740:i32[][])  [unwired: 8 in]
            }
          }
          n822 = Add(x=w1717, y=w1716) -> (x+y=→"ETA":timestamp)
          n823 = local write "cam_fps"(w1713) -> ()
          n824 = local write "mainimg"(w1701) -> ()
          n825 = case shown="True" w1700 {
            tunnel: w1699 -> [w1729 w1737]
            tunnel: w1709 -> [w1731 w1736]
            tunnel: [w1730 w1734] -> w1708
            tunnel: [w1728 w1733] -> w1697
            tunnel: w1696 -> [w1727 w1732]
            frame False {
              n826 = Add(x=w1729, y=w1731) -> (x+y=w1730:dbl[][])
              n827 = Increment(x=w1727) -> (x+1=w1728:i32)
            }
            frame True {
              n828 = Multiply(x=w1736, y=w1732) -> (x*y=w1738:dbl[][])
              n829 = Increment(x=w1732) -> (x+1=w1733:i32)
              n830 = Add(x=w1737, y=w1738) -> (x+y=w1735:dbl[][])
              n831 = Divide(x=w1735, y=w1733) -> (x/y=w1734:dbl[][])
            }
          }
          "Pics L" <- w1697
          n832 = local write "sideimg"(w1708) -> ()
        }
        n833 = Enqueue Element(queue=w1684, element=w1676, error in (no error)=w1688) -> (error out=w1681:errorcluster)  [unwired: 1 in, 2 out]
      }
      frame "suspend" {
        n834 = Dequeue Element(queue=w1760) -> ()  [unwired: 2 in, 4 out]
      }
    }
    "cam_error" <- w1478
  }
